vi "DL-SMART-MS-Modify-06-23-7.0.vi"() -> ()   [LabVIEW 2013]
uses:
  <userlib>/caLab/Private/Put_DBL-1D_PV.vi
  <resource>/objmgr/imaqdx.rc
  <vilib>/Utility/file.llb/Write To Spreadsheet File (DBL).vi
  <userlib>/caLab/Private/Put_I32_PV.vi
  <userlib>/caLab/Private/Get_PV.vi
  <vilib>/Analysis/NI_AALPro.lvlib
  cal_p.vi
  <userlib>/caLab/Private/CaLabEvent_PV-1D.vi
  <vilib>/Utility/file.llb/Read From Spreadsheet File (DBL).vi
  <vilib>/Utility/config.llb/NI_LVConfig.lvlib
  <vilib>/Utility/config.llb/Write Key (Double).vi
  <vilib>/Utility/config.llb/Read Key (Double).vi
  <vilib>/Utility/config.llb/Write Key (U32).vi
  <vilib>/Utility/config.llb/Read Key (U32).vi
  <vilib>/Utility/config.llb/Write Key (String).vi
  <vilib>/Utility/config.llb/Read Key (String).vi
  <vilib>/Utility/config.llb/Config Data RefNum.ctl
panel:
  out "targetMark":string
  out "config":T1 caption="引用句柄"
  in  "stop":bool=TRUE
  out "LaserEnergy uJ 2":dbl
  out "idn status":string
  out "MS":cluster{dbl[], "filtered data":dbl[]}(graph)
  out "std sample":T2(array[cluster])
  out "Image":T3(plugin-control)
  out "selected id":i32
  out "selected row":i32
  out "currentNO":string
  out "commet":string
  out "sampleID":string
  in  "Shots/Point":i32=100
  in  "chamber in":bool caption="TakeMS"
  in  "chamber out":bool caption="TakeMS"
  in  "Laser parameter":T5
  in  "ADC parameter":T6
  in  "ShutDownSystem":bool
  in  "ADC reference":refnum<vi>
  in  "SetLaserTransmission":dbl(slide) min=0.0 max=50.0 scale=0.0..20.0
  in  "LaserHV":u8=50 min=1 max=100
  in  "频率/Hz":u8=30
  out "Pul.HV-Real":dbl
  out "Identify Spcetrum":cluster{"ID1:X":dbl[], "ID1:Y":dbl[]}[](graph)
  in  "测试记录":i32(listbox)=6
  in  "Identification Results (单靶鉴定结果)":i32(listbox)=2
  in  "HVEnable":bool
  out "GateClose":bool
  out "LaserOK":bool
  out "HV-OK":bool
  out "Vacuum-OK":bool
  in  "Tab Control":T7(tab)
  in  "helix-Zeta-Step":dbl=100.0
  in  "helix-b":dbl=0.2
  in  "AcquireMS-Methods":u8(ring) items=["SinglePoint", "Multipoints", "MultiTar"]
  in  "Thresh":dbl=-0.005 format="%#_13g"
  in  "right rank":i32=2
  in  "left rank":i32=2
  in  "deBaseline":bool
  in  "MCPHV-Set":dbl=1400.0 min=0.0 max=1600.0
  in  "LensHV-Set":dbl=8000.0 min=0.0 max=10000.0
  in  "Tar.HV-Set":dbl=18010.0 min=0.0 max=20000.0
  in  "Pul.HV-Set":dbl=1400.0 min=0.0 max=2000.0
  in  "PulseDelay":dbl
  in  "ADCFreq":dbl
  in  "CH1_Coupling":u64(ring)=2 items=["Volt DC"=1, "Volt AC"=2, "Ampere DC"=4, "Ampere AC"=8, "Ohm"=16]
  in  "Channel 1_Range":dbl(ring)=4.0 items=["80 V"=80.0, "40 V"=40.0, "20 V"=20.0, "8 V"=8.0, "4 V"=4.0, "2 V"=2.0, "800 mV"=0.8, "400 mV"=0.4, "200 mV"=0.2]
  in  "Anal. Setting File":string="High Mass"
  in  "SettingFileSave":bool caption="TakeMS"
  in  "SettingFileAppl":bool caption="TakeMS"
  in  "SettingDel":bool caption="TakeMS"
  in  "RunADC":bool caption="TakeMS"
  out "ADCstatus":bool
  in  "Vac_Prot.":bool
  in  "Turbo_Fore":bool
  in  "Main_Samp":bool
  in  "Samp_Atmos":bool
  in  "Fore_Samp":bool
  in  "StartPump":bool
  in  "SopPump":bool
  out "TurboSpeed":dbl(knob) scale=0.0..100.0
  out "PumpKW":dbl
  out "PumpAmps":dbl
  out "PumpTemp":u16
  out "PumpVolts":dbl
  in  "laser OFF":bool
  in  "laser ON":bool
  out "cluster":T8
  in  "laser Deactive":bool
  out "A1-position-Y":dbl=45.0 caption="Y" min=0.0 max=55.0
  out "A1-position-X":dbl=53.4 caption="X" min=0.0 max=55.0
  in  "GO":bool
  in  "Y":dbl min=0.0 max=55.0
  in  "X":dbl min=0.0 max=55.0
  in  "A1-Position":bool caption="X-"
  in  "Plat_To_Zero":bool caption="TakeMS"
  in  "Plat_Cal":bool caption="TakeMS"
  out "Y当前":dbl
  out "X当前":dbl
  out "移动":bool
  out "Y满":bool
  out "Y标":bool
  out "X满":bool
  out "Y0":bool
  out "X0":bool
  out "靶位In/Out":bool
  out "仓门":bool
  out "Y过热":bool
  out "X过热":bool
  out "通讯":bool
  in  "Operation Record":i32(listbox)
  in  "OptionRecordLoad 2":bool caption="TakeMS"
  in  "OptionRecordClear":bool caption="TakeMS"
  out "c:":dbl
  out "b:":dbl
  out "a:":dbl
  in  "cancel cal":bool
  in  "cal save":bool
  in  "peak cal":bool
  in  "peak detect":bool
  in  "标准样品":u16(ring) items=["肺炎克雷伯菌", "铜绿假单胞菌"]
  in  "定标参数":i32(listbox)
  out "Tar.HV-Real":dbl
  out "LensHV-Real":dbl
  out "MCPHV-Real":dbl
  out "Lvaccum":dbl=0.83 format="%#_2e"
  out "Hvaccum":dbl=3.4e-05 format="%#_2e"
  in  "H12":bool
  in  "G12":bool
  in  "F12":bool
  in  "E12":bool
  in  "D12":bool
  in  "C12":bool
  in  "B12":bool
  in  "A12":bool
  in  "H11":bool
  in  "G11":bool
  in  "F11":bool
  in  "E11":bool
  in  "D11":bool
  in  "C11":bool
  in  "B11":bool
  in  "A11":bool
  in  "H10":bool
  in  "G10":bool
  in  "F10":bool
  in  "E10":bool
  in  "D10":bool
  in  "C10":bool
  in  "B10":bool
  in  "A10":bool
  in  "H9":bool
  in  "G9":bool
  in  "F9":bool
  in  "E9":bool
  in  "D9":bool
  in  "C9":bool
  in  "B9":bool
  in  "A9":bool
  in  "H8":bool
  in  "G8":bool
  in  "F8":bool
  in  "E8":bool
  in  "D8":bool
  in  "C8":bool
  in  "B8":bool
  in  "A8":bool
  in  "H7":bool
  in  "G7":bool
  in  "F7":bool
  in  "E7":bool
  in  "D7":bool
  in  "C7":bool
  in  "B7":bool
  in  "A7":bool
  in  "H6":bool
  in  "G6":bool
  in  "F6":bool
  in  "E6":bool
  in  "D6":bool
  in  "C6":bool
  in  "B6":bool
  in  "A6":bool
  in  "H5":bool
  in  "G5":bool
  in  "F5":bool
  in  "E5":bool
  in  "D5":bool
  in  "C5":bool
  in  "B5":bool
  in  "A5":bool
  in  "H4":bool
  in  "G4":bool
  in  "F4":bool
  in  "E4":bool
  in  "D4":bool
  in  "C4":bool
  in  "B4":bool
  in  "A4":bool
  in  "H3":bool
  in  "G3":bool
  in  "F3":bool
  in  "E3":bool
  in  "D3":bool
  in  "C3":bool
  in  "B3":bool
  in  "A3":bool
  in  "H2":bool
  in  "G2":bool
  in  "F2":bool
  in  "E2":bool
  in  "D2":bool
  in  "C2":bool
  in  "B2":bool
  in  "A2":bool
  in  "H1":bool
  in  "G1":bool
  in  "F1":bool
  in  "E1":bool
  in  "D1":bool
  in  "C1":bool
  in  "B1":bool
  in  "A1":bool
  in  "Clear":bool caption="TakeMS"
  in  "Add":bool caption="TakeMS"
  in  "TakeMS-Stop":bool caption="TakeMS"
  in  "TakeMS-Run":bool caption="TakeMS"
  # "Laser (激光)"
  # "光栅"
  # "uJ"
  # "Acq.(采谱)"
  # "Vacuum(真空)"
  # "1"
  # "2"
  # "3"
  # "4"
  # "5"
  # "6"
  # "7"
  # "8"
  # "9"
  # "10"
  # "11"
  # "12"
  # "A"
  # "Pa"
  # "High"
  # "B"
  # "Low"
  # "Pa"
  # "C"
  # "H.V.(高压)"
  # "D"
  # "MCP"
  # "V"
  # "E"
  # "Tar."
  # "V"
  # "F"
  # "Pul."
  # "V"
  # "G"
  # "Lens"
  # "V"
  # "H"
  # "Vauum (真空)"
  # "H.V. (高压)"
  # "Laser (激光)"
  # "Gate (仓门)"
  # "mm"
  # "Radian"
  # "H.V. (高压参数)"
  # "ADC(采集卡设置)"
  # "ADCFreq(采样)"
  # "MCP (探测器)"
  # "V"
  # "Hz"
  # "Tar. (靶)"
  # "V"
  # "Setting File(设置文件)"
  # "Coupling"
  # "Pulse (脉冲)"
  # "V"
  # "IntRange"
  # "V"
  # "Lens (透镜)"
  # "Delay (延时)"
  # "ns"
  # "Sole. Valves"
  # "Turbo Pump"
  # "自锁保护"
  # "机械/分子"
  # "主仓/样仓"
  # "样仓/大气"
  # "机械/样仓"
  # "激光器状态"
  # "mm"
  # "mm"
  # "mm"
  # "mm"
  # "mm"
  # "mm"
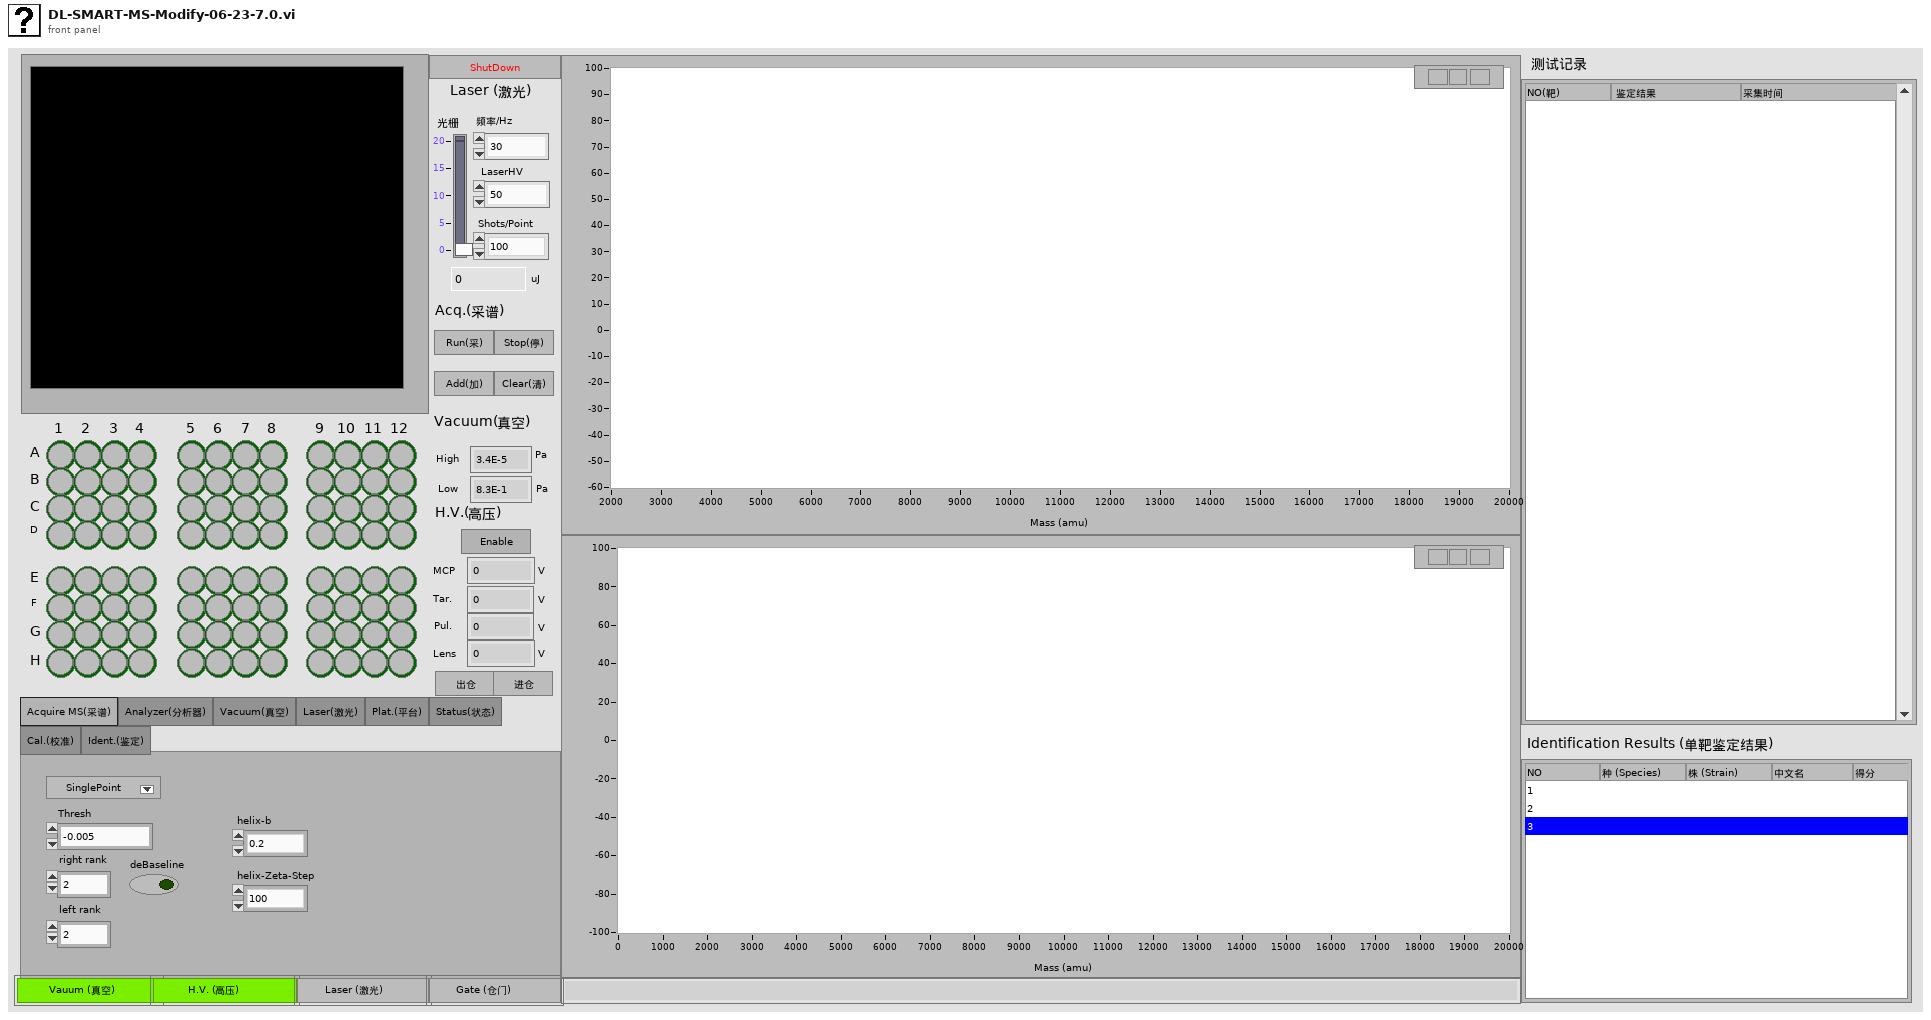
[diagram p1: front panel]
types:
  T1 = typedef "NI_LVConfig.lvlib/Config Data RefNum.ctl" = refnum<k1>
  T2 = cluster{"name":string, "mz":dbl[], "time":dbl[]}[]
  T3 = typedef "IMAQ Image.ctl" = refnum<image>
  T4 = typedef "Semaphore RefNum" = refnum<k1>
  T5 = cluster{"VISA resource name":refnum<visa-resource-name>, "standby":bool, "semaphore in":T4, "SetLaserEnergy":dbl}
  T6 = cluster{"TpDeviceHandle_t":u32, "Record Length/Samples":u64, "ShotsPerPoint":u16}
  T7 = enum32{"Acquire MS(采谱)", "Analyzer(分析器)", "Vacuum(真空)", "Laser(激光)", "Plat.(平台)", "Status(状态)", "Cal.(校准)", "Ident.(鉴定)"}
  T8 = cluster{"链接":bool, "待机":bool, "发射":bool, "[3]":bool, "内存":bool, "测能":bool, "温警":bool, "静态":bool, "操作":bool}
  T9 = cluster{"tag1":string, "tag2":string, "x":dbl[], "y":dbl[], "ID1:X":dbl[], "ID1:Y":dbl[], "ID1:REF:X":dbl[], "ID1:REF:Y":dbl[], "ID2:X":dbl[], "ID2:Y":dbl[], "ID2:REF:X":dbl[], "ID2:REF:Y":dbl[], "ID3:X":dbl[], "ID3:Y":dbl[], "ID3:REF:X":dbl[], "ID3:REF:Y":dbl[], "ID1:TAG1":string, "ID1:TAG2":string, "ID2:TAG1":string, "ID2:TAG2":string, "ID3:TAG1":string, "ID3:TAG2":string, "ID1:NAME":string, "ID2:NAME":string, "ID3:NAME":string, "ID1:SCORE":string, "ID2:SCORE":string, "ID3:SCORE":string, "NO":string}[]
  T10 = cluster{"laser semaphore":T4, "pump semaphore":T4}
  T11 = enum8{"Enabled", "Disabled", "Disabled and Grayed Out"}
  T12 = cluster{"tag1":string, "tag2":string, "x":dbl[], "y":dbl[], "ID1:X":dbl[], "ID1:Y":dbl[], "ID1:REF:X":dbl[], "ID1:REF:Y":dbl[], "ID2:X":dbl[], "ID2:Y":dbl[], "ID2:REF:X":dbl[], "ID2:REF:Y":dbl[], "ID3:X":dbl[], "ID3:Y":dbl[], "ID3:REF:X":dbl[], "ID3:REF:Y":dbl[], "ID1:TAG1":string, "ID1:TAG2":string, "ID2:TAG1":string, "ID2:TAG2":string, "ID3:TAG1":string, "ID3:TAG2":string, "ID1:NAME":string, "ID2:NAME":string, "ID3:NAME":string, "ID1:SCORE":string, "ID2:SCORE":string, "ID3:SCORE":string, "NO":string}
  T13 = cluster{"monitor":refnum<user-event>, "motor status":refnum<user-event>, "motor":refnum<user-event>, "notifier out":refnum<notifier>, "queue out":refnum<queue>, "AI":T4, "DI":T4, "CX":T4, "CY":T4}
  T14 = cluster{"AI Task":refnum<k21>, "AO Task":refnum<k21>, "DO Task":refnum<k21>, "DI Task":refnum<k21>, "PWM x":refnum<k21>, "PWM y":refnum<k21>, "counter x":refnum<k21>, "counter y":refnum<k21>}
  T15 = cluster{"tasks":cluster{"AI Task":refnum<k21>, "AO Task":refnum<k21>, "DO Task":refnum<k21>, "DI Task":refnum<k21>, "PWM x":refnum<k21>, "PWM y":refnum<k21>, "counter x":refnum<k21>, "counter y":refnum<k21>}, "interface":cluster{"monitor":refnum<user-event>, "motor status":refnum<user-event>, "motor":refnum<user-event>, "notifier out":refnum<notifier>, "queue out":refnum<queue>, "AI":T4, "DI":T4, "CX":T4, "CY":T4}, "error out":errorcluster}
  T16 = cluster{"ConfiguredPumpCom":refnum<visa-resource-name>, "ConfiguredLaserCom":refnum<visa-resource-name>}
  T17 = typedef "LVPoint32TypeDef.ctl" = cluster{"Horizontal":i32, "Vertical":i32}
  T18 = typedef "LVRowAndColumnTypeDef.ctl" = cluster{"Row":i32, "Column":i32}
  T19 = cluster{"Type":u32, "Version":u32, "Flags":u32, "SerialNumberHigh":u32, "SerialNumberLow":u32, "BusType":u32, "InterfaceName":string, "VendorName":string, "ModelName":string, "CameraFileName":string, "CameraAttributeURL":string}[]
  T20 = cluster{"Type":u32, "Version":u32, "Flags":u32, "SerialNumberHigh":u32, "SerialNumberLow":u32, "BusType":u32, "InterfaceName":string, "VendorName":string, "ModelName":string, "CameraFileName":string, "CameraAttributeURL":string}
  T21 = typedef "IMAQdx.ctl" = refnum<k21>
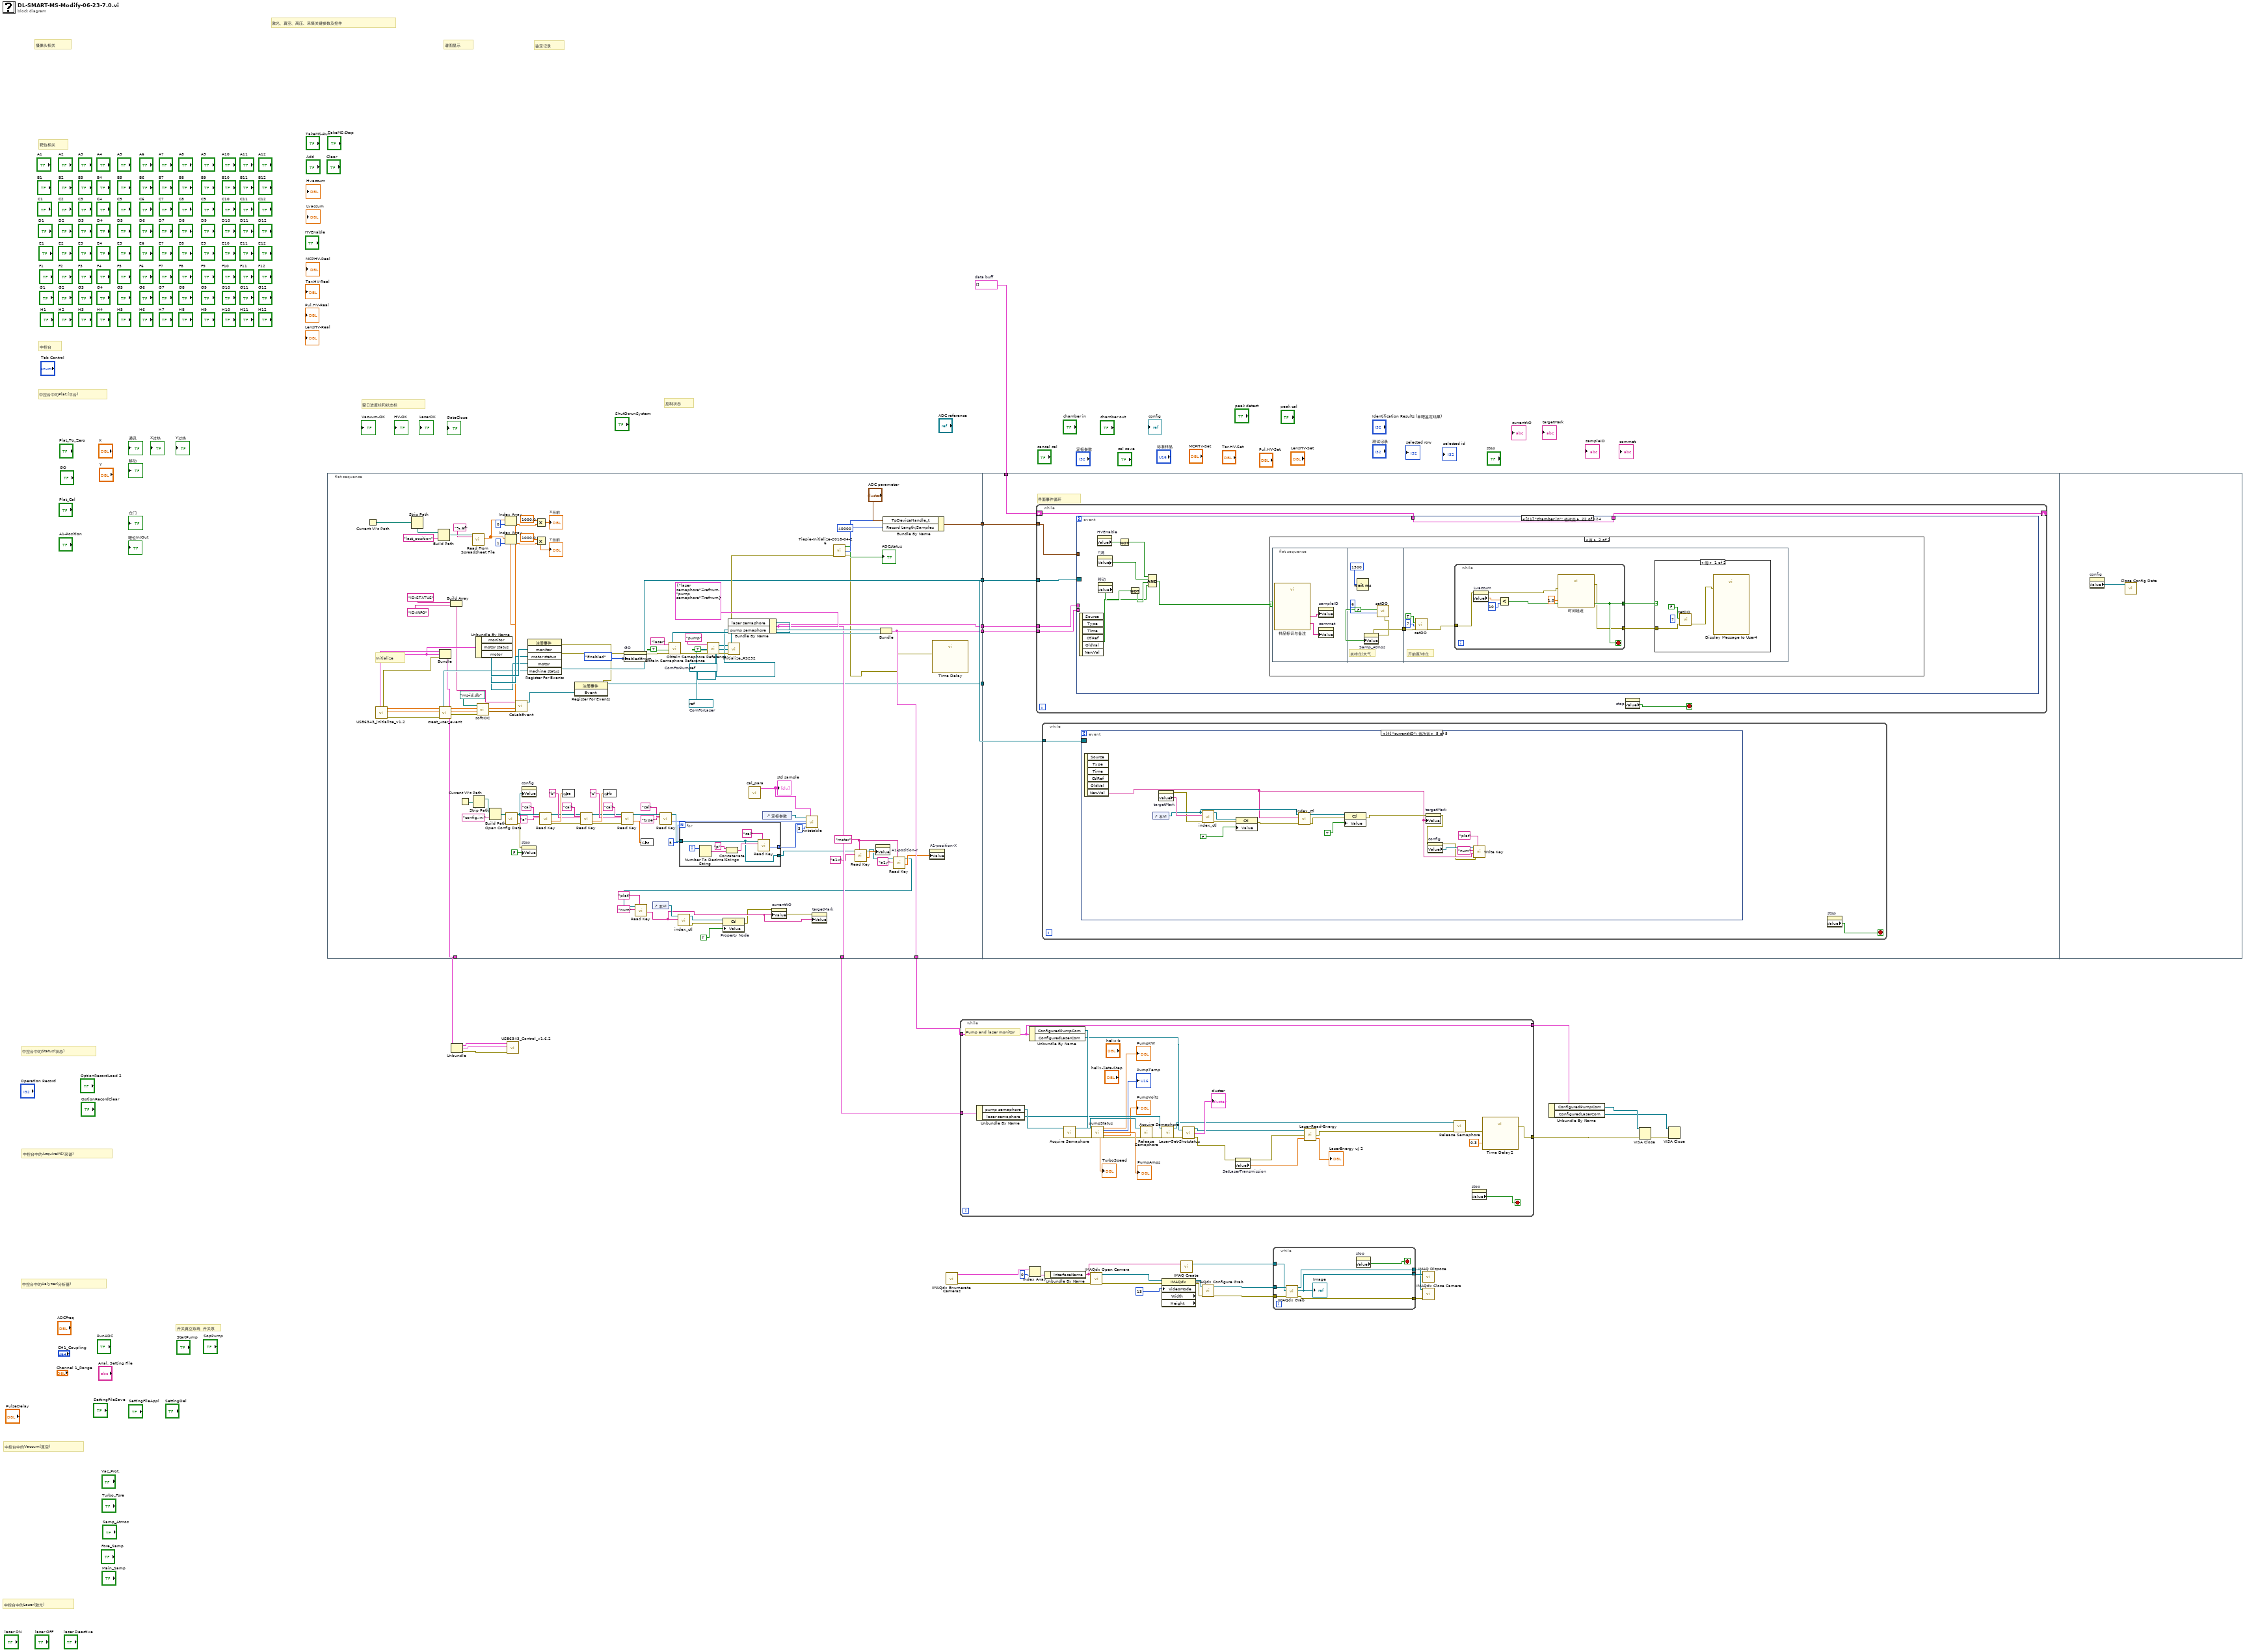
[diagram p0: block diagram]
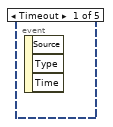
[diagram p2: hidden frame]
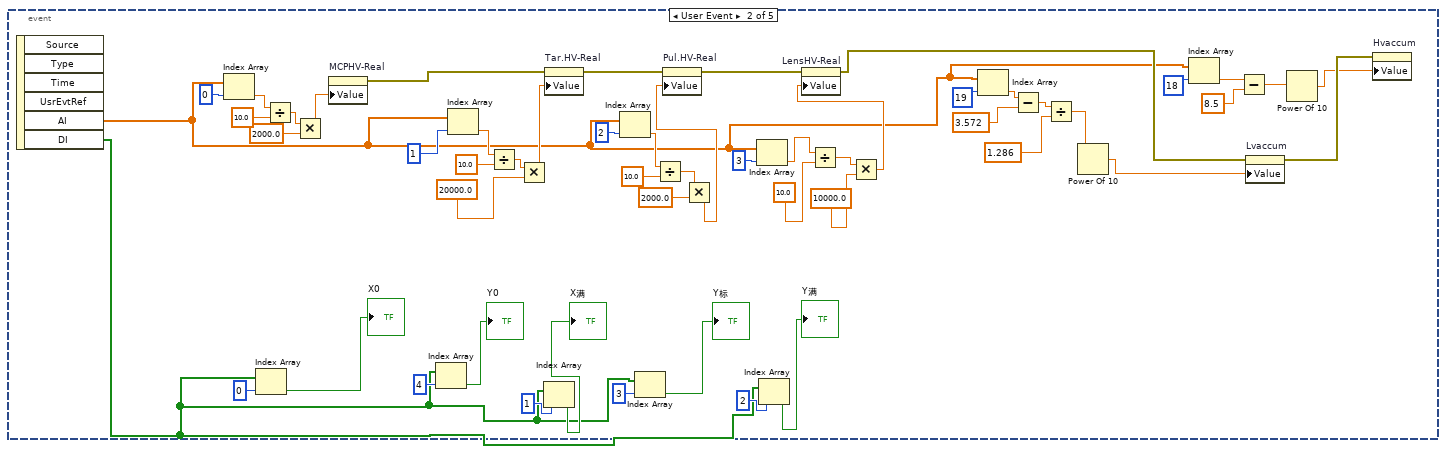
[diagram p3: hidden frame]
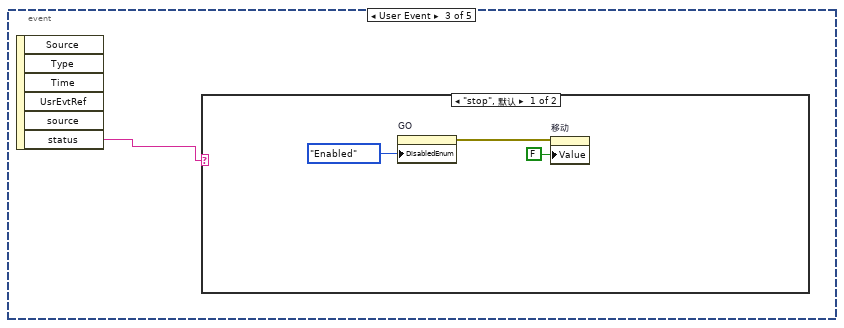
[diagram p4: hidden frame]
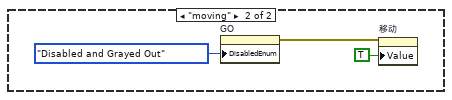
[diagram p5: hidden frame]
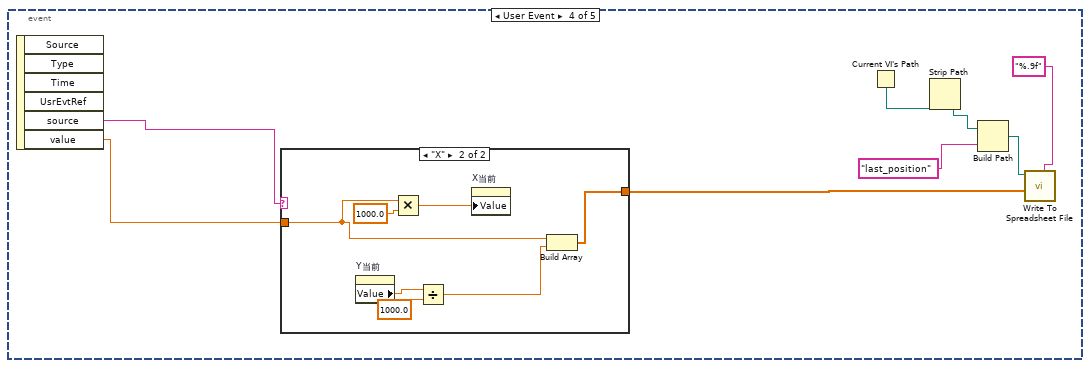
[diagram p6: hidden frame]
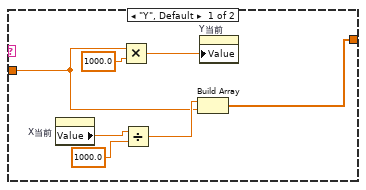
[diagram p7: hidden frame]
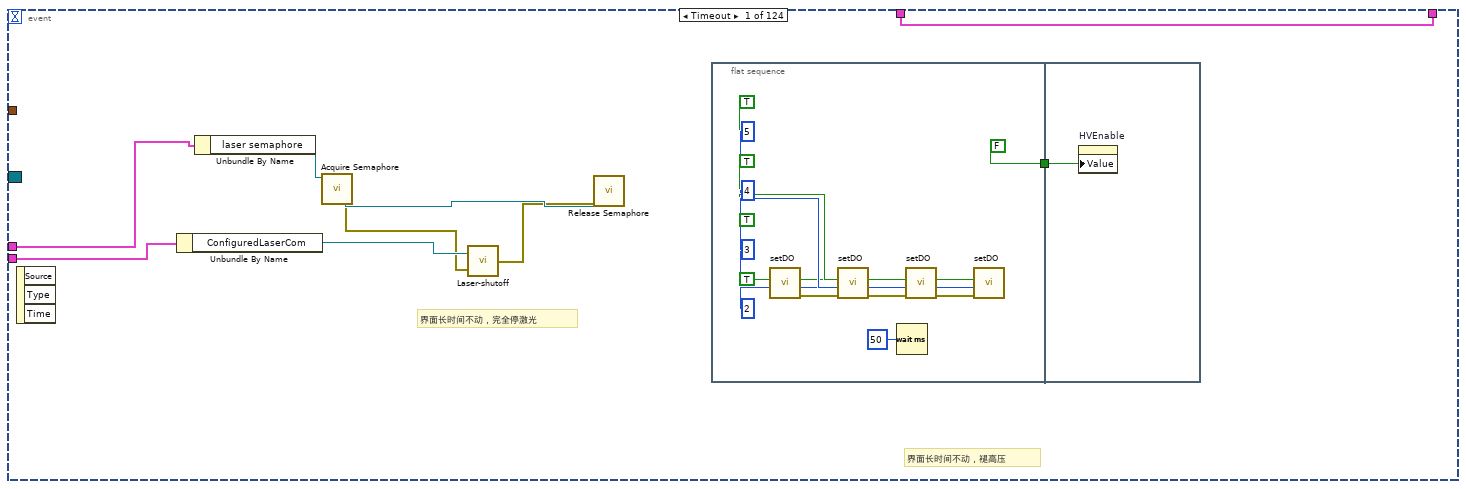
[diagram p8: hidden frame]
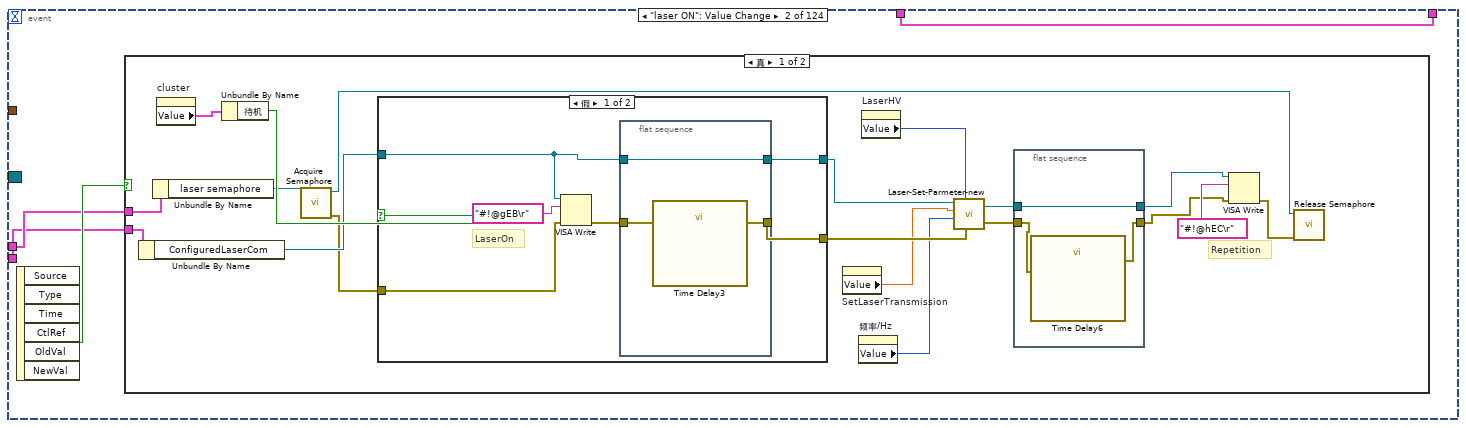
[diagram p9: hidden frame]
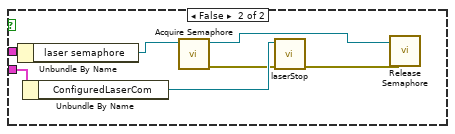
[diagram p11: hidden frame]
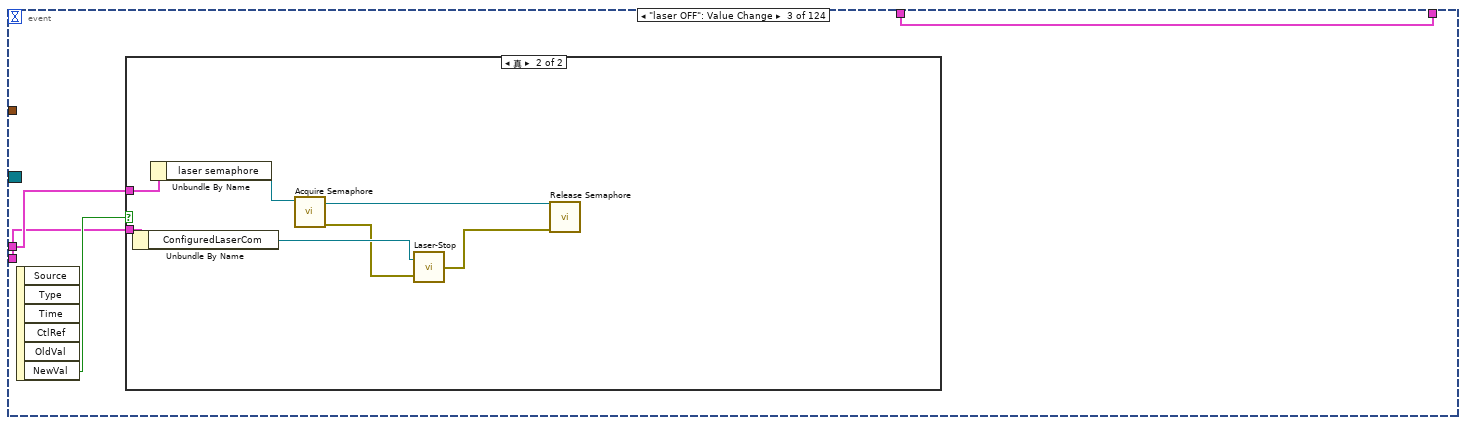
[diagram p12: hidden frame]
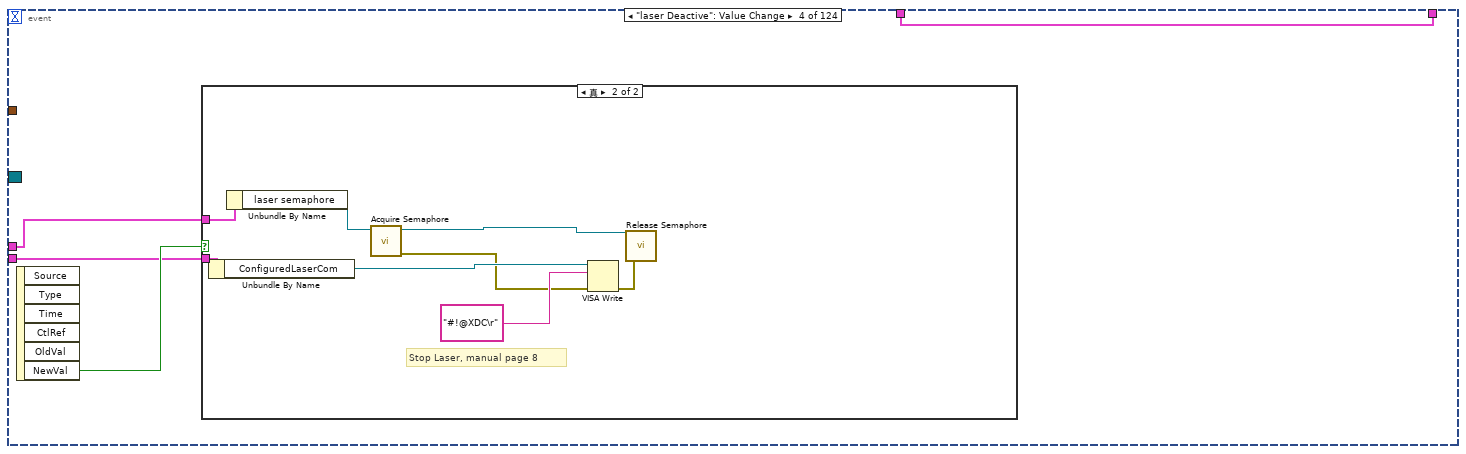
[diagram p14: hidden frame]
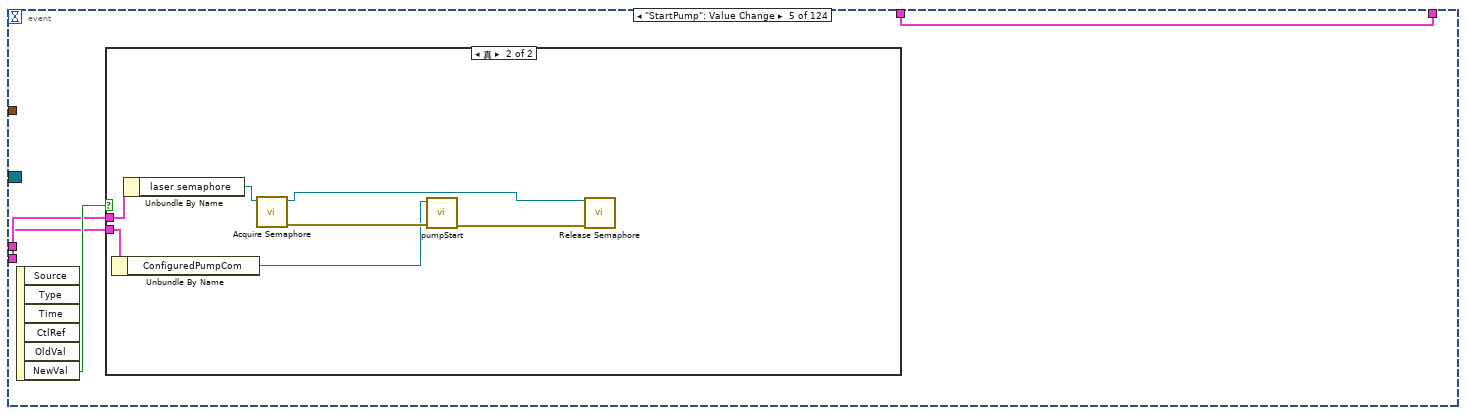
[diagram p16: hidden frame]
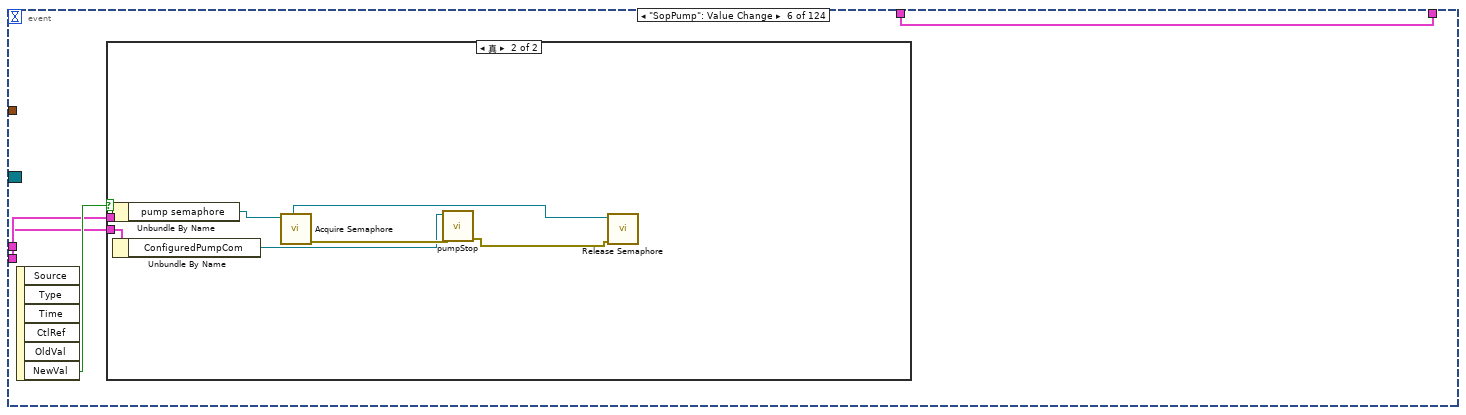
[diagram p18: hidden frame]
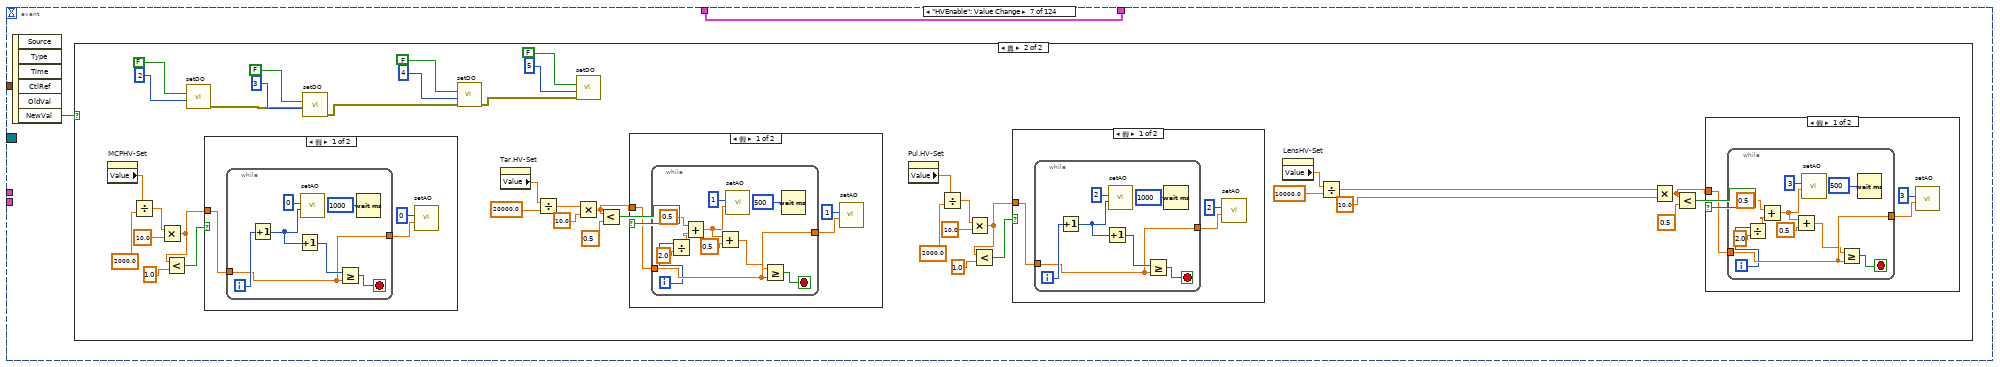
[diagram p20: hidden frame]
diagram:
  w26 = T9 []  # data buff
  # "Pump and laser monitor"
  # "开关真空系统  开关泵"
  # "控制状态"
  # "鉴定记录"
  # "谱图显示"
  # "激光、真空、高压、采集关键参数及控件"
  # "窗口进度栏和状态栏"
  # "中控台中的Laser(激光)"
  # "中控台中的Vaccum(真空)"
  # "中控台中的Aalyzer(分析器)"
  # "中控台中的AcquireMS(采谱)"
  # "中控台中的Status(状态)"
  # "中控台中的Plat.(平台)"
  # "中控台"
  # "靶位相关"
  # "摄像头相关"
  n1 = flat-sequence {
    tunnel: [w91] -> w33
    tunnel: [w116] -> w32
    tunnel: [w116] -> w30
    tunnel: [w115] -> w31
    tunnel: [w115] -> w29
    tunnel: [w119] -> w28
    tunnel: [w108] -> w27
    tunnel: [w79] -> w6
    tunnel: w33 -> [w146]
    tunnel: w32 -> [w150]
    tunnel: w31 -> [w149]
    tunnel: w27 -> [w148]
    tunnel: w26 -> [w147]
    tunnel: w6 -> [w145]
    frame #0 {
      w46 = "motor" ("section")
      w113 = refnum<visa-resource-name> "COM9"  # ComForLaser
      w114 = refnum<visa-resource-name> "COM10"  # ComForPump
      # "Initialize"
      n2 = Current VI's Path() -> (path=w106:path)
      n3 = Strip Path(path=w106) -> (stripped path=w105:path)  [unwired: 1 out]
      n4 = Build Path(base path=w105, name or relative path="last_position") -> (appended path=w103:path)
      n5 = Build Array("ID:STATUS", "ID:INFO") -> (w81:string[])
      n6 = Current VI's Path() -> (path=w76:path)
      n7 = call-poly <vilib>:"Read From Spreadsheet File.vi"("format (%.3f)"="%.6f", "file path (dialog if empty)"=w103) -> ("first row"=w101:dbl[])  [unwired: 5 in, 4 out]
      n8 = Strip Path(path=w76) -> (stripped path=w75:path)  [unwired: 1 out]
      n9 = Build Path(base path=w75, name or relative path="config.ini" ("名称或相对路径")) -> (appended path=w73:path)
      n10 = Index Array(array=w101, index=0) -> (element=w98:dbl)
      n11 = Index Array(array=w101, index=1) -> (element=w95:dbl)
      n12 = call "USB6343_initialize_v1.2.vi"("Y initial position"=w95, "X initial position"=w98) -> ("error out"=w120:errorcluster, "interface"=w121:T13, "tasks"=w122:T14)  [unwired: 7 in]
      n13 = Bundle("tasks"=w122, "interface"=w121, "error out"=w120) -> (w119:T15)  [unwired: 1 in]
      n14 = call "creat_user_event.vi"("error in (no error)"=w120) -> ("error out"=w88:errorcluster, "machine status"=w130:refnum<user-event>)  [unwired: 9 in]
      n15 = Unbundle By Name(w121) -> ("monitor"=w137:refnum<user-event>, "motor status"=w136:refnum<user-event>, "motor"=w135:refnum<user-event>)
      n16 = call "softIOC.vi"("error in (no error)"=w88, "路径"=path "ms-id.db") -> ("error out"=w89:errorcluster)  [unwired: 8 in, 1 out]
      n17 = call <vilib>:"Open Config Data.vi"("configuration file path"=w73) -> ("error out"=w72:errorcluster, "refnum"=w71:T1)  [unwired: 8 in, 1 out]
      n18 = call-poly <userlib>:"CaLabEvent.vi"("error in (no error)"=w89, "PV Names"=w81) -> ("Event"=w80:refnum<user-event>)  [unwired: 7 in, 2 out]
      n19 = property on="config" class="TypRef (严格)"("Value"=w71) -> ()  [unwired: 2 in, 2 out]
      n20 = property on="stop" class="Bool (严格)"(error in=w72, "Value"=FALSE ("ShutDownSystem")) -> ()  [unwired: 1 in, 2 out]
      n21 = Multiply(x=1000.0, y=w98) -> (x*y=→"X当前":dbl)
      n22 = Multiply(x=1000.0, y=w95) -> (x*y=→"Y当前":dbl)
      n23 = call-poly <vilib>:"Read Key.vi"("section"="cal", "key"="a", "refnum"=w71) -> ("error out"=w63:errorcluster, "value"=w68:dbl, "refnum out"=w64:T1)  [unwired: 5 in, 1 out]
      n24 = global write "cal_p.vi" "a"(w68) -> ()
      n25 = register-events(w80) -> (reference out=w79:refnum<event-registration>, error out=w78:errorcluster)  [unwired: 2 in]
      n26 = register-events(error in=w78, w137, w136, w135, w130) -> (reference out=w91:refnum<event-registration>, error out=w87:errorcluster)  [unwired: 1 in]
      n27 = call-poly <vilib>:"Read Key.vi"("section"="cal", "error in (no error)"=w63, "key"="b", "refnum"=w64) -> ("error out"=w59:errorcluster, "value"=w65:dbl, "refnum out"=w58:T1)  [unwired: 4 in, 1 out]
      n28 = global write "cal_p.vi" "b"(w65) -> ()
      n29 = call-poly <vilib>:"Read Key.vi"("section"="cal", "error in (no error)"=w59, "key"="c", "refnum"=w58) -> ("value"=w60:dbl, "refnum out"=w57:T1)  [unwired: 4 in, 2 out]
      n30 = property on="GO" class="Bool (严格)"(error in=w87, "DisabledEnum"=T11."Enabled" ("Disabled")) -> (error out=w131:errorcluster)  [unwired: 1 in, 1 out]
      n31 = global write "cal_p.vi" "c"(w60) -> ()
      n32 = control-ref of="本VI"() -> (w40:refnum<vi>)
      n33 = call-poly <vilib>:"Read Key.vi"("section"="cal", "key"="type", "refnum"=w57) -> ("value"=w54:u32, "refnum out"=w53:T1)  [unwired: 5 in, 2 out]
      n34 = call <vilib>:"Obtain Semaphore Reference.vi"("error in (no error)"=w131, "create if not found (T)"=TRUE, "name (unnamed)"="laser") -> ("error out"=w126:errorcluster, "semaphore"=w123:T4)  [unwired: 2 in, 1 out]
      n35 = for {
        N: 5 -> [_]
        tunnel: w53 -> [w138]
        tunnel: [w139] -> w51 mode=indexing
        tunnel: [w138] -> w50
        i -> [w143]
        n36 = Number To Decimal String(number=w143) -> (decimal integer string=w142:string)  [unwired: 1 in]
        n37 = Concatenate Strings("p", w142) -> (w140:string)
        n38 = call-poly <vilib>:"Read Key.vi"("section"="cal", "key"=w140, "refnum"=w138) -> ("value"=w139:u32)  [unwired: 5 in, 3 out]
      }
      n39 = call <vilib>:"Obtain Semaphore Reference.vi"("error in (no error)"=w126, "create if not found (T)"=TRUE, "name (unnamed)"="pump") -> ("error out"=w125:errorcluster, "semaphore"=w117:T4)  [unwired: 2 in, 1 out]
      n40 = Bundle By Name(cluster=T10 {"laser semaphore"=refnum, "pump semaphore"=refnum}, "laser semaphore"=w123, "pump semaphore"=w117) -> (w116:T10)
      n41 = call "Initialize_RS232.vi"("error in (no error)"=w125, "ComForLaser"=w113, "ComForPump"=w114) -> ("error out"=w112:errorcluster, "ConfiguredLaserCom"=w128:refnum<visa-resource-name>, "ConfiguredPumpCom"=w129:refnum<visa-resource-name>)
      n42 = call "cal_para.vi"() -> ("std sample"=w85:T2)  [unwired: 11 in]
      "std sample" <- w85
      n43 = control-ref of="定标参数"() -> (w86:refnum<vi>)
      n44 = call "writetable.vi"("std sample"=w85, "col"=3, "Array in"=w51, "type"=w54, "reference"=w86) -> ()  [unwired: 7 in]
      n45 = call "Tiepie-Initialize-2018-04-26.vi"("error in (no error)"=w112) -> ("error out"=w90:errorcluster, "TpDeviceHandle_t"=w110:u32, "Card-OK"=→"ADCstatus":bool)  [unwired: 3 in]
      n46 = call-poly <vilib>:"Read Key.vi"("section"=w46, "key"="a1x", "refnum"=w50) -> ("value"=w48:dbl, "refnum out"=w47:T1)  [unwired: 5 in, 2 out]
      n47 = property on="A1-position-Y" class="DigNum (严格)"("Value"=w48) -> ()  [unwired: 2 in, 2 out]
      n48 = Bundle("ConfiguredPumpCom"=w129, "ConfiguredLaserCom"=w128) -> (w115:T16)  [unwired: 1 in]
      n49 = Bundle By Name(cluster="ADC parameter", "TpDeviceHandle_t"=w110, "Record Length/Samples"=u64 40000) -> (w108:T6)
      n50 = call-poly <vilib>:"Read Key.vi"("section"=w46, "key"="a1y", "refnum"=w47) -> ("value"=w44:dbl, "refnum out"=w43:T1)  [unwired: 5 in, 2 out]
      n51 = call-poly <vilib>:"Read Key.vi"("section"="plat", "key"="num", "refnum"=w43) -> ("value"=w35:string)  [unwired: 5 in, 3 out]
      n52 = call "index_ctl.vi"("lable"=w35, "VI refence"=w40) -> ("error out"=w39:errorcluster, "Ctl refence"=w38:refnum<vi>)  [unwired: 8 in]
      n53 = property on="Property Node" class="Ctl"(reference=w38, error in=w39, "Value"=TRUE) -> (error out=w34:errorcluster)  [unwired: 1 out]
      n54 = property on="currentNO" class="Str"(error in=w34, "Value"=w35) -> (error out=w36:errorcluster)  [unwired: 1 in, 1 out]
      n55 = property on="targetMark" class="Str"(error in=w36, "Value"=w35) -> ()  [unwired: 1 in, 2 out]
      n56 = property on="A1-position-X" class="DigNum (严格)"("Value"=w44) -> ()  [unwired: 2 in, 2 out]
      n57 = call "Time Delay"("error in (no error)"=w90) -> ()  [unwired: 10 in, 1 out]
    }
    frame #1 {
      # "界面事件循环"
      n58 = while {
        tunnel: w145 -> [w258]
        tunnel: w149 -> [w257]
        tunnel: w150 -> [w256]
        tunnel: w148 -> [w255]
        shift-right: [w253] -> _
        shift-left: w147 -> [w254]
        stop <- w252 stop-if-true
        n59 = event shown="[21] \"chamber in\": 值改变" {
          selector: w258 -> [_ _ _ _ _ _ _ _ _ _ _ _ _ _ _ _ _ _ _ _ _ _ _ _ _ _ _ _ _ _ _ _ _ _ _ _ _ _ _ _ _ _ _ _ _ _ _ _ _ _ _ _ _ _ _ _ _ _ _ _ _ _ _ _ _ _ _ _ _ _ _ _ _ _ _ _ _ _ _ _ _ _ _ _ _ _ _ _ _ _ _ _ _ _ _ _ _ _ _ _ _ _ _ _ _ _ _ _ _ _ _ _ _ _ _ _ _ _ _ _ _ _ _ _]
          dyn-events: _ -> [_ _ _ _ _ _ _ _ _ _ _ _ _ _ _ _ _ _ _ _ _ _ _ _ _ _ _ _ _ _ _ _ _ _ _ _ _ _ _ _ _ _ _ _ _ _ _ _ _ _ _ _ _ _ _ _ _ _ _ _ _ _ _ _ _ _ _ _ _ _ _ _ _ _ _ _ _ _ _ _ _ _ _ _ _ _ _ _ _ _ _ _ _ _ _ _ _ _ _ _ _ _ _ _ _ _ _ _ _ _ _ _ _ _ _ _ _ _ _ _ _ _ _ _]
          timeout: _ -> [_ _ _ _ _ _ _ _ _ _ _ _ _ _ _ _ _ _ _ _ _ _ _ _ _ _ _ _ _ _ _ _ _ _ _ _ _ _ _ _ _ _ _ _ _ _ _ _ _ _ _ _ _ _ _ _ _ _ _ _ _ _ _ _ _ _ _ _ _ _ _ _ _ _ _ _ _ _ _ _ _ _ _ _ _ _ _ _ _ _ _ _ _ _ _ _ _ _ _ _ _ _ _ _ _ _ _ _ _ _ _ _ _ _ _ _ _ _ _ _ _ _ _ _]
          tunnel: w257 -> [w261 w283 w326 w337 w349 w360 _ _ _ _ _ _ _ _ w555 w614 _ _ _ _ _ _ _ _ _ _ _ _ _ _ _ _ _ _ _ _ _ _ _ _ _ _ _ _ _ _ _ _ _ _ _ _ _ _ _ _ _ _ _ _ _ _ _ _ _ _ _ _ _ _ _ _ _ _ _ _ _ _ _ _ _ _ _ _ _ _ _ _ _ _ _ _ _ _ _ _ _ _ _ _ _ _ _ _ _ _ _ _ _ _ _ _ _ _ _ _ _ _ _ _ _ _ _ w2697]
          tunnel: w256 -> [w262 w284 w327 w336 w350 w361 _ _ _ _ _ _ _ _ w556 w615 _ _ _ _ _ _ _ _ _ _ _ _ _ _ _ _ _ _ _ _ _ _ _ _ _ _ _ _ _ _ _ _ _ _ _ _ _ _ _ _ _ _ _ _ _ _ _ _ _ _ _ _ _ _ _ _ _ _ _ _ _ _ _ _ _ _ _ _ _ _ _ _ _ _ _ _ _ _ _ _ _ _ _ _ _ _ _ _ _ _ _ _ _ _ _ _ _ _ _ _ _ _ _ _ _ _ _ _]
          tunnel: w255 -> [_ _ _ _ _ _ _ _ _ _ _ _ _ _ w557 _ _ _ _ _ _ _ _ _ _ _ _ _ _ _ _ _ _ _ _ _ _ _ _ _ _ _ _ _ _ _ _ _ _ _ _ _ _ _ _ _ _ _ _ _ _ _ _ _ _ _ _ _ _ _ _ _ _ _ _ _ _ _ _ _ _ _ _ _ _ _ _ _ _ _ _ _ _ _ _ _ _ _ _ _ _ _ _ _ _ _ _ _ _ _ _ _ _ _ _ _ _ _ _ _ _ _ _ _]
          tunnel: w254 -> [w259 w282 w325 w339 w348 w359 w370 w478 w493 w508 w515 w522 w529 w538 w554 w616 w618 w648 w683 w722 w724 w731 w768 w806 w808 w858 w870 w886 w904 w921 w938 w955 w972 w991 w1016 w1033 w1050 w1067 w1084 w1101 w1120 w1139 w1158 w1177 w1196 w1215 w1234 w1253 w1272 w1291 w1310 w1329 w1348 w1367 w1386 w1405 w1424 w1443 w1462 w1481 w1500 w1519 w1538 w1557 w1576 w1595 w1614 w1633 w1652 w1671 w1694 w1713 w1732 w1751 w1770 w1789 w1808 w1827 w1846 w1865 w1884 w1903 w1922 w1941 w1960 w1979 w1998 w2017 w2036 w2055 w2074 w2093 w2112 w2131 w2150 w2169 w2188 w2207 w2226 w2245 w2264 w2283 w2302 w2321 w2340 w2359 w2378 w2397 w2416 w2435 w2454 w2473 w2492 w2511 w2530 w2549 w2568 w2587 w2606 w2625 w2644 w2663 w2682 w2696]
          tunnel: [w259 w282 w325 w339 w348 w359 w370 w478 w493 w508 w515 w522 w529 w538 w553 w616 w617 w648 w683 w722 w724 w731 w768 w806 w808 w858 w870 w886 w904 w921 w938 w955 w972 w990 w1016 w1033 w1050 w1067 w1084 w1101 w1120 w1139 w1158 w1177 w1196 w1215 w1234 w1253 w1272 w1291 w1310 w1329 w1348 w1367 w1386 w1405 w1424 w1443 w1462 w1481 w1500 w1519 w1538 w1557 w1576 w1595 w1614 w1633 w1652 w1671 w1694 w1713 w1732 w1751 w1770 w1789 w1808 w1827 w1846 w1865 w1884 w1903 w1922 w1941 w1960 w1979 w1998 w2017 w2036 w2055 w2074 w2093 w2112 w2131 w2150 w2169 w2188 w2207 w2226 w2245 w2264 w2283 w2302 w2321 w2340 w2359 w2378 w2397 w2416 w2435 w2454 w2473 w2492 w2511 w2530 w2549 w2568 w2587 w2606 w2625 w2644 w2663 w2682 w2696] -> w253
          event Timeout {
            # "界面长时间不动，褪高压"
            # "界面长时间不动，完全停激光"
            n60 = event-data() -> ()  [unwired: 1 in, 3 out]
            n61 = Unbundle By Name(w261) -> ("ConfiguredLaserCom"=w265:refnum<visa-resource-name>)
            n62 = Unbundle By Name(w262) -> ("laser semaphore"=w267:T4)
            n63 = call <vilib>:"Acquire Semaphore.vi"("semaphore"=w267) -> ("error out"=w264:errorcluster, "semaphore out"=w266:T4)  [unwired: 4 in, 1 out]
            n64 = call "Laser-shutoff.vi"("error in (no error)"=w264, "VISA resource name"=w265) -> ("error out"=w263:errorcluster)
            n65 = call <vilib>:"Release Semaphore.vi"("error in (no error)"=w263, "semaphore"=w266) -> ()  [unwired: 4 in, 2 out]
            n66 = flat-sequence {
              tunnel: [FALSE ("HVEnable")] -> w260
              tunnel: w260 -> [w281]
              frame #0 {
                n67 = call "setDO.vi"("channel"=2, "on/off"=TRUE) -> ("错误输出"=w278:errorcluster)  [unwired: 9 in]
                n68 = call "setDO.vi"("错误输入（无错误）"=w278, "channel"=3, "on/off"=TRUE) -> ("错误输出"=w279:errorcluster)  [unwired: 8 in]
                n69 = Wait (ms)(milliseconds to wait=u32 50) -> ()  [unwired: 1 out]
                n70 = call "setDO.vi"("错误输入（无错误）"=w279, "channel"=4, "on/off"=TRUE) -> ("错误输出"=w280:errorcluster)  [unwired: 8 in]
                n71 = call "setDO.vi"("错误输入（无错误）"=w280, "channel"=5, "on/off"=TRUE) -> ()  [unwired: 8 in, 1 out]
              }
              frame #1 {
                n72 = property on="HVEnable" class="Bool (严格)"("Value"=w281) -> ()  [unwired: 2 in, 2 out]
              }
            }
          }
          event "laser ON": Value Change {
            n73 = event-data() -> ("NewVal"=w285:bool)  [unwired: 1 in, 5 out]
            n74 = case shown="真" w285 {
              tunnel: w284 -> [w304 w324]
              tunnel: w283 -> [w303 w322]
              frame True {
                # "Repetition"
                n75 = Unbundle By Name(w303) -> ("ConfiguredLaserCom"=w300:refnum<visa-resource-name>)
                n76 = Unbundle By Name(w304) -> ("laser semaphore"=w297:T4)
                n77 = property on="cluster" class="Clust (严格)"() -> ("Value"=w302:T8)  [unwired: 2 in, 2 out]
                n78 = Unbundle By Name(w302) -> ("待机"=w301:bool)
                n79 = call <vilib>:"Acquire Semaphore.vi"("semaphore"=w297) -> ("error out"=w295:errorcluster, "semaphore out"=w296:T4)  [unwired: 4 in, 1 out]
                n80 = case shown="假" w301 {
                  tunnel: w300 -> [w312 w317]
                  tunnel: [w311 w317] -> w294
                  tunnel: [w309 w316] -> w293
                  tunnel: w295 -> [w308 w316]
                  frame False {
                    # "LaserOn"
                    n81 = VISA Write(VISA resource name=w312, write buffer="#!@gEB\r", error in (no error)=w308) -> (error out=w310:errorcluster)  [unwired: 2 out]
                    n82 = flat-sequence {
                      tunnel: w310 -> [w315]
                      tunnel: [w315] -> w309
                      tunnel: w312 -> [w314]
                      tunnel: [w314] -> w311
                      frame #0 {
                        n83 = call "Time Delay3"() -> ()  [unwired: 11 in, 1 out]
                      }
                    }
                  }
                  frame True {
                  }
                }
                n84 = property on="SetLaserTransmission" class="Slide (严格)"() -> ("Value"=w287:dbl)  [unwired: 2 in, 2 out]
                n85 = property on="频率/Hz" class="DigNum (严格)"() -> ("Value"=w286:u8)  [unwired: 2 in, 2 out]
                n86 = property on="LaserHV" class="DigNum (严格)"() -> ("Value"=w288:u8)  [unwired: 2 in, 2 out]
                n87 = call "Laser-Set-Parmeter-new.vi"("error in (no error)"=w293, "LaserHV"=w288, "LaserFreq"=w286, "SetTransmission"=w287, "VISA resource name"=w294) -> ("error out"=w290:errorcluster, "VISA resource name out"=w292:refnum<visa-resource-name>)  [unwired: 1 in]
                n88 = flat-sequence {
                  tunnel: w292 -> [w307]
                  tunnel: [w307] -> w291
                  tunnel: w290 -> [w306]
                  tunnel: [w305] -> w289
                  frame #0 {
                    n89 = call "Time Delay6"("error in (no error)"=w306) -> ("error out"=w305:errorcluster)  [unwired: 10 in]
                  }
                }
                n90 = VISA Write(VISA resource name=w291, write buffer="#!@hEC\r", error in (no error)=w289) -> (error out=w298:errorcluster)  [unwired: 2 out]
                n91 = call <vilib>:"Release Semaphore.vi"("error in (no error)"=w298, "semaphore"=w296) -> ()  [unwired: 4 in, 2 out]
              }
              frame False {
                n92 = Unbundle By Name(w324) -> ("laser semaphore"=w323:T4)
                n93 = Unbundle By Name(w322) -> ("ConfiguredLaserCom"=w321:refnum<visa-resource-name>)
                n94 = call <vilib>:"Acquire Semaphore.vi"("semaphore"=w323) -> ("error out"=w320:errorcluster, "semaphore out"=w318:T4)  [unwired: 4 in, 1 out]
                n95 = call "laserStop.vi"("error in (no error)"=w320, "VISA resource name"=w321) -> ("error out"=w319:errorcluster)  [unwired: 9 in]
                n96 = call <vilib>:"Release Semaphore.vi"("error in (no error)"=w319, "semaphore"=w318) -> ()  [unwired: 4 in, 2 out]
              }
            }
          }
          event "laser OFF": Value Change {
            n97 = event-data() -> ("NewVal"=w328:bool)  [unwired: 1 in, 5 out]
            n98 = case shown="真" w328 {
              tunnel: w327 -> [_ w335]
              tunnel: w326 -> [_ w333]
              frame False {
              }
              frame True {
                n99 = Unbundle By Name(w333) -> ("ConfiguredLaserCom"=w331:refnum<visa-resource-name>)
                n100 = Unbundle By Name(w335) -> ("laser semaphore"=w334:T4)
                n101 = call <vilib>:"Acquire Semaphore.vi"("semaphore"=w334) -> ("error out"=w330:errorcluster, "semaphore out"=w332:T4)  [unwired: 4 in, 1 out]
                n102 = call "Laser-Stop.vi"("error in (no error)"=w330, "VISA resource name"=w331) -> ("error out"=w329:errorcluster)
                n103 = call <vilib>:"Release Semaphore.vi"("error in (no error)"=w329, "semaphore"=w332) -> ()  [unwired: 4 in, 2 out]
              }
            }
          }
          event "laser Deactive": Value Change {
            n104 = event-data() -> ("NewVal"=w338:bool)  [unwired: 1 in, 5 out]
            n105 = case shown="真" w338 {
              tunnel: w336 -> [_ w347]
              tunnel: w337 -> [_ w345]
              frame False {
              }
              frame True {
                # "Stop Laser, manual page 8"
                n106 = Unbundle By Name(w345) -> ("ConfiguredLaserCom"=w342:refnum<visa-resource-name>)
                n107 = Unbundle By Name(w347) -> ("laser semaphore"=w346:T4)
                n108 = call <vilib>:"Acquire Semaphore.vi"("semaphore"=w346) -> ("error out"=w341:errorcluster, "semaphore out"=w344:T4)  [unwired: 4 in, 1 out]
                n109 = VISA Write(VISA resource name=w342, write buffer="#!@XDC\r", error in (no error)=w341) -> (error out=w340:errorcluster)  [unwired: 2 out]
                n110 = call <vilib>:"Release Semaphore.vi"("error in (no error)"=w340, "semaphore"=w344) -> ()  [unwired: 4 in, 2 out]
              }
            }
          }
          event "StartPump": Value Change {
            n111 = event-data() -> ("NewVal"=w351:bool)  [unwired: 1 in, 5 out]
            n112 = case shown="真" w351 {
              tunnel: w350 -> [_ w356]
              tunnel: w349 -> [_ w355]
              frame False {
              }
              frame True {
                n113 = Unbundle By Name(w355) -> ("ConfiguredPumpCom"=w354:refnum<visa-resource-name>)
                n114 = Unbundle By Name(w356) -> ("laser semaphore"=w353:T4)
                n115 = call <vilib>:"Acquire Semaphore.vi"("semaphore"=w353) -> ("error out"=w358:errorcluster, "semaphore out"=w352:T4)  [unwired: 4 in, 1 out]
                n116 = call "pumpStart.vi"("error in (no error)"=w358, "VISA resource name"=w354) -> ("error out"=w357:errorcluster)  [unwired: 9 in]
                n117 = call <vilib>:"Release Semaphore.vi"("error in (no error)"=w357, "semaphore"=w352) -> ()  [unwired: 4 in, 2 out]
              }
            }
          }
          event "SopPump": Value Change {
            n118 = event-data() -> ("NewVal"=w362:bool)  [unwired: 1 in, 5 out]
            n119 = case shown="真" w362 {
              tunnel: w361 -> [_ w366]
              tunnel: w360 -> [_ w364]
              frame False {
              }
              frame True {
                n120 = Unbundle By Name(w366) -> ("pump semaphore"=w365:T4)
                n121 = Unbundle By Name(w364) -> ("ConfiguredPumpCom"=w363:refnum<visa-resource-name>)
                n122 = call <vilib>:"Acquire Semaphore.vi"("semaphore"=w365) -> ("error out"=w369:errorcluster, "semaphore out"=w367:T4)  [unwired: 4 in, 1 out]
                n123 = call "pumpStop.vi"("error in (no error)"=w369, "VISA resource name"=w363) -> ("error out"=w368:errorcluster)  [unwired: 9 in]
                n124 = call <vilib>:"Release Semaphore.vi"("error in (no error)"=w368, "semaphore"=w367) -> ()  [unwired: 4 in, 2 out]
              }
            }
          }
          event "HVEnable": Value Change {
            n125 = event-data() -> ("NewVal"=w371:bool)  [unwired: 1 in, 5 out]
            n126 = case shown="真" w371 {
              frame False {
                n127 = call "setDO.vi"("channel"=2, "on/off"=TRUE) -> ("错误输出"=w374:errorcluster)  [unwired: 9 in]
                n128 = call "setDO.vi"("错误输入（无错误）"=w374, "channel"=3, "on/off"=TRUE) -> ("错误输出"=w373:errorcluster)  [unwired: 8 in]
                n129 = call "setDO.vi"("错误输入（无错误）"=w373, "channel"=4, "on/off"=TRUE) -> ("错误输出"=w372:errorcluster)  [unwired: 8 in]
                n130 = call "setDO.vi"("错误输入（无错误）"=w372, "channel"=5, "on/off"=TRUE) -> ()  [unwired: 8 in, 1 out]
              }
              frame True {
                n131 = property on="MCPHV-Set" class="DigNum (严格)"() -> ("Value"=w407:dbl)  [unwired: 2 in, 2 out]
                n132 = Divide(x=w407, y=2000.0) -> (x/y=w409:dbl)
                n133 = Multiply(x=w409, y=10.0) -> (x*y=w400:dbl)
                n134 = Less?(x=w400, y=1.0) -> (x < y?=w401:bool)
                n135 = call "setDO.vi"("channel"=2, "on/off"=FALSE) -> ("错误输出"=w413:errorcluster)  [unwired: 9 in]
                n136 = case shown="假" w401 {
                  tunnel: w400 -> [w468 w476]
                  frame False {
                    n137 = while {
                      tunnel: w468 -> [w470]
                      tunnel: [w470] -> w466
                      i -> [w474]
                      stop <- w471 stop-if-true
                      n138 = Increment(x=w474) -> (x+1=w473:i32)
                      n139 = Increment(x=w473) -> (x+1=w472:i32)
                      n140 = call "setAO.vi"("value"=w473, "channel"=0) -> ()  [unwired: 9 in, 1 out]
                      n141 = Greater Or Equal?(x=w472, y=w470) -> (x >= y?=w471:bool)
                      n142 = Wait (ms)(milliseconds to wait=1000) -> ()  [unwired: 1 out]
                    }
                    n143 = call "setAO.vi"("value"=w466, "channel"=0) -> ()  [unwired: 9 in, 1 out]
                  }
                  frame True {
                    n144 = call "setAO.vi"("value"=w476, "channel"=0) -> ()  [unwired: 9 in, 1 out]
                  }
                }
                n145 = call "setDO.vi"("错误输入（无错误）"=w413, "channel"=3, "on/off"=FALSE) -> ("错误输出"=w412:errorcluster)  [unwired: 8 in]
                n146 = call "setDO.vi"("错误输入（无错误）"=w412, "channel"=4, "on/off"=FALSE) -> ("错误输出"=w411:errorcluster)  [unwired: 8 in]
                n147 = property on="Tar.HV-Set" class="DigNum (严格)"() -> ("Value"=w403:dbl)  [unwired: 2 in, 2 out]
                n148 = Divide(x=w403, y=20000.0) -> (x/y=w405:dbl)
                n149 = call "setDO.vi"("错误输入（无错误）"=w411, "channel"=5, "on/off"=FALSE) -> ()  [unwired: 8 in, 1 out]
                n150 = Multiply(x=w405, y=10.0) -> (x*y=w397:dbl)
                n151 = Less?(x=w397, y=0.5) -> (x < y?=w398:bool)
                n152 = case shown="假" w398 {
                  tunnel: w397 -> [w452 w464]
                  frame False {
                    n153 = while {
                      tunnel: w452 -> [w461]
                      tunnel: [w461] -> w450
                      i -> [w457]
                      stop <- w462 stop-if-true
                      n154 = Divide(x=w457, y=2.0) -> (x/y=w458:dbl)
                      n155 = Add(x=0.5, y=w458) -> (x+y=w455:dbl)
                      n156 = Add(x=w455, y=0.5) -> (x+y=w453:dbl)
                      n157 = call "setAO.vi"("value"=w455, "channel"=1) -> ()  [unwired: 9 in, 1 out]
                      n158 = Greater Or Equal?(x=w453, y=w461) -> (x >= y?=w462:bool)
                      n159 = Wait (ms)(milliseconds to wait=500) -> ()  [unwired: 1 out]
                    }
                    n160 = call "setAO.vi"("value"=w450, "channel"=1) -> ()  [unwired: 9 in, 1 out]
                  }
                  frame True {
                    n161 = call "setAO.vi"("value"=w464, "channel"=1) -> ()  [unwired: 9 in, 1 out]
                  }
                }
                n162 = property on="Pul.HV-Set" class="DigNum (严格)"() -> ("Value"=w396:dbl)  [unwired: 2 in, 2 out]
                n163 = Divide(x=w396, y=2000.0) -> (x/y=w391:dbl)
                n164 = Multiply(x=w391, y=10.0) -> (x*y=w395:dbl)
                n165 = Less?(x=w395, y=1.0) -> (x < y?=w394:bool)
                n166 = case shown="假" w394 {
                  tunnel: w395 -> [w440 w448]
                  frame False {
                    n167 = while {
                      tunnel: w440 -> [w442]
                      tunnel: [w442] -> w438
                      i -> [w446]
                      stop <- w443 stop-if-true
                      n168 = Increment(x=w446) -> (x+1=w445:i32)
                      n169 = Increment(x=w445) -> (x+1=w444:i32)
                      n170 = call "setAO.vi"("value"=w445, "channel"=2) -> ()  [unwired: 9 in, 1 out]
                      n171 = Greater Or Equal?(x=w444, y=w442) -> (x >= y?=w443:bool)
                      n172 = Wait (ms)(milliseconds to wait=1000) -> ()  [unwired: 1 out]
                    }
                    n173 = call "setAO.vi"("value"=w438, "channel"=2) -> ()  [unwired: 9 in, 1 out]
                  }
                  frame True {
                    n174 = call "setAO.vi"("value"=w448, "channel"=2) -> ()  [unwired: 9 in, 1 out]
                  }
                }
                n175 = property on="LensHV-Set" class="DigNum (严格)"() -> ("Value"=w389:dbl)  [unwired: 2 in, 2 out]
                n176 = Divide(x=w389, y=10000.0) -> (x/y=w384:dbl)
                n177 = Multiply(x=w384, y=10.0) -> (x*y=w388:dbl)
                n178 = Less?(x=w388, y=0.5) -> (x < y?=w387:bool)
                n179 = case shown="假" w387 {
                  tunnel: w388 -> [w424 w436]
                  frame False {
                    n180 = while {
                      tunnel: w424 -> [w433]
                      tunnel: [w433] -> w422
                      i -> [w429]
                      stop <- w434 stop-if-true
                      n181 = Divide(x=w429, y=2.0) -> (x/y=w430:dbl)
                      n182 = Add(x=0.5, y=w430) -> (x+y=w427:dbl)
                      n183 = Add(x=w427, y=0.5) -> (x+y=w425:dbl)
                      n184 = call "setAO.vi"("value"=w427, "channel"=3) -> ()  [unwired: 9 in, 1 out]
                      n185 = Greater Or Equal?(x=w425, y=w433) -> (x >= y?=w434:bool)
                      n186 = Wait (ms)(milliseconds to wait=500) -> ()  [unwired: 1 out]
                    }
                    n187 = call "setAO.vi"("value"=w422, "channel"=3) -> ()  [unwired: 9 in, 1 out]
                  }
                  frame True {
                    n188 = call "setAO.vi"("value"=w436, "channel"=3) -> ()  [unwired: 9 in, 1 out]
                  }
                }
              }
            }
          }
          event "Samp_Atmos": Value Change {
            n189 = event-data() -> ("OldVal"=w479:bool, "NewVal"=w483:bool)  [unwired: 1 in, 4 out]
            n190 = property on="Fore_Samp" class="Bool (严格)"() -> ("Value"=w482:bool)  [unwired: 2 in, 2 out]
            n191 = And(x=w483, y=w482) -> (x .and. y?=w481:bool)
            n192 = Not(x=w481) -> (.not. x?=w480:bool)
            n193 = case shown="真" w480 {
              tunnel: w483 -> [_ w486]
              tunnel: w479 -> [w485 _]
              frame False {
                n194 = property on="Samp_Atmos" class="Bool (严格)"("Value"=w485) -> (error out=w484:errorcluster)  [unwired: 2 in, 1 out]
                n195 = call "Display Message to User7"("error in (no error)"=w484) -> ()  [unwired: 9 in, 2 out]
              }
              frame True {
                n196 = case shown="假" w486 {
                  frame False {
                    n197 = call "setDO.vi"("channel"=6, "on/off"=FALSE) -> ()  [unwired: 9 in, 1 out]
                  }
                  frame True {
                    n198 = property on="Y满" class="Bool (严格)"() -> ("Value"=w490:bool)  [unwired: 2 in, 2 out]
                    n199 = Not(x=w490) -> (.not. x?=w489:bool)
                    n200 = case shown="假" w489 {
                      frame False {
                        n201 = call "setDO.vi"("channel"=6, "on/off"=TRUE) -> ()  [unwired: 9 in, 1 out]
                      }
                      frame True {
                        n202 = call "Display Message to User6"() -> ()  [unwired: 10 in, 2 out]
                      }
                    }
                  }
                }
              }
            }
          }
          event "Fore_Samp": Value Change {
            n203 = event-data() -> ("OldVal"=w494:bool, "NewVal"=w498:bool)  [unwired: 1 in, 4 out]
            n204 = property on="Samp_Atmos" class="Bool (严格)"() -> ("Value"=w497:bool)  [unwired: 2 in, 2 out]
            n205 = And(x=w498, y=w497) -> (x .and. y?=w496:bool)
            n206 = Not(x=w496) -> (.not. x?=w495:bool)
            n207 = case shown="真" w495 {
              tunnel: w498 -> [_ w501]
              tunnel: w494 -> [w500 _]
              frame False {
                n208 = property on="Fore_Samp" class="Bool (严格)"("Value"=w500) -> (error out=w499:errorcluster)  [unwired: 2 in, 1 out]
                n209 = call "Display Message to User8"("error in (no error)"=w499) -> ()  [unwired: 9 in, 2 out]
              }
              frame True {
                n210 = case shown="真" w501 {
                  frame False {
                    n211 = call "setDO.vi"("channel"=7, "on/off"=FALSE) -> ()  [unwired: 9 in, 1 out]
                  }
                  frame True {
                    n212 = property on="Y满" class="Bool (严格)"() -> ("Value"=w505:bool)  [unwired: 2 in, 2 out]
                    n213 = Not(x=w505) -> (.not. x?=w504:bool)
                    n214 = case shown="真" w504 {
                      frame False {
                        n215 = call "setDO.vi"("channel"=7, "on/off"=TRUE) -> ()  [unwired: 9 in, 1 out]
                      }
                      frame True {
                        n216 = call "Display Message to User"() -> ()  [unwired: 10 in, 2 out]
                      }
                    }
                  }
                }
              }
            }
          }
          event "MCPHV-Set": Value Change {
            n217 = event-data() -> ("NewVal"=w509:dbl)  [unwired: 1 in, 5 out]
            n218 = Divide(x=w509, y=2000.0) -> (x/y=w512:dbl)
            n219 = Multiply(x=w512, y=10.0) -> (x*y=w510:dbl)
            n220 = call "setAO.vi"("value"=w510, "channel"=0) -> ()  [unwired: 9 in, 1 out]
          }
          event "Tar.HV-Set": Value Change {
            n221 = event-data() -> ("NewVal"=w521:dbl)  [unwired: 1 in, 5 out]
            n222 = Divide(x=w521, y=20000.0) -> (x/y=w518:dbl)
            n223 = Multiply(x=w518, y=10.0) -> (x*y=w516:dbl)
            n224 = call "setAO.vi"("value"=w516, "channel"=1) -> ()  [unwired: 9 in, 1 out]
          }
          event "Pul.HV-Set": Value Change {
            n225 = event-data() -> ("NewVal"=w528:dbl)  [unwired: 1 in, 5 out]
            n226 = Divide(x=w528, y=2000.0) -> (x/y=w525:dbl)
            n227 = Multiply(x=w525, y=10.0) -> (x*y=w523:dbl)
            n228 = call "setAO.vi"("value"=w523, "channel"=2) -> ()  [unwired: 9 in, 1 out]
          }
          event "LensHV-Set": Value Change {
            n229 = event-data() -> ("NewVal"=w535:dbl)  [unwired: 1 in, 5 out]
            n230 = Divide(x=w535, y=10000.0) -> (x/y=w532:dbl)
            n231 = Multiply(x=w532, y=10.0) -> (x*y=w531:dbl)
            n232 = call "setAO.vi"("value"=w531, "channel"=3) -> ()  [unwired: 9 in, 1 out]
          }
          event "Image": Mouse Down {
            n233 = event-data() -> ("Coords"=w536:T17)  [unwired: 1 in, 7 out]
            n234 = property on="移动" class="Bool (严格)"() -> ("Value"=w537:bool)  [unwired: 2 in, 2 out]
            n235 = case shown="假" w537 {
              tunnel: w536 -> [w548 _]
              frame False {
                w545 = -0.005 ("x")
                n236 = Unbundle(w548) -> ("Horizontal"=w547:i32, "Vertical"=w546:i32)
                n237 = property on="X当前" class="DigNum (严格)"() -> ("Value"=w544:dbl)  [unwired: 2 in, 2 out]
                n238 = property on="Y当前" class="DigNum (严格)"() -> ("Value"=w540:dbl)  [unwired: 2 in, 2 out]
                n239 = Subtract(x=w547, y=252.0) -> (x-y=w550:dbl)
                n240 = Subtract(x=w546, y=191.0) -> (x-y=w549:dbl)
                n241 = Multiply(x=w545, y=w550) -> (x*y=w543:dbl)
                n242 = Multiply(x=w545, y=w549) -> (x*y=w541:dbl)
                n243 = Add(x=w544, y=w543) -> (x+y=w542:dbl)
                n244 = Add(x=w541, y=w540) -> (x+y=w539:dbl)
                n245 = call "goto.vi"("Y(mm)"=w539, "X(mm)"=w542) -> ()  [unwired: 9 in, 1 out]
              }
              frame True {
              }
            }
          }
          event "TakeMS-Run": Value Change {
            n246 = event-data() -> ("NewVal"=w558:bool)  [unwired: 1 in, 5 out]
            n247 = case shown="真" w558 {
              tunnel: w557 -> [_ w574]
              tunnel: w556 -> [_ w571]
              tunnel: w555 -> [_ w570]
              tunnel: w554 -> [w559 w561]
              tunnel: [w559 w560] -> w553
              frame False {
              }
              frame True {
                n248 = Unbundle By Name(w570) -> ("ConfiguredLaserCom"=w567:refnum<visa-resource-name>)
                n249 = Unbundle By Name(w571) -> ("laser semaphore"=w565:T4)
                n250 = property on="cluster" class="Clust (严格)"() -> ("Value"=w569:T8)  [unwired: 2 in, 2 out]
                n251 = Bundle By Name(cluster=w574, "ShotsPerPoint"="Shots/Point") -> (w572:T6)
                n252 = Unbundle By Name(w569) -> ("待机"=w566:bool)
                n253 = property on="SetLaserTransmission" class="Slide (严格)"() -> ("Value"=w564:dbl)  [unwired: 2 in, 2 out]
                n254 = Bundle By Name(cluster="Laser parameter", "VISA resource name"=w567, "standby"=w566, "semaphore in"=w565, "SetLaserEnergy"=w564) -> (w563:T5)
                n255 = case shown="0, 默认" "AcquireMS-Methods" {
                  tunnel: w572 -> [w594 _ _]
                  tunnel: w563 -> [w595 _ _]
                  tunnel: w561 -> [w593 w604 w605]
                  tunnel: [w584 w604 w605] -> w560
                  frame 0, Default {
                    n256 = Get Date/Time String() -> (date string=w591:string, time string=w590:string)  [unwired: 3 in]
                    n257 = Concatenate Strings(w591, " " ("字符串"), w590) -> (w585:string)
                    n258 = call "Tiepie-takeData-2018-06-01.vi"("left rank"="left rank", "right rank"="right rank", "deBaseline"="deBaseline", "Thresh"="Thresh", "Laser parameter"=w595, "ADC parameter"=w594) -> ("output cluster"=w576:cluster{dbl[], "filtered data":dbl[]})  [unwired: 1 in, 1 out]
                    "MS" <- w576
                    n259 = Unbundle(w576) -> (w577:dbl[], "filtered data"=w592:dbl[])
                    n260 = property on="currentNO" class="Str"() -> ("Value"=w587:string)  [unwired: 2 in, 2 out]
                    n261 = Bundle By Name(cluster=T12 {"tag1"="", "tag2"="", "x"=[], "y"=[], "ID1:X"=[], "ID1:Y"=[], "ID1:REF:X"=[], "ID1:REF:Y"=[], "ID2:X"=[], "ID2:Y"=[], "ID2:REF:X"=[], "ID2:REF:Y"=[], "ID3:X"=[], "ID3:Y"=[], "ID3:REF:X"=[], "ID3:REF:Y"=[], "ID1:TAG1"="", "ID1:TAG2"="", "ID2:TAG1"="", "ID2:TAG2"="", "ID3:TAG1"="", "ID3:TAG2"="", "ID1:NAME"="", "ID2:NAME"="", "ID3:NAME"="", "ID1:SCORE"="", "ID2:SCORE"="", "ID3:SCORE"="", "NO"=""}, "y"=w592, "x"=w577, "tag1"="未鉴定", "tag2"=w585, "NO"=w587) -> (w586:T12)
                    n262 = Build Array (concatenate)(w593, w586) -> (w584:T9)
                    n263 = for {
                      tunnel: w584 -> [w603] mode=indexing
                      shift-right: [w596] -> w582
                      shift-left: string[][] [] ("Item Names") -> [w598]
                      i -> [w599]
                      n264 = Unbundle By Name(w603) -> ("NO"=w602:string, "tag1"=w601:string, "tag2"=w600:string)
                      n265 = Build Array(w602, w601, w600) -> (w597:string[])
                      n266 = Insert Into Array "Insert Into Array"(array=w598, index (row)=w599, new element=w597) -> (w596:string[][])  [unwired: 1 in]
                    }
                    n267 = property on="测试记录" class="MCListbox (严格)"("ItemNames"=w582) -> ()  [unwired: 2 in, 2 out]
                  }
                  frame 1 {
                  }
                  frame 2 {
                  }
                }
              }
            }
          }
          event "LaserHV", "频率/Hz", "SetLaserTransmission": Value Change {
            n268 = event-data() -> ()  [unwired: 1 in, 6 out]
            n269 = Unbundle By Name(w614) -> ("ConfiguredLaserCom"=w606:refnum<visa-resource-name>)
            n270 = Unbundle By Name(w615) -> ("laser semaphore"=w610:T4)
            n271 = call <vilib>:"Acquire Semaphore.vi"("semaphore"=w610) -> ("error out"=w609:errorcluster, "semaphore out"=w607:T4)  [unwired: 4 in, 1 out]
            n272 = call "Laser-Set-Parmeter-new.vi"("error in (no error)"=w609, "LaserHV"="LaserHV", "LaserFreq"="频率/Hz", "SetTransmission"="SetLaserTransmission", "VISA resource name"=w606) -> ("error out"=w608:errorcluster)  [unwired: 1 in, 1 out]
            n273 = call <vilib>:"Release Semaphore.vi"("error in (no error)"=w608, "semaphore"=w607) -> ()  [unwired: 4 in, 2 out]
          }
          event "测试记录": Shortcut Menu Selection (User) {
            n274 = event-data() -> ("ItemTag"=w619:string)  [unwired: 1 in, 7 out]
            n275 = case shown="\"鉴定\"" w619 {
              tunnel: w618 -> [w620 w627 w634 w639]
              tunnel: [w620 w627 w634 w635] -> w617
              frame "假", Default {
              }
              frame "鉴定" {
                n276 = property on="selected row" class="DigNum (严格)"() -> ("Value"=w623:i32)  [unwired: 2 in, 2 out]
                n277 = Index Array(array=w627, index=w623) -> (element=w633:T12)
                n278 = Unbundle By Name(w633) -> ("x"=w632:dbl[], "y"=w628:dbl[])
                n279 = call-poly <userlib>:"CaLabPut.vi"("Values"=w632, "PV Names"="MS:X") -> ("Error out"=w630:errorcluster)  [unwired: 6 in, 3 out]
                n280 = call-poly <userlib>:"CaLabPut.vi"("Error in (no error)"=w630, "Values"=w628, "PV Names"="MS:Y") -> ("Error out"=w626:errorcluster)  [unwired: 5 in, 3 out]
                n281 = call-poly <userlib>:"CaLabPut.vi"("Error in (no error)"=w626, "Value"=w623, "PV Name"="MS:NUM") -> ("Error out"=w625:errorcluster)  [unwired: 5 in, 3 out]
                n282 = call-poly <userlib>:"CaLabPut.vi"("Error in (no error)"=w625, "Value"=1, "PV Name"="MS:START") -> ()  [unwired: 5 in, 4 out]
              }
              frame "参数" {
              }
              frame "删除" {
                n283 = property on="selected row" class="DigNum (严格)"() -> ("Value"=w638:i32)  [unwired: 2 in, 2 out]
                n284 = Delete From Array "Delete From Array"(array=w639, index=w638) -> (array with subset deleted=w635:T9)  [unwired: 1 in, 1 out]
                n285 = for {
                  tunnel: w635 -> [w647] mode=indexing
                  shift-right: [w640] -> w636
                  shift-left: string[][] [] ("Item Names") -> [w642]
                  i -> [w643]
                  n286 = Unbundle By Name(w647) -> ("NO"=w646:string, "tag1"=w645:string, "tag2"=w644:string)
                  n287 = Build Array(w646, w645, w644) -> (w641:string[])
                  n288 = Insert Into Array "Insert Into Array"(array=w642, index (row)=w643, new element=w641) -> (w640:string[][])  [unwired: 1 in]
                }
                n289 = property on="测试记录" class="MCListbox (严格)"("ItemNames"=w636) -> ()  [unwired: 2 in, 2 out]
              }
            }
          }
          event "测试记录": Mouse Down {
            n290 = event-data() -> ("Coords"=w653:T17)  [unwired: 1 in, 7 out]
            n291 = invoke on="测试记录" class="MCListbox (严格)" method="Point To Row Column"("Point"=w653) -> ("CellPosition"=w652:T18)  [unwired: 6 in, 6 out]
            n292 = Unbundle By Name(w652) -> ("Row"=w649:i32)
            n293 = Array Size(array=w648) -> (size(s)=w651:i32)
            n294 = Greater Or Equal?(x=w651, y=w649) -> (x >= y?=w650:bool)
            n295 = case shown="真" w650 {
              tunnel: w649 -> [_ w680]
              tunnel: w648 -> [_ w681]
              frame False {
              }
              frame True {
                n296 = property on="selected row" class="DigNum (严格)"("Value"=w680) -> ()  [unwired: 2 in, 2 out]
                n297 = Index Array(array=w681, index=w680) -> (element=w679:T12)
                n298 = Unbundle By Name(w679) -> ("ID1:TAG1"=w662:string, "ID1:TAG2"=w676:string, "ID1:NAME"=w675:string, "ID1:SCORE"=w666:string, "ID2:TAG1"=w660:string, "ID2:TAG2"=w673:string, "ID2:NAME"=w672:string, "ID2:SCORE"=w665:string, "ID3:TAG1"=w658:string, "ID3:TAG2"=w657:string, "ID3:NAME"=w656:string, "ID3:SCORE"=w655:string)
                n299 = Build Array("1" ("element"), w662, w676, w675, w666) -> (w674:string[])
                n300 = Build Array("2" ("element"), w660, w673, w672, w665) -> (w669:string[])
                n301 = Build Array("3" ("element"), w658, w657, w656, w655) -> (w664:string[])
                n302 = Insert Into Array(array=string[][] [] ("项名"), index (row)=0 ("索引 (行)"), new element=w674) -> (w671:string[][])  [unwired: 1 in]
                n303 = Insert Into Array(array=w671, index (row)=1 ("索引 (行)"), new element=w669) -> (w668:string[][])  [unwired: 1 in]
                n304 = Insert Into Array(array=w668, index (row)=2 ("索引 (行)"), new element=w664) -> (w663:string[][])  [unwired: 1 in]
                n305 = property on="Identification Results (单靶鉴定结果)" class="MCListbox (严格)"("ItemNames"=w663) -> ()  [unwired: 2 in, 2 out]
              }
            }
          }
          event "Identification Results (单靶鉴定结果)": Mouse Down {
            n306 = event-data() -> ("Coords"=w687:T17)  [unwired: 1 in, 7 out]
            n307 = invoke on="Identification Results (单靶鉴定结果)" class="MCListbox (严格)" method="Point To Row Column"("Point"=w687) -> ("CellPosition"=w686:T18)  [unwired: 6 in, 6 out]
            n308 = Unbundle By Name(w686) -> ("Row"=w682:i32)
            n309 = Less Or Equal?(x=w682, y=2) -> (x <= y?=w684:bool)
            n310 = case shown="真" w684 {
              tunnel: w683 -> [_ w694]
              tunnel: w682 -> [_ w688]
              frame False {
              }
              frame True {
                n311 = property on="selected row" class="DigNum (严格)"() -> ("Value"=w693:i32)  [unwired: 2 in, 2 out]
                n312 = Index Array(array=w694, index=w693) -> (element=w692:T12)
                n313 = case shown="2" w688 {
                  tunnel: w692 -> [w700 w712 w721]
                  tunnel: [w699 w708 w717] -> w691
                  tunnel: [w698 w707 w716] -> w689
                  frame 0, Default {
                    n314 = Unbundle By Name(w700) -> ("x"=w702:dbl[], "y"=w701:dbl[], "ID1:REF:X"=w703:dbl[], "ID1:REF:Y"=w697:dbl[])
                    n315 = Multiply(x=w697, y=-1.0) -> (x*y=w695:dbl[])
                    n316 = Bundle("x"=w702, "y"=w701) -> (w699:cluster{"x":dbl[], "y":dbl[]})  [unwired: 1 in]
                    n317 = Bundle("ID1:REF:X"=w703, w695) -> (w698:cluster{"ID1:REF:X":dbl[], dbl[]})  [unwired: 1 in]
                  }
                  frame 1 {
                    n318 = Unbundle By Name(w712) -> ("x"=w710:dbl[], "y"=w709:dbl[], "ID2:REF:X"=w711:dbl[], "ID2:REF:Y"=w706:dbl[])
                    n319 = Multiply(x=w706, y=-1.0) -> (x*y=w704:dbl[])
                    n320 = Bundle("x"=w710, "y"=w709) -> (w708:cluster{"x":dbl[], "y":dbl[]})  [unwired: 1 in]
                    n321 = Bundle("ID2:REF:X"=w711, w704) -> (w707:cluster{"ID2:REF:X":dbl[], dbl[]})  [unwired: 1 in]
                  }
                  frame 2 {
                    n322 = Unbundle By Name(w721) -> ("x"=w719:dbl[], "y"=w718:dbl[], "ID3:REF:X"=w720:dbl[], "ID3:REF:Y"=w715:dbl[])
                    n323 = Multiply(x=w715, y=-1.0) -> (x*y=w713:dbl[])
                    n324 = Bundle("x"=w719, "y"=w718) -> (w717:cluster{"x":dbl[], "y":dbl[]})  [unwired: 1 in]
                    n325 = Bundle("ID3:REF:X"=w720, w713) -> (w716:cluster{"ID3:REF:X":dbl[], dbl[]})  [unwired: 1 in]
                  }
                }
                n326 = Build Array(w691, w689) -> (→"Identify Spcetrum":cluster{"ID3:REF:X":dbl[], "y":dbl[]}[])
              }
            }
          }
          event "Plat_To_Zero": Value Change {
            n327 = event-data() -> ("NewVal"=w723:bool)  [unwired: 1 in, 5 out]
            n328 = case shown="假" w723 {
              frame False {
              }
              frame True {
                (unwired) TRUE ("plat zeroed")
                n329 = call "plate_cal.vi"() -> ()  [unwired: 11 in, 1 out]
              }
            }
          }
          event "GO": Value Change {
            n330 = event-data() -> ("NewVal"=w726:bool)  [unwired: 1 in, 5 out]
            n331 = property on="移动" class="Bool (严格)"() -> ("Value"=w728:bool)  [unwired: 2 in, 2 out]
            n332 = Not(x=w728) -> (.not. x?=w727:bool)
            n333 = And(x=w727, y=w726) -> (x .and. y?=w725:bool)
            n334 = case shown="真" w725 {
              frame False {
              }
              frame True {
                n335 = property on="X" class="DigNum (严格)"() -> ("Value"=w730:dbl)  [unwired: 2 in, 2 out]
                n336 = property on="Y" class="DigNum (严格)"() -> ("Value"=w729:dbl)  [unwired: 2 in, 2 out]
                n337 = call "goto.vi"("Y(mm)"=w729, "X(mm)"=w730) -> ()  [unwired: 9 in, 1 out]
              }
            }
          }
          event "chamber in": Value Change {
            n338 = event-data() -> ("NewVal"=w733:bool)  [unwired: 1 in, 5 out]
            n339 = property on="HVEnable" class="Bool (严格)"() -> ("Value"=w738:bool)  [unwired: 2 in, 2 out]
            n340 = property on="Y满" class="Bool (严格)"() -> ("Value"=w734:bool)  [unwired: 2 in, 2 out]
            n341 = property on="移动" class="Bool (严格)"() -> ("Value"=w737:bool)  [unwired: 2 in, 2 out]
            n342 = Not(x=w738) -> (.not. x?=w735:bool)
            n343 = Not(x=w737) -> (.not. x?=w736:bool)
            n344 = Compound Arithmetic op=AND(w735, w734, w736, w733) -> (w732:bool)
            n345 = case shown="真" w732 {
              frame False {
              }
              frame True {
                n346 = flat-sequence {
                  tunnel: [w743] -> w739
                  tunnel: w739 -> [w750]
                  frame #0 {
                    n347 = call "样品标识与备注"() -> ("备注"=w740:string, "样品名称"=w741:string)  [unwired: 16 in, 2 out]
                    n348 = property on="sampleID" class="Str"("Value"=w741) -> ()  [unwired: 2 in, 2 out]
                    n349 = property on="commet" class="Str"("Value"=w740) -> ()  [unwired: 2 in, 2 out]
                  }
                  frame #1 {
                    w744 = FALSE ("on/off")
                    # "关样仓/大气"
                    n350 = Wait (ms)(milliseconds to wait=1500) -> ()  [unwired: 1 out]
                    n351 = call "setDO.vi"("channel"=6, "on/off"=w744) -> ("错误输出"=w742:errorcluster)  [unwired: 9 in]
                    n352 = property on="Samp_Atmos" class="Bool (严格)"(error in=w742, "Value"=w744) -> (error out=w743:errorcluster)  [unwired: 1 in, 1 out]
                  }
                  frame #2 {
                    # "开前泵/样仓"
                    n353 = call "setDO.vi"("错误输入（无错误）"=w750, "channel"=7, "on/off"=TRUE) -> ("错误输出"=w747:errorcluster)  [unwired: 8 in]
                    n354 = while {
                      tunnel: [w757] -> w749
                      tunnel: [w754] -> w748
                      tunnel: w747 -> [w756]
                      stop <- w757 stop-if-true
                      n355 = property on="Lvaccum" class="DigNum (严格)"(error in=w756) -> (error out=w755:errorcluster, "Value"=w759:dbl)  [unwired: 1 in, 1 out]
                      n356 = Less?(x=w759, y=10) -> (x < y?=w757:bool)
                      n357 = call "时间延迟"("error in (no error)"=w755, "Delay Time (s)"=1.0) -> ("error out"=w754:errorcluster)  [unwired: 9 in]
                    }
                    n358 = case shown="假" w749 {
                      tunnel: w748 -> [w761 w763]
                      frame False {
                        (unwired) 7
                        n359 = call "setDO.vi"("错误输入（无错误）"=w761, "on/off"=FALSE) -> ("错误输出"=w760:errorcluster)  [unwired: 9 in]
                        n360 = call "Display Message to User4"("error in (no error)"=w760) -> ()  [unwired: 9 in, 2 out]
                      }
                      frame True {
                        n361 = flat-sequence {
                          tunnel: w763 -> [w764]
                          frame #0 {
                            n362 = call "setDO.vi"("错误输入（无错误）"=w764, "channel"=7, "on/off"=FALSE) -> ()  [unwired: 8 in, 1 out]
                          }
                          frame #1 {
                            n363 = call "chamber_in.vi"() -> ()  [unwired: 12 in]
                          }
                        }
                      }
                    }
                  }
                }
              }
            }
          }
          event "chamber out": Value Change {
            n364 = event-data() -> ("NewVal"=w767:bool)  [unwired: 1 in, 5 out]
            n365 = case shown="真" w767 {
              frame False {
              }
              frame True {
                n366 = property on="移动" class="Bool (严格)"() -> ("Value"=w773:bool)  [unwired: 2 in, 2 out]
                n367 = property on="Y满" class="Bool (严格)"() -> ("Value"=w774:bool)  [unwired: 2 in, 2 out]
                n368 = property on="HVEnable" class="Bool (严格)"() -> ("Value"=w775:bool)  [unwired: 2 in, 2 out]
                n369 = Not "非"(x=w773) -> (.not. x?=w771:bool)
                n370 = Not "非"(x=w774) -> (.not. x?=w772:bool)
                n371 = Not "非"(x=w775) -> (.not. x?=w769:bool)
                n372 = Compound Arithmetic op=AND "复合运算"(w769, w772, w771) -> (w770:bool)
                n373 = case shown="真" w770 {
                  frame False {
                    n374 = call "Display Message to User3"() -> ()  [unwired: 10 in, 2 out]
                  }
                  frame True {
                    n375 = flat-sequence {
                      tunnel: [w779] -> w777
                      tunnel: w777 -> [w785]
                      tunnel: [w786] -> w776
                      tunnel: w776 -> [w797]
                      frame #0 {
                        n376 = call "chamber_out.vi"() -> ()  [unwired: 12 in]
                      }
                      frame #1 {
                        w780 = FALSE ("on/off")
                        # "关前泵/样仓"
                        n377 = Wait (ms)(milliseconds to wait=1500) -> ()  [unwired: 1 out]
                        n378 = call "setDO.vi"("channel"=7, "on/off"=w780) -> ("错误输出"=w778:errorcluster)  [unwired: 9 in]
                        n379 = property on="Fore_Samp" class="Bool (严格)"(error in=w778, "Value"=w780) -> (error out=w779:errorcluster)  [unwired: 1 in, 1 out]
                      }
                      frame #2 {
                        # "开样仓/大气"
                        n380 = call "Time Delay4"("error in (no error)"=w785, "Delay Time (s)"=3.0) -> ("error out"=w784:errorcluster)  [unwired: 9 in]
                        n381 = property on="Y满" class="Bool (严格)"(error in=w784) -> (error out=w787:errorcluster, "Value"=w788:bool)  [unwired: 1 in, 1 out]
                        n382 = case shown="真" w788 {
                          tunnel: w787 -> [w790 w792]
                          tunnel: [w789 w791] -> w786
                          frame False {
                            n383 = call "Display Message to User2"("error in (no error)"=w790) -> ("error out"=w789:errorcluster)  [unwired: 9 in, 1 out]
                          }
                          frame True {
                            n384 = call "setDO.vi"("错误输入（无错误）"=w792, "channel"=6, "on/off"=TRUE) -> ("错误输出"=w791:errorcluster)  [unwired: 8 in]
                          }
                        }
                      }
                      frame #3 {
                        n385 = call "Time Delay5"("error in (no error)"=w797, "Delay Time (s)"=3.0) -> ("error out"=w796:errorcluster)  [unwired: 9 in]
                        n386 = call "setDO.vi"("错误输入（无错误）"=w796, "channel"=6, "on/off"=FALSE) -> ()  [unwired: 8 in, 1 out]
                      }
                    }
                  }
                }
              }
            }
          }
          event "标准样品": Value Change {
            n387 = event-data() -> ("NewVal"=w800:u16)  [unwired: 1 in, 5 out]
            n388 = local read "std sample"() -> (w804:T2)
            n389 = control-ref of="定标参数"() -> (w805:refnum<vi>)
            n390 = property on="config" class="TypRef (严格)"() -> ("Value"=w803:T1)  [unwired: 2 in, 2 out]
            n391 = call-poly <vilib>:"Write Key.vi"("section"="cal", "value"=w800, "key"="type", "refnum"=w803) -> ()  [unwired: 5 in, 3 out]
            n392 = call "writetable.vi"("std sample"=w804, "type"=w800, "reference"=w805) -> ()  [unwired: 9 in]
          }
          event "peak cal": Value Change {
            n393 = event-data() -> ("NewVal"=w807:bool)  [unwired: 1 in, 5 out]
            n394 = case shown="真" w807 {
              frame False {
              }
              frame True {
                w819 = "cal" ("section")
                n395 = property on="定标参数" class="MCListbox (严格)"() -> ("ItemNames"=w838:string[][])  [unwired: 2 in, 2 out]
                n396 = Index Array(array=w838, index (col)=1 ("disabled index (col)")) -> (element=w839:string[])  [unwired: 1 in]
                n397 = Index Array(array=w838, index (col)=3 ("disabled index (col)")) -> (element=w836:string[])  [unwired: 1 in]
                n398 = property on="config" class="TypRef (严格)"() -> ("Value"=w813:T1)  [unwired: 2 in, 2 out]
                n399 = Fract/Exp String To Number(string=w836) -> (number=w814:dbl[])  [unwired: 3 in, 1 out]
                n400 = Fract/Exp String To Number(string=w839) -> (number=w829:dbl[])  [unwired: 3 in, 1 out]
                n401 = call "write_peak_data.vi"("array in"=w814, "refnum"=w813) -> ("error out"=w811:errorcluster, "refnum out"=w812:T1)  [unwired: 8 in]
                n402 = call <vilib>:"General Polynomial Fit.vi"("Y"=w829, "polynomial order"=2, "X"=w814) -> ("Polynomial Coefficients"=w832:dbl[])  [unwired: 9 in, 3 out]
                n403 = Index Array(array=w832, index=2) -> (element=w822:dbl)
                "a:" <- w822
                n404 = Index Array(array=w832, index=1) -> (element=w817:dbl)
                "b:" <- w817
                n405 = Index Array(array=w832, index=0) -> (element=w816:dbl)
                "c:" <- w816
                n406 = global write "cal_p.vi" "a"(w822) -> ()
                n407 = global write "cal_p.vi" "b"(w817) -> ()
                n408 = for {
                  tunnel: w814 -> [w853] mode=indexing
                  tunnel: [w857] -> w830 mode=indexing
                  tunnel: w816 -> [w854]
                  tunnel: w817 -> [w855]
                  tunnel: w822 -> [w856]
                  n409 = formula code="m=a*x*x+b*x+c;"("a"=w856, "b"=w855, "c"=w854, "x"=w853) -> ("m"=w857:dbl)
                }
                n410 = global write "cal_p.vi" "c"(w816) -> ()
                n411 = call-poly <vilib>:"Write Key.vi"("section"=w819, "error in (no error)"=w811, "value"=w822, "key"="a", "refnum"=w812) -> ("error out"=w810:errorcluster, "refnum out"=w821:T1)  [unwired: 4 in, 1 out]
                n412 = for {
                  tunnel: w830 -> [w851] mode=indexing
                  tunnel: w829 -> [w852] mode=indexing
                  tunnel: [w850] -> w824 mode=indexing
                  n413 = formula code="delta=100*(m-m0)/m0;"("m0"=w852, "m"=w851) -> ("delta"=w850:dbl)
                }
                n414 = call-poly <vilib>:"Write Key.vi"("section"=w819, "error in (no error)"=w810, "value"=w817, "key"="b", "refnum"=w821) -> ("error out"=w809:errorcluster, "refnum out"=w815:T1)  [unwired: 4 in, 1 out]
                n415 = call-poly <vilib>:"Write Key.vi"("section"=w819, "error in (no error)"=w809, "value"=w816, "key"="c", "refnum"=w815) -> ()  [unwired: 4 in, 3 out]
                n416 = control-ref of="定标参数"() -> (w828:refnum<vi>)
                n417 = property on="Property Node" class="MCListbox (严格)"(reference=w828) -> (reference out=w827:refnum<vi>, "ItemNames"=w826:string[][])  [unwired: 1 in, 1 out]
                n418 = for {
                  shift-right: [w846] -> w825
                  shift-left: w826 -> [w849]
                  tunnel: w824 -> [w847] mode=indexing
                  i -> [w848]
                  n419 = Number To Fractional String(number=w847, precision (6)=i16 2) -> (F-format string=w844:string)  [unwired: 2 in]
                  n420 = Concatenate Strings(w844, "%" ("string")) -> (w842:string)
                  n421 = Replace Array Subset(array=w849, new element=w842, index (row)=w848, index (col)=4 ("disabled index (col)")) -> (w846:string[][])
                }
                n422 = property on="Property Node" class="MCListbox (严格)"(reference=w827, "ItemNames"=w825) -> ()  [unwired: 1 in, 2 out]
              }
            }
          }
          event "A1-Position": Value Change {
            n423 = event-data() -> ("NewVal"=w859:bool)  [unwired: 1 in, 5 out]
            n424 = case shown="真" w859 {
              frame False {
              }
              frame True {
                n425 = property on="X当前" class="DigNum (严格)"() -> ("Value"=w865:dbl)  [unwired: 2 in, 2 out]
                "A1-position-X" <- w865
                n426 = property on="Y当前" class="DigNum (严格)"() -> ("Value"=w860:dbl)  [unwired: 2 in, 2 out]
                "A1-position-Y" <- w860
                n427 = property on="config" class="TypRef (严格)"() -> ("Value"=w868:T1)  [unwired: 2 in, 2 out]
                n428 = call-poly <vilib>:"Write Key.vi"("section"="motor", "value"=w865, "key"="a1x", "refnum"=w868) -> ("error out"=w861:errorcluster, "refnum out"=w862:T1)  [unwired: 5 in, 1 out]
                n429 = call-poly <vilib>:"Write Key.vi"("section"="motor", "error in (no error)"=w861, "value"=w860, "key"="a1y", "refnum"=w862) -> ()  [unwired: 4 in, 3 out]
              }
            }
          }
          event "A1": Value Change {
            n430 = event-data() -> ("NewVal"=w872:bool)  [unwired: 1 in, 5 out]
            n431 = property on="移动" class="Bool (严格)"() -> ("Value"=w874:bool)  [unwired: 2 in, 2 out]
            n432 = Not(x=w874) -> (.not. x?=w873:bool)
            n433 = And(x=w873, y=w872) -> (x .and. y?=w871:bool)
            n434 = case shown="真" w871 {
              frame False {
              }
              frame True {
                n435 = property on="A1-position-X" class="DigNum (严格)"() -> (error out=w879:errorcluster, "Value"=w877:dbl)  [unwired: 2 in, 1 out]
                n436 = property on="A1-position-Y" class="DigNum (严格)"(error in=w879) -> (error out=w878:errorcluster, "Value"=w876:dbl)  [unwired: 1 in, 1 out]
                n437 = vi-ref "goto.vi"() -> (w883:refnum<vi>)
                n438 = property class="VI"(reference=w883, error in=w878) -> ("Name"=w882:string)  [unwired: 2 out]
                n439 = Open VI Reference(type specifier VI Refnum (for type only)=refnum<vi> refnum, vi path=w882, options=128) -> (vi reference=w880:refnum<vi>)  [unwired: 3 in, 1 out]
                n440 = call-by-ref "Start Asynchronous Call"(reference=w880, "Y(mm)"=w876, "X(mm)"=w877) -> ()  [unwired: 10 in, 3 out]
              }
            }
            n441 = property on="currentNO" class="Str"("Val(Sgnl)"="A1") -> ()  [unwired: 2 in, 2 out]
          }
          event "A2": Value Change {
            n442 = event-data() -> ("NewVal"=w887:bool)  [unwired: 1 in, 5 out]
            n443 = property on="移动" class="Bool (严格)"() -> ("Value"=w890:bool)  [unwired: 2 in, 2 out]
            n444 = Not(x=w890) -> (.not. x?=w889:bool)
            n445 = And(x=w889, y=w887) -> (x .and. y?=w888:bool)
            n446 = case shown="真" w888 {
              frame False {
              }
              frame True {
                n447 = property on="A1-position-X" class="DigNum (严格)"() -> (error out=w894:errorcluster, "Value"=w901:dbl)  [unwired: 2 in, 1 out]
                n448 = property on="A1-position-Y" class="DigNum (严格)"(error in=w894) -> (error out=w893:errorcluster, "Value"=w891:dbl)  [unwired: 1 in, 1 out]
                n449 = Subtract(x=w901, y=4.5) -> (x-y=w892:dbl)
                n450 = vi-ref "goto.vi"() -> (w899:refnum<vi>)
                n451 = property class="VI"(reference=w899, error in=w893) -> ("Name"=w898:string)  [unwired: 2 out]
                n452 = Open VI Reference(type specifier VI Refnum (for type only)=refnum<vi> refnum, vi path=w898, options=128) -> (vi reference=w896:refnum<vi>)  [unwired: 3 in, 1 out]
                n453 = call-by-ref "Start Asynchronous Call"(reference=w896, "Y(mm)"=w891, "X(mm)"=w892) -> ()  [unwired: 10 in, 3 out]
              }
            }
            n454 = control-ref of="currentNO"() -> (w884:refnum<vi>)
            n455 = property on="属性节点" class="Str"(reference=w884, "Val(Sgnl)"="A2") -> ()  [unwired: 1 in, 2 out]
          }
          event "A3": Value Change {
            n456 = event-data() -> ("NewVal"=w905:bool)  [unwired: 1 in, 5 out]
            n457 = property on="移动" class="Bool (严格)"() -> ("Value"=w908:bool)  [unwired: 2 in, 2 out]
            n458 = Not(x=w908) -> (.not. x?=w907:bool)
            n459 = And(x=w907, y=w905) -> (x .and. y?=w906:bool)
            n460 = case shown="真" w906 {
              frame False {
              }
              frame True {
                n461 = property on="A1-position-X" class="DigNum (严格)"() -> (error out=w912:errorcluster, "Value"=w919:dbl)  [unwired: 2 in, 1 out]
                n462 = property on="A1-position-Y" class="DigNum (严格)"(error in=w912) -> (error out=w911:errorcluster, "Value"=w909:dbl)  [unwired: 1 in, 1 out]
                n463 = Subtract(x=w919, y=9.0) -> (x-y=w910:dbl)
                n464 = vi-ref "goto.vi"() -> (w917:refnum<vi>)
                n465 = property class="VI"(reference=w917, error in=w911) -> ("Name"=w916:string)  [unwired: 2 out]
                n466 = Open VI Reference(type specifier VI Refnum (for type only)=refnum<vi> refnum, vi path=w916, options=128) -> (vi reference=w914:refnum<vi>)  [unwired: 3 in, 1 out]
                n467 = call-by-ref "Start Asynchronous Call"(reference=w914, "Y(mm)"=w909, "X(mm)"=w910) -> ()  [unwired: 10 in, 3 out]
              }
            }
            n468 = control-ref of="currentNO"() -> (w902:refnum<vi>)
            n469 = property on="属性节点" class="Str"(reference=w902, "Val(Sgnl)"="A3") -> ()  [unwired: 1 in, 2 out]
          }
          event "A4": Value Change {
            n470 = event-data() -> ("NewVal"=w922:bool)  [unwired: 1 in, 5 out]
            n471 = property on="移动" class="Bool (严格)"() -> ("Value"=w925:bool)  [unwired: 2 in, 2 out]
            n472 = Not(x=w925) -> (.not. x?=w924:bool)
            n473 = And(x=w924, y=w922) -> (x .and. y?=w923:bool)
            n474 = case shown="真" w923 {
              frame False {
              }
              frame True {
                n475 = property on="A1-position-X" class="DigNum (严格)"() -> (error out=w929:errorcluster, "Value"=w936:dbl)  [unwired: 2 in, 1 out]
                n476 = property on="A1-position-Y" class="DigNum (严格)"(error in=w929) -> (error out=w928:errorcluster, "Value"=w926:dbl)  [unwired: 1 in, 1 out]
                n477 = Subtract(x=w936, y=13.5) -> (x-y=w927:dbl)
                n478 = vi-ref "goto.vi"() -> (w934:refnum<vi>)
                n479 = property class="VI"(reference=w934, error in=w928) -> ("Name"=w933:string)  [unwired: 2 out]
                n480 = Open VI Reference(type specifier VI Refnum (for type only)=refnum<vi> refnum, vi path=w933, options=128) -> (vi reference=w931:refnum<vi>)  [unwired: 3 in, 1 out]
                n481 = call-by-ref "Start Asynchronous Call"(reference=w931, "Y(mm)"=w926, "X(mm)"=w927) -> ()  [unwired: 10 in, 3 out]
              }
            }
            n482 = property on="currentNO" class="Str"("Val(Sgnl)"="A4") -> ()  [unwired: 2 in, 2 out]
          }
          event "A5": Value Change {
            n483 = event-data() -> ("NewVal"=w939:bool)  [unwired: 1 in, 5 out]
            n484 = property on="移动" class="Bool (严格)"() -> ("Value"=w942:bool)  [unwired: 2 in, 2 out]
            n485 = Not(x=w942) -> (.not. x?=w941:bool)
            n486 = And(x=w941, y=w939) -> (x .and. y?=w940:bool)
            n487 = case shown="真" w940 {
              frame False {
              }
              frame True {
                n488 = property on="A1-position-X" class="DigNum (严格)"() -> (error out=w946:errorcluster, "Value"=w953:dbl)  [unwired: 2 in, 1 out]
                n489 = property on="A1-position-Y" class="DigNum (严格)"(error in=w946) -> (error out=w945:errorcluster, "Value"=w943:dbl)  [unwired: 1 in, 1 out]
                n490 = Subtract(x=w953, y=18) -> (x-y=w944:dbl)
                n491 = vi-ref "goto.vi"() -> (w951:refnum<vi>)
                n492 = property class="VI"(reference=w951, error in=w945) -> ("Name"=w950:string)  [unwired: 2 out]
                n493 = Open VI Reference(type specifier VI Refnum (for type only)=refnum<vi> refnum, vi path=w950, options=128) -> (vi reference=w948:refnum<vi>)  [unwired: 3 in, 1 out]
                n494 = call-by-ref "Start Asynchronous Call"(reference=w948, "Y(mm)"=w943, "X(mm)"=w944) -> ()  [unwired: 10 in, 3 out]
              }
            }
            n495 = property on="currentNO" class="Str"("Val(Sgnl)"="A5") -> ()  [unwired: 2 in, 2 out]
          }
          event "A6": Value Change {
            n496 = event-data() -> ("NewVal"=w956:bool)  [unwired: 1 in, 5 out]
            n497 = property on="移动" class="Bool (严格)"() -> ("Value"=w959:bool)  [unwired: 2 in, 2 out]
            n498 = Not(x=w959) -> (.not. x?=w958:bool)
            n499 = And(x=w958, y=w956) -> (x .and. y?=w957:bool)
            n500 = case shown="真" w957 {
              frame False {
              }
              frame True {
                n501 = property on="A1-position-X" class="DigNum (严格)"() -> (error out=w963:errorcluster, "Value"=w970:dbl)  [unwired: 2 in, 1 out]
                n502 = property on="A1-position-Y" class="DigNum (严格)"(error in=w963) -> (error out=w962:errorcluster, "Value"=w960:dbl)  [unwired: 1 in, 1 out]
                n503 = Subtract(x=w970, y=22.5) -> (x-y=w961:dbl)
                n504 = vi-ref "goto.vi"() -> (w968:refnum<vi>)
                n505 = property class="VI"(reference=w968, error in=w962) -> ("Name"=w967:string)  [unwired: 2 out]
                n506 = Open VI Reference(type specifier VI Refnum (for type only)=refnum<vi> refnum, vi path=w967, options=128) -> (vi reference=w965:refnum<vi>)  [unwired: 3 in, 1 out]
                n507 = call-by-ref "Start Asynchronous Call"(reference=w965, "Y(mm)"=w960, "X(mm)"=w961) -> ()  [unwired: 10 in, 3 out]
              }
            }
            n508 = property on="currentNO" class="Str"("Val(Sgnl)"="A6") -> ()  [unwired: 2 in, 2 out]
          }
          event "A7": Value Change {
            n509 = event-data() -> ("NewVal"=w973:bool)  [unwired: 1 in, 5 out]
            n510 = property on="移动" class="Bool (严格)"() -> ("Value"=w976:bool)  [unwired: 2 in, 2 out]
            n511 = Not(x=w976) -> (.not. x?=w975:bool)
            n512 = And(x=w975, y=w973) -> (x .and. y?=w974:bool)
            n513 = case shown="真" w974 {
              frame False {
              }
              frame True {
                n514 = property on="A1-position-X" class="DigNum (严格)"() -> (error out=w980:errorcluster, "Value"=w987:dbl)  [unwired: 2 in, 1 out]
                n515 = property on="A1-position-Y" class="DigNum (严格)"(error in=w980) -> (error out=w979:errorcluster, "Value"=w977:dbl)  [unwired: 1 in, 1 out]
                n516 = Subtract(x=w987, y=27) -> (x-y=w978:dbl)
                n517 = vi-ref "goto.vi"() -> (w985:refnum<vi>)
                n518 = property class="VI"(reference=w985, error in=w979) -> ("Name"=w984:string)  [unwired: 2 out]
                n519 = Open VI Reference(type specifier VI Refnum (for type only)=refnum<vi> refnum, vi path=w984, options=128) -> (vi reference=w982:refnum<vi>)  [unwired: 3 in, 1 out]
                n520 = call-by-ref "Start Asynchronous Call"(reference=w982, "Y(mm)"=w977, "X(mm)"=w978) -> ()  [unwired: 10 in, 3 out]
              }
            }
            n521 = property on="currentNO" class="Str"("Val(Sgnl)"="A7") -> ()  [unwired: 2 in, 2 out]
          }
          event User Event {
            n522 = event-data() -> ("PV name"=w989:string, "value array (string)"=w988:string[])  [unwired: 1 in, 9 out]
            n523 = case shown="\"ID:STATUS\"" w989 {
              tunnel: w991 -> [w995 w1001]
              tunnel: [w995 w1004] -> w990
              tunnel: w988 -> [w994 _]
              frame "ID:INFO", Default {
                n524 = Index Array(array=w994, index=0) -> (element=→"idn status":string)
              }
              frame "ID:STATUS" {
                n525 = call "getIOCdata.vi"() -> ("输出簇"=w1002:T12)  [unwired: 11 in]
                n526 = call-poly <userlib>:"CaLabGet.vi"("PV Name"="MS:NUM") -> ("1rst Value (number)"=w1000:dbl)  [unwired: 8 in, 6 out]
                n527 = Index Array(array=w1001, index=w1000) -> (element=w999:T12)
                n528 = Unbundle By Name(w999) -> ("NO"=w998:string, "tag2"=w997:string)
                n529 = Bundle By Name(cluster=w1002, "NO"=w998, "tag2"=w997) -> (w996:T12)
                n530 = Replace Array Subset "Replace Array Subset"(array=w1001, new element=w996, index=w1000) -> (w1004:T9)
                n531 = for {
                  tunnel: w1004 -> [w1014] mode=indexing
                  shift-right: [w1007] -> w1003
                  shift-left: string[][] [] ("Item Names") -> [w1009]
                  i -> [w1010]
                  n532 = Unbundle By Name(w1014) -> ("NO"=w1013:string, "tag1"=w1012:string, "tag2"=w1011:string)
                  n533 = Build Array(w1013, w1012, w1011) -> (w1008:string[])
                  n534 = Insert Into Array "Insert Into Array"(array=w1009, index (row)=w1010, new element=w1008) -> (w1007:string[][])  [unwired: 1 in]
                }
                n535 = property on="测试记录" class="MCListbox (严格)"("ItemNames"=w1003) -> ()  [unwired: 2 in, 2 out]
              }
            }
          }
          event "A8": Value Change {
            n536 = event-data() -> ("NewVal"=w1017:bool)  [unwired: 1 in, 5 out]
            n537 = property on="移动" class="Bool (严格)"() -> ("Value"=w1020:bool)  [unwired: 2 in, 2 out]
            n538 = Not(x=w1020) -> (.not. x?=w1019:bool)
            n539 = And(x=w1019, y=w1017) -> (x .and. y?=w1018:bool)
            n540 = case shown="假" w1018 {
              frame False {
              }
              frame True {
                n541 = property on="A1-position-X" class="DigNum (严格)"() -> (error out=w1024:errorcluster, "Value"=w1031:dbl)  [unwired: 2 in, 1 out]
                n542 = property on="A1-position-Y" class="DigNum (严格)"(error in=w1024) -> (error out=w1023:errorcluster, "Value"=w1021:dbl)  [unwired: 1 in, 1 out]
                n543 = Subtract(x=w1031, y=31.5) -> (x-y=w1022:dbl)
                n544 = vi-ref "goto.vi"() -> (w1029:refnum<vi>)
                n545 = property class="VI"(reference=w1029, error in=w1023) -> ("Name"=w1028:string)  [unwired: 2 out]
                n546 = Open VI Reference(type specifier VI Refnum (for type only)=refnum<vi> refnum, vi path=w1028, options=128) -> (vi reference=w1026:refnum<vi>)  [unwired: 3 in, 1 out]
                n547 = call-by-ref "Start Asynchronous Call"(reference=w1026, "Y(mm)"=w1021, "X(mm)"=w1022) -> ()  [unwired: 10 in, 3 out]
              }
            }
            n548 = property on="currentNO" class="Str"("Val(Sgnl)"="A8") -> ()  [unwired: 2 in, 2 out]
          }
          event "A9": Value Change {
            n549 = event-data() -> ("NewVal"=w1034:bool)  [unwired: 1 in, 5 out]
            n550 = property on="移动" class="Bool (严格)"() -> ("Value"=w1037:bool)  [unwired: 2 in, 2 out]
            n551 = Not(x=w1037) -> (.not. x?=w1036:bool)
            n552 = And(x=w1036, y=w1034) -> (x .and. y?=w1035:bool)
            n553 = case shown="真" w1035 {
              frame False {
              }
              frame True {
                n554 = property on="A1-position-X" class="DigNum (严格)"() -> (error out=w1041:errorcluster, "Value"=w1048:dbl)  [unwired: 2 in, 1 out]
                n555 = property on="A1-position-Y" class="DigNum (严格)"(error in=w1041) -> (error out=w1040:errorcluster, "Value"=w1038:dbl)  [unwired: 1 in, 1 out]
                n556 = Subtract(x=w1048, y=36) -> (x-y=w1039:dbl)
                n557 = vi-ref "goto.vi"() -> (w1046:refnum<vi>)
                n558 = property class="VI"(reference=w1046, error in=w1040) -> ("Name"=w1045:string)  [unwired: 2 out]
                n559 = Open VI Reference(type specifier VI Refnum (for type only)=refnum<vi> refnum, vi path=w1045, options=128) -> (vi reference=w1043:refnum<vi>)  [unwired: 3 in, 1 out]
                n560 = call-by-ref "Start Asynchronous Call"(reference=w1043, "Y(mm)"=w1038, "X(mm)"=w1039) -> ()  [unwired: 10 in, 3 out]
              }
            }
            n561 = property on="currentNO" class="Str"("Val(Sgnl)"="A9") -> ()  [unwired: 2 in, 2 out]
          }
          event "A10": Value Change {
            n562 = event-data() -> ("NewVal"=w1051:bool)  [unwired: 1 in, 5 out]
            n563 = property on="移动" class="Bool (严格)"() -> ("Value"=w1054:bool)  [unwired: 2 in, 2 out]
            n564 = Not(x=w1054) -> (.not. x?=w1053:bool)
            n565 = And(x=w1053, y=w1051) -> (x .and. y?=w1052:bool)
            n566 = case shown="真" w1052 {
              frame False {
              }
              frame True {
                n567 = property on="A1-position-X" class="DigNum (严格)"() -> (error out=w1058:errorcluster, "Value"=w1065:dbl)  [unwired: 2 in, 1 out]
                n568 = property on="A1-position-Y" class="DigNum (严格)"(error in=w1058) -> (error out=w1057:errorcluster, "Value"=w1055:dbl)  [unwired: 1 in, 1 out]
                n569 = Subtract(x=w1065, y=40.5) -> (x-y=w1056:dbl)
                n570 = vi-ref "goto.vi"() -> (w1063:refnum<vi>)
                n571 = property class="VI"(reference=w1063, error in=w1057) -> ("Name"=w1062:string)  [unwired: 2 out]
                n572 = Open VI Reference(type specifier VI Refnum (for type only)=refnum<vi> refnum, vi path=w1062, options=128) -> (vi reference=w1060:refnum<vi>)  [unwired: 3 in, 1 out]
                n573 = call-by-ref "Start Asynchronous Call"(reference=w1060, "Y(mm)"=w1055, "X(mm)"=w1056) -> ()  [unwired: 10 in, 3 out]
              }
            }
            n574 = property on="currentNO" class="Str"("Val(Sgnl)"="A10") -> ()  [unwired: 2 in, 2 out]
          }
          event "A11": Value Change {
            n575 = event-data() -> ("NewVal"=w1068:bool)  [unwired: 1 in, 5 out]
            n576 = property on="移动" class="Bool (严格)"() -> ("Value"=w1071:bool)  [unwired: 2 in, 2 out]
            n577 = Not(x=w1071) -> (.not. x?=w1070:bool)
            n578 = And(x=w1070, y=w1068) -> (x .and. y?=w1069:bool)
            n579 = case shown="真" w1069 {
              frame False {
              }
              frame True {
                n580 = property on="A1-position-X" class="DigNum (严格)"() -> (error out=w1075:errorcluster, "Value"=w1082:dbl)  [unwired: 2 in, 1 out]
                n581 = property on="A1-position-Y" class="DigNum (严格)"(error in=w1075) -> (error out=w1074:errorcluster, "Value"=w1072:dbl)  [unwired: 1 in, 1 out]
                n582 = Subtract(x=w1082, y=45) -> (x-y=w1073:dbl)
                n583 = vi-ref "goto.vi"() -> (w1080:refnum<vi>)
                n584 = property class="VI"(reference=w1080, error in=w1074) -> ("Name"=w1079:string)  [unwired: 2 out]
                n585 = Open VI Reference(type specifier VI Refnum (for type only)=refnum<vi> refnum, vi path=w1079, options=128) -> (vi reference=w1077:refnum<vi>)  [unwired: 3 in, 1 out]
                n586 = call-by-ref "Start Asynchronous Call"(reference=w1077, "Y(mm)"=w1072, "X(mm)"=w1073) -> ()  [unwired: 10 in, 3 out]
              }
            }
            n587 = property on="currentNO" class="Str"("Val(Sgnl)"="A11") -> ()  [unwired: 2 in, 2 out]
          }
          event "A12": Value Change {
            n588 = event-data() -> ("NewVal"=w1085:bool)  [unwired: 1 in, 5 out]
            n589 = property on="移动" class="Bool (严格)"() -> ("Value"=w1088:bool)  [unwired: 2 in, 2 out]
            n590 = Not(x=w1088) -> (.not. x?=w1087:bool)
            n591 = And(x=w1087, y=w1085) -> (x .and. y?=w1086:bool)
            n592 = case shown="真" w1086 {
              frame False {
              }
              frame True {
                n593 = property on="A1-position-X" class="DigNum (严格)"() -> (error out=w1092:errorcluster, "Value"=w1099:dbl)  [unwired: 2 in, 1 out]
                n594 = property on="A1-position-Y" class="DigNum (严格)"(error in=w1092) -> (error out=w1091:errorcluster, "Value"=w1089:dbl)  [unwired: 1 in, 1 out]
                n595 = Subtract(x=w1099, y=49.5) -> (x-y=w1090:dbl)
                n596 = vi-ref "goto.vi"() -> (w1097:refnum<vi>)
                n597 = property class="VI"(reference=w1097, error in=w1091) -> ("Name"=w1096:string)  [unwired: 2 out]
                n598 = Open VI Reference(type specifier VI Refnum (for type only)=refnum<vi> refnum, vi path=w1096, options=128) -> (vi reference=w1094:refnum<vi>)  [unwired: 3 in, 1 out]
                n599 = call-by-ref "Start Asynchronous Call"(reference=w1094, "Y(mm)"=w1089, "X(mm)"=w1090) -> ()  [unwired: 10 in, 3 out]
              }
            }
            n600 = property on="currentNO" class="Str"("Val(Sgnl)"="A12") -> ()  [unwired: 2 in, 2 out]
          }
          event "B1": Value Change {
            n601 = event-data() -> ("NewVal"=w1102:bool)  [unwired: 1 in, 5 out]
            n602 = property on="移动" class="Bool (严格)"() -> ("Value"=w1105:bool)  [unwired: 2 in, 2 out]
            n603 = Not(x=w1105) -> (.not. x?=w1104:bool)
            n604 = And(x=w1104, y=w1102) -> (x .and. y?=w1103:bool)
            n605 = case shown="真" w1103 {
              frame False {
              }
              frame True {
                n606 = property on="A1-position-X" class="DigNum (严格)"() -> (error out=w1111:errorcluster, "Value"=w1118:dbl)  [unwired: 2 in, 1 out]
                n607 = property on="A1-position-Y" class="DigNum (严格)"(error in=w1111) -> (error out=w1110:errorcluster, "Value"=w1107:dbl)  [unwired: 1 in, 1 out]
                n608 = Subtract(x=w1107, y=4.5) -> (x-y=w1106:dbl)
                n609 = Subtract(x=w1118, y=0) -> (x-y=w1109:dbl)
                n610 = vi-ref "goto.vi"() -> (w1116:refnum<vi>)
                n611 = property class="VI"(reference=w1116, error in=w1110) -> ("Name"=w1115:string)  [unwired: 2 out]
                n612 = Open VI Reference(type specifier VI Refnum (for type only)=refnum<vi> refnum, vi path=w1115, options=128) -> (vi reference=w1113:refnum<vi>)  [unwired: 3 in, 1 out]
                n613 = call-by-ref "Start Asynchronous Call"(reference=w1113, "Y(mm)"=w1106, "X(mm)"=w1109) -> ()  [unwired: 10 in, 3 out]
              }
            }
            n614 = property on="currentNO" class="Str"("Val(Sgnl)"="B1") -> ()  [unwired: 2 in, 2 out]
          }
          event "B2": Value Change {
            n615 = event-data() -> ("NewVal"=w1121:bool)  [unwired: 1 in, 5 out]
            n616 = property on="移动" class="Bool (严格)"() -> ("Value"=w1124:bool)  [unwired: 2 in, 2 out]
            n617 = Not(x=w1124) -> (.not. x?=w1123:bool)
            n618 = And(x=w1123, y=w1121) -> (x .and. y?=w1122:bool)
            n619 = case shown="真" w1122 {
              frame False {
              }
              frame True {
                n620 = property on="A1-position-X" class="DigNum (严格)"() -> (error out=w1130:errorcluster, "Value"=w1137:dbl)  [unwired: 2 in, 1 out]
                n621 = property on="A1-position-Y" class="DigNum (严格)"(error in=w1130) -> (error out=w1129:errorcluster, "Value"=w1126:dbl)  [unwired: 1 in, 1 out]
                n622 = Subtract(x=w1126, y=4.5) -> (x-y=w1125:dbl)
                n623 = Subtract(x=w1137, y=4.5) -> (x-y=w1128:dbl)
                n624 = vi-ref "goto.vi"() -> (w1135:refnum<vi>)
                n625 = property class="VI"(reference=w1135, error in=w1129) -> ("Name"=w1134:string)  [unwired: 2 out]
                n626 = Open VI Reference(type specifier VI Refnum (for type only)=refnum<vi> refnum, vi path=w1134, options=128) -> (vi reference=w1132:refnum<vi>)  [unwired: 3 in, 1 out]
                n627 = call-by-ref "Start Asynchronous Call"(reference=w1132, "Y(mm)"=w1125, "X(mm)"=w1128) -> ()  [unwired: 10 in, 3 out]
              }
            }
            n628 = property on="currentNO" class="Str"("Val(Sgnl)"="B2") -> ()  [unwired: 2 in, 2 out]
          }
          event "B3": Value Change {
            n629 = event-data() -> ("NewVal"=w1140:bool)  [unwired: 1 in, 5 out]
            n630 = property on="移动" class="Bool (严格)"() -> ("Value"=w1143:bool)  [unwired: 2 in, 2 out]
            n631 = Not(x=w1143) -> (.not. x?=w1142:bool)
            n632 = And(x=w1142, y=w1140) -> (x .and. y?=w1141:bool)
            n633 = case shown="真" w1141 {
              frame False {
              }
              frame True {
                n634 = property on="A1-position-X" class="DigNum (严格)"() -> (error out=w1149:errorcluster, "Value"=w1156:dbl)  [unwired: 2 in, 1 out]
                n635 = property on="A1-position-Y" class="DigNum (严格)"(error in=w1149) -> (error out=w1148:errorcluster, "Value"=w1145:dbl)  [unwired: 1 in, 1 out]
                n636 = Subtract(x=w1145, y=4.5) -> (x-y=w1144:dbl)
                n637 = Subtract(x=w1156, y=9) -> (x-y=w1147:dbl)
                n638 = vi-ref "goto.vi"() -> (w1154:refnum<vi>)
                n639 = property class="VI"(reference=w1154, error in=w1148) -> ("Name"=w1153:string)  [unwired: 2 out]
                n640 = Open VI Reference(type specifier VI Refnum (for type only)=refnum<vi> refnum, vi path=w1153, options=128) -> (vi reference=w1151:refnum<vi>)  [unwired: 3 in, 1 out]
                n641 = call-by-ref "Start Asynchronous Call"(reference=w1151, "Y(mm)"=w1144, "X(mm)"=w1147) -> ()  [unwired: 10 in, 3 out]
              }
            }
            n642 = property on="currentNO" class="Str"("Val(Sgnl)"="B3") -> ()  [unwired: 2 in, 2 out]
          }
          event "B4": Value Change {
            n643 = event-data() -> ("NewVal"=w1159:bool)  [unwired: 1 in, 5 out]
            n644 = property on="移动" class="Bool (严格)"() -> ("Value"=w1162:bool)  [unwired: 2 in, 2 out]
            n645 = Not(x=w1162) -> (.not. x?=w1161:bool)
            n646 = And(x=w1161, y=w1159) -> (x .and. y?=w1160:bool)
            n647 = case shown="真" w1160 {
              frame False {
              }
              frame True {
                n648 = property on="A1-position-X" class="DigNum (严格)"() -> (error out=w1168:errorcluster, "Value"=w1175:dbl)  [unwired: 2 in, 1 out]
                n649 = property on="A1-position-Y" class="DigNum (严格)"(error in=w1168) -> (error out=w1167:errorcluster, "Value"=w1164:dbl)  [unwired: 1 in, 1 out]
                n650 = Subtract(x=w1164, y=4.5) -> (x-y=w1163:dbl)
                n651 = Subtract(x=w1175, y=13.5) -> (x-y=w1166:dbl)
                n652 = vi-ref "goto.vi"() -> (w1173:refnum<vi>)
                n653 = property class="VI"(reference=w1173, error in=w1167) -> ("Name"=w1172:string)  [unwired: 2 out]
                n654 = Open VI Reference(type specifier VI Refnum (for type only)=refnum<vi> refnum, vi path=w1172, options=128) -> (vi reference=w1170:refnum<vi>)  [unwired: 3 in, 1 out]
                n655 = call-by-ref "Start Asynchronous Call"(reference=w1170, "Y(mm)"=w1163, "X(mm)"=w1166) -> ()  [unwired: 10 in, 3 out]
              }
            }
            n656 = property on="currentNO" class="Str"("Val(Sgnl)"="B4") -> ()  [unwired: 2 in, 2 out]
          }
          event "B5": Value Change {
            n657 = event-data() -> ("NewVal"=w1178:bool)  [unwired: 1 in, 5 out]
            n658 = property on="移动" class="Bool (严格)"() -> ("Value"=w1181:bool)  [unwired: 2 in, 2 out]
            n659 = Not(x=w1181) -> (.not. x?=w1180:bool)
            n660 = And(x=w1180, y=w1178) -> (x .and. y?=w1179:bool)
            n661 = case shown="真" w1179 {
              frame False {
              }
              frame True {
                n662 = property on="A1-position-X" class="DigNum (严格)"() -> (error out=w1187:errorcluster, "Value"=w1194:dbl)  [unwired: 2 in, 1 out]
                n663 = property on="A1-position-Y" class="DigNum (严格)"(error in=w1187) -> (error out=w1186:errorcluster, "Value"=w1183:dbl)  [unwired: 1 in, 1 out]
                n664 = Subtract(x=w1183, y=4.5) -> (x-y=w1182:dbl)
                n665 = Subtract(x=w1194, y=18) -> (x-y=w1185:dbl)
                n666 = vi-ref "goto.vi"() -> (w1192:refnum<vi>)
                n667 = property class="VI"(reference=w1192, error in=w1186) -> ("Name"=w1191:string)  [unwired: 2 out]
                n668 = Open VI Reference(type specifier VI Refnum (for type only)=refnum<vi> refnum, vi path=w1191, options=128) -> (vi reference=w1189:refnum<vi>)  [unwired: 3 in, 1 out]
                n669 = call-by-ref "Start Asynchronous Call"(reference=w1189, "Y(mm)"=w1182, "X(mm)"=w1185) -> ()  [unwired: 10 in, 3 out]
              }
            }
            n670 = property on="currentNO" class="Str"("Val(Sgnl)"="B5") -> ()  [unwired: 2 in, 2 out]
          }
          event "B6": Value Change {
            n671 = event-data() -> ("NewVal"=w1197:bool)  [unwired: 1 in, 5 out]
            n672 = property on="移动" class="Bool (严格)"() -> ("Value"=w1200:bool)  [unwired: 2 in, 2 out]
            n673 = Not(x=w1200) -> (.not. x?=w1199:bool)
            n674 = And(x=w1199, y=w1197) -> (x .and. y?=w1198:bool)
            n675 = case shown="真" w1198 {
              frame False {
              }
              frame True {
                n676 = property on="A1-position-X" class="DigNum (严格)"() -> (error out=w1206:errorcluster, "Value"=w1213:dbl)  [unwired: 2 in, 1 out]
                n677 = property on="A1-position-Y" class="DigNum (严格)"(error in=w1206) -> (error out=w1205:errorcluster, "Value"=w1202:dbl)  [unwired: 1 in, 1 out]
                n678 = Subtract(x=w1202, y=4.5) -> (x-y=w1201:dbl)
                n679 = Subtract(x=w1213, y=22.5) -> (x-y=w1204:dbl)
                n680 = vi-ref "goto.vi"() -> (w1211:refnum<vi>)
                n681 = property class="VI"(reference=w1211, error in=w1205) -> ("Name"=w1210:string)  [unwired: 2 out]
                n682 = Open VI Reference(type specifier VI Refnum (for type only)=refnum<vi> refnum, vi path=w1210, options=128) -> (vi reference=w1208:refnum<vi>)  [unwired: 3 in, 1 out]
                n683 = call-by-ref "Start Asynchronous Call"(reference=w1208, "Y(mm)"=w1201, "X(mm)"=w1204) -> ()  [unwired: 10 in, 3 out]
              }
            }
            n684 = property on="currentNO" class="Str"("Val(Sgnl)"="B6") -> ()  [unwired: 2 in, 2 out]
          }
          event "B7": Value Change {
            n685 = event-data() -> ("NewVal"=w1216:bool)  [unwired: 1 in, 5 out]
            n686 = property on="移动" class="Bool (严格)"() -> ("Value"=w1219:bool)  [unwired: 2 in, 2 out]
            n687 = Not(x=w1219) -> (.not. x?=w1218:bool)
            n688 = And(x=w1218, y=w1216) -> (x .and. y?=w1217:bool)
            n689 = case shown="真" w1217 {
              frame False {
              }
              frame True {
                n690 = property on="A1-position-X" class="DigNum (严格)"() -> (error out=w1225:errorcluster, "Value"=w1232:dbl)  [unwired: 2 in, 1 out]
                n691 = property on="A1-position-Y" class="DigNum (严格)"(error in=w1225) -> (error out=w1224:errorcluster, "Value"=w1221:dbl)  [unwired: 1 in, 1 out]
                n692 = Subtract(x=w1221, y=4.5) -> (x-y=w1220:dbl)
                n693 = Subtract(x=w1232, y=27) -> (x-y=w1223:dbl)
                n694 = vi-ref "goto.vi"() -> (w1230:refnum<vi>)
                n695 = property class="VI"(reference=w1230, error in=w1224) -> ("Name"=w1229:string)  [unwired: 2 out]
                n696 = Open VI Reference(type specifier VI Refnum (for type only)=refnum<vi> refnum, vi path=w1229, options=128) -> (vi reference=w1227:refnum<vi>)  [unwired: 3 in, 1 out]
                n697 = call-by-ref "Start Asynchronous Call"(reference=w1227, "Y(mm)"=w1220, "X(mm)"=w1223) -> ()  [unwired: 10 in, 3 out]
              }
            }
            n698 = property on="currentNO" class="Str"("Val(Sgnl)"="B7") -> ()  [unwired: 2 in, 2 out]
          }
          event "B8": Value Change {
            n699 = event-data() -> ("NewVal"=w1235:bool)  [unwired: 1 in, 5 out]
            n700 = property on="移动" class="Bool (严格)"() -> ("Value"=w1238:bool)  [unwired: 2 in, 2 out]
            n701 = Not(x=w1238) -> (.not. x?=w1237:bool)
            n702 = And(x=w1237, y=w1235) -> (x .and. y?=w1236:bool)
            n703 = case shown="真" w1236 {
              frame False {
              }
              frame True {
                n704 = property on="A1-position-X" class="DigNum (严格)"() -> (error out=w1244:errorcluster, "Value"=w1251:dbl)  [unwired: 2 in, 1 out]
                n705 = property on="A1-position-Y" class="DigNum (严格)"(error in=w1244) -> (error out=w1243:errorcluster, "Value"=w1240:dbl)  [unwired: 1 in, 1 out]
                n706 = Subtract(x=w1240, y=4.5) -> (x-y=w1239:dbl)
                n707 = Subtract(x=w1251, y=31.5) -> (x-y=w1242:dbl)
                n708 = vi-ref "goto.vi"() -> (w1249:refnum<vi>)
                n709 = property class="VI"(reference=w1249, error in=w1243) -> ("Name"=w1248:string)  [unwired: 2 out]
                n710 = Open VI Reference(type specifier VI Refnum (for type only)=refnum<vi> refnum, vi path=w1248, options=128) -> (vi reference=w1246:refnum<vi>)  [unwired: 3 in, 1 out]
                n711 = call-by-ref "Start Asynchronous Call"(reference=w1246, "Y(mm)"=w1239, "X(mm)"=w1242) -> ()  [unwired: 10 in, 3 out]
              }
            }
            n712 = property on="currentNO" class="Str"("Val(Sgnl)"="B8") -> ()  [unwired: 2 in, 2 out]
          }
          event "B9": Value Change {
            n713 = event-data() -> ("NewVal"=w1254:bool)  [unwired: 1 in, 5 out]
            n714 = property on="移动" class="Bool (严格)"() -> ("Value"=w1257:bool)  [unwired: 2 in, 2 out]
            n715 = Not(x=w1257) -> (.not. x?=w1256:bool)
            n716 = And(x=w1256, y=w1254) -> (x .and. y?=w1255:bool)
            n717 = case shown="真" w1255 {
              frame False {
              }
              frame True {
                n718 = property on="A1-position-X" class="DigNum (严格)"() -> (error out=w1263:errorcluster, "Value"=w1270:dbl)  [unwired: 2 in, 1 out]
                n719 = property on="A1-position-Y" class="DigNum (严格)"(error in=w1263) -> (error out=w1262:errorcluster, "Value"=w1259:dbl)  [unwired: 1 in, 1 out]
                n720 = Subtract(x=w1259, y=4.5) -> (x-y=w1258:dbl)
                n721 = Subtract(x=w1270, y=36) -> (x-y=w1261:dbl)
                n722 = vi-ref "goto.vi"() -> (w1268:refnum<vi>)
                n723 = property class="VI"(reference=w1268, error in=w1262) -> ("Name"=w1267:string)  [unwired: 2 out]
                n724 = Open VI Reference(type specifier VI Refnum (for type only)=refnum<vi> refnum, vi path=w1267, options=128) -> (vi reference=w1265:refnum<vi>)  [unwired: 3 in, 1 out]
                n725 = call-by-ref "Start Asynchronous Call"(reference=w1265, "Y(mm)"=w1258, "X(mm)"=w1261) -> ()  [unwired: 10 in, 3 out]
              }
            }
            n726 = property on="currentNO" class="Str"("Val(Sgnl)"="B9") -> ()  [unwired: 2 in, 2 out]
          }
          event "B10": Value Change {
            n727 = event-data() -> ("NewVal"=w1273:bool)  [unwired: 1 in, 5 out]
            n728 = property on="移动" class="Bool (严格)"() -> ("Value"=w1276:bool)  [unwired: 2 in, 2 out]
            n729 = Not(x=w1276) -> (.not. x?=w1275:bool)
            n730 = And(x=w1275, y=w1273) -> (x .and. y?=w1274:bool)
            n731 = case shown="真" w1274 {
              frame False {
              }
              frame True {
                n732 = property on="A1-position-X" class="DigNum (严格)"() -> (error out=w1282:errorcluster, "Value"=w1289:dbl)  [unwired: 2 in, 1 out]
                n733 = property on="A1-position-Y" class="DigNum (严格)"(error in=w1282) -> (error out=w1281:errorcluster, "Value"=w1278:dbl)  [unwired: 1 in, 1 out]
                n734 = Subtract(x=w1278, y=4.5) -> (x-y=w1277:dbl)
                n735 = Subtract(x=w1289, y=40.5) -> (x-y=w1280:dbl)
                n736 = vi-ref "goto.vi"() -> (w1287:refnum<vi>)
                n737 = property class="VI"(reference=w1287, error in=w1281) -> ("Name"=w1286:string)  [unwired: 2 out]
                n738 = Open VI Reference(type specifier VI Refnum (for type only)=refnum<vi> refnum, vi path=w1286, options=128) -> (vi reference=w1284:refnum<vi>)  [unwired: 3 in, 1 out]
                n739 = call-by-ref "Start Asynchronous Call"(reference=w1284, "Y(mm)"=w1277, "X(mm)"=w1280) -> ()  [unwired: 10 in, 3 out]
              }
            }
            n740 = property on="currentNO" class="Str"("Val(Sgnl)"="B10") -> ()  [unwired: 2 in, 2 out]
          }
          event "B11": Value Change {
            n741 = event-data() -> ("NewVal"=w1292:bool)  [unwired: 1 in, 5 out]
            n742 = property on="移动" class="Bool (严格)"() -> ("Value"=w1295:bool)  [unwired: 2 in, 2 out]
            n743 = Not(x=w1295) -> (.not. x?=w1294:bool)
            n744 = And(x=w1294, y=w1292) -> (x .and. y?=w1293:bool)
            n745 = case shown="真" w1293 {
              frame False {
              }
              frame True {
                n746 = property on="A1-position-X" class="DigNum (严格)"() -> (error out=w1301:errorcluster, "Value"=w1308:dbl)  [unwired: 2 in, 1 out]
                n747 = property on="A1-position-Y" class="DigNum (严格)"(error in=w1301) -> (error out=w1300:errorcluster, "Value"=w1297:dbl)  [unwired: 1 in, 1 out]
                n748 = Subtract(x=w1297, y=4.5) -> (x-y=w1296:dbl)
                n749 = Subtract(x=w1308, y=45) -> (x-y=w1299:dbl)
                n750 = vi-ref "goto.vi"() -> (w1306:refnum<vi>)
                n751 = property class="VI"(reference=w1306, error in=w1300) -> ("Name"=w1305:string)  [unwired: 2 out]
                n752 = Open VI Reference(type specifier VI Refnum (for type only)=refnum<vi> refnum, vi path=w1305, options=128) -> (vi reference=w1303:refnum<vi>)  [unwired: 3 in, 1 out]
                n753 = call-by-ref "Start Asynchronous Call"(reference=w1303, "Y(mm)"=w1296, "X(mm)"=w1299) -> ()  [unwired: 10 in, 3 out]
              }
            }
            n754 = property on="currentNO" class="Str"("Val(Sgnl)"="B11") -> ()  [unwired: 2 in, 2 out]
          }
          event "B12": Value Change {
            n755 = event-data() -> ("NewVal"=w1311:bool)  [unwired: 1 in, 5 out]
            n756 = property on="移动" class="Bool (严格)"() -> ("Value"=w1314:bool)  [unwired: 2 in, 2 out]
            n757 = Not(x=w1314) -> (.not. x?=w1313:bool)
            n758 = And(x=w1313, y=w1311) -> (x .and. y?=w1312:bool)
            n759 = case shown="真" w1312 {
              frame False {
              }
              frame True {
                n760 = property on="A1-position-X" class="DigNum (严格)"() -> (error out=w1320:errorcluster, "Value"=w1327:dbl)  [unwired: 2 in, 1 out]
                n761 = property on="A1-position-Y" class="DigNum (严格)"(error in=w1320) -> (error out=w1319:errorcluster, "Value"=w1316:dbl)  [unwired: 1 in, 1 out]
                n762 = Subtract(x=w1316, y=4.5) -> (x-y=w1315:dbl)
                n763 = Subtract(x=w1327, y=49.5) -> (x-y=w1318:dbl)
                n764 = vi-ref "goto.vi"() -> (w1325:refnum<vi>)
                n765 = property class="VI"(reference=w1325, error in=w1319) -> ("Name"=w1324:string)  [unwired: 2 out]
                n766 = Open VI Reference(type specifier VI Refnum (for type only)=refnum<vi> refnum, vi path=w1324, options=128) -> (vi reference=w1322:refnum<vi>)  [unwired: 3 in, 1 out]
                n767 = call-by-ref "Start Asynchronous Call"(reference=w1322, "Y(mm)"=w1315, "X(mm)"=w1318) -> ()  [unwired: 10 in, 3 out]
              }
            }
            n768 = property on="currentNO" class="Str"("Val(Sgnl)"="B12") -> ()  [unwired: 2 in, 2 out]
          }
          event "C1": Value Change {
            n769 = event-data() -> ("NewVal"=w1330:bool)  [unwired: 1 in, 5 out]
            n770 = property on="移动" class="Bool (严格)"() -> ("Value"=w1333:bool)  [unwired: 2 in, 2 out]
            n771 = Not(x=w1333) -> (.not. x?=w1332:bool)
            n772 = And(x=w1332, y=w1330) -> (x .and. y?=w1331:bool)
            n773 = case shown="真" w1331 {
              frame False {
              }
              frame True {
                n774 = property on="A1-position-X" class="DigNum (严格)"() -> (error out=w1339:errorcluster, "Value"=w1346:dbl)  [unwired: 2 in, 1 out]
                n775 = property on="A1-position-Y" class="DigNum (严格)"(error in=w1339) -> (error out=w1338:errorcluster, "Value"=w1335:dbl)  [unwired: 1 in, 1 out]
                n776 = Subtract(x=w1335, y=9) -> (x-y=w1334:dbl)
                n777 = Subtract(x=w1346, y=0) -> (x-y=w1337:dbl)
                n778 = vi-ref "goto.vi"() -> (w1344:refnum<vi>)
                n779 = property class="VI"(reference=w1344, error in=w1338) -> ("Name"=w1343:string)  [unwired: 2 out]
                n780 = Open VI Reference(type specifier VI Refnum (for type only)=refnum<vi> refnum, vi path=w1343, options=128) -> (vi reference=w1341:refnum<vi>)  [unwired: 3 in, 1 out]
                n781 = call-by-ref "Start Asynchronous Call"(reference=w1341, "Y(mm)"=w1334, "X(mm)"=w1337) -> ()  [unwired: 10 in, 3 out]
              }
            }
            n782 = property on="currentNO" class="Str"("Val(Sgnl)"="C1") -> ()  [unwired: 2 in, 2 out]
          }
          event "C2": Value Change {
            n783 = event-data() -> ("NewVal"=w1349:bool)  [unwired: 1 in, 5 out]
            n784 = property on="移动" class="Bool (严格)"() -> ("Value"=w1352:bool)  [unwired: 2 in, 2 out]
            n785 = Not(x=w1352) -> (.not. x?=w1351:bool)
            n786 = And(x=w1351, y=w1349) -> (x .and. y?=w1350:bool)
            n787 = case shown="真" w1350 {
              frame False {
              }
              frame True {
                n788 = property on="A1-position-X" class="DigNum (严格)"() -> (error out=w1358:errorcluster, "Value"=w1365:dbl)  [unwired: 2 in, 1 out]
                n789 = property on="A1-position-Y" class="DigNum (严格)"(error in=w1358) -> (error out=w1357:errorcluster, "Value"=w1354:dbl)  [unwired: 1 in, 1 out]
                n790 = Subtract(x=w1354, y=9) -> (x-y=w1353:dbl)
                n791 = Subtract(x=w1365, y=4.5) -> (x-y=w1356:dbl)
                n792 = vi-ref "goto.vi"() -> (w1363:refnum<vi>)
                n793 = property class="VI"(reference=w1363, error in=w1357) -> ("Name"=w1362:string)  [unwired: 2 out]
                n794 = Open VI Reference(type specifier VI Refnum (for type only)=refnum<vi> refnum, vi path=w1362, options=128) -> (vi reference=w1360:refnum<vi>)  [unwired: 3 in, 1 out]
                n795 = call-by-ref "Start Asynchronous Call"(reference=w1360, "Y(mm)"=w1353, "X(mm)"=w1356) -> ()  [unwired: 10 in, 3 out]
              }
            }
            n796 = property on="currentNO" class="Str"("Val(Sgnl)"="C2") -> ()  [unwired: 2 in, 2 out]
          }
          event "C3": Value Change {
            n797 = event-data() -> ("NewVal"=w1368:bool)  [unwired: 1 in, 5 out]
            n798 = property on="移动" class="Bool (严格)"() -> ("Value"=w1371:bool)  [unwired: 2 in, 2 out]
            n799 = Not(x=w1371) -> (.not. x?=w1370:bool)
            n800 = And(x=w1370, y=w1368) -> (x .and. y?=w1369:bool)
            n801 = case shown="真" w1369 {
              frame False {
              }
              frame True {
                n802 = property on="A1-position-X" class="DigNum (严格)"() -> (error out=w1377:errorcluster, "Value"=w1384:dbl)  [unwired: 2 in, 1 out]
                n803 = property on="A1-position-Y" class="DigNum (严格)"(error in=w1377) -> (error out=w1376:errorcluster, "Value"=w1373:dbl)  [unwired: 1 in, 1 out]
                n804 = Subtract(x=w1373, y=9) -> (x-y=w1372:dbl)
                n805 = Subtract(x=w1384, y=9) -> (x-y=w1375:dbl)
                n806 = vi-ref "goto.vi"() -> (w1382:refnum<vi>)
                n807 = property class="VI"(reference=w1382, error in=w1376) -> ("Name"=w1381:string)  [unwired: 2 out]
                n808 = Open VI Reference(type specifier VI Refnum (for type only)=refnum<vi> refnum, vi path=w1381, options=128) -> (vi reference=w1379:refnum<vi>)  [unwired: 3 in, 1 out]
                n809 = call-by-ref "Start Asynchronous Call"(reference=w1379, "Y(mm)"=w1372, "X(mm)"=w1375) -> ()  [unwired: 10 in, 3 out]
              }
            }
            n810 = property on="currentNO" class="Str"("Val(Sgnl)"="C3") -> ()  [unwired: 2 in, 2 out]
          }
          event "C4": Value Change {
            n811 = event-data() -> ("NewVal"=w1387:bool)  [unwired: 1 in, 5 out]
            n812 = property on="移动" class="Bool (严格)"() -> ("Value"=w1390:bool)  [unwired: 2 in, 2 out]
            n813 = Not(x=w1390) -> (.not. x?=w1389:bool)
            n814 = And(x=w1389, y=w1387) -> (x .and. y?=w1388:bool)
            n815 = case shown="真" w1388 {
              frame False {
              }
              frame True {
                n816 = property on="A1-position-X" class="DigNum (严格)"() -> (error out=w1396:errorcluster, "Value"=w1403:dbl)  [unwired: 2 in, 1 out]
                n817 = property on="A1-position-Y" class="DigNum (严格)"(error in=w1396) -> (error out=w1395:errorcluster, "Value"=w1392:dbl)  [unwired: 1 in, 1 out]
                n818 = Subtract(x=w1392, y=9) -> (x-y=w1391:dbl)
                n819 = Subtract(x=w1403, y=13.5) -> (x-y=w1394:dbl)
                n820 = vi-ref "goto.vi"() -> (w1401:refnum<vi>)
                n821 = property class="VI"(reference=w1401, error in=w1395) -> ("Name"=w1400:string)  [unwired: 2 out]
                n822 = Open VI Reference(type specifier VI Refnum (for type only)=refnum<vi> refnum, vi path=w1400, options=128) -> (vi reference=w1398:refnum<vi>)  [unwired: 3 in, 1 out]
                n823 = call-by-ref "Start Asynchronous Call"(reference=w1398, "Y(mm)"=w1391, "X(mm)"=w1394) -> ()  [unwired: 10 in, 3 out]
              }
            }
            n824 = property on="currentNO" class="Str"("Val(Sgnl)"="C4") -> ()  [unwired: 2 in, 2 out]
          }
          event "C5": Value Change {
            n825 = event-data() -> ("NewVal"=w1406:bool)  [unwired: 1 in, 5 out]
            n826 = property on="移动" class="Bool (严格)"() -> ("Value"=w1409:bool)  [unwired: 2 in, 2 out]
            n827 = Not(x=w1409) -> (.not. x?=w1408:bool)
            n828 = And(x=w1408, y=w1406) -> (x .and. y?=w1407:bool)
            n829 = case shown="真" w1407 {
              frame False {
              }
              frame True {
                n830 = property on="A1-position-X" class="DigNum (严格)"() -> (error out=w1415:errorcluster, "Value"=w1422:dbl)  [unwired: 2 in, 1 out]
                n831 = property on="A1-position-Y" class="DigNum (严格)"(error in=w1415) -> (error out=w1414:errorcluster, "Value"=w1411:dbl)  [unwired: 1 in, 1 out]
                n832 = Subtract(x=w1411, y=9) -> (x-y=w1410:dbl)
                n833 = Subtract(x=w1422, y=18) -> (x-y=w1413:dbl)
                n834 = vi-ref "goto.vi"() -> (w1420:refnum<vi>)
                n835 = property class="VI"(reference=w1420, error in=w1414) -> ("Name"=w1419:string)  [unwired: 2 out]
                n836 = Open VI Reference(type specifier VI Refnum (for type only)=refnum<vi> refnum, vi path=w1419, options=128) -> (vi reference=w1417:refnum<vi>)  [unwired: 3 in, 1 out]
                n837 = call-by-ref "Start Asynchronous Call"(reference=w1417, "Y(mm)"=w1410, "X(mm)"=w1413) -> ()  [unwired: 10 in, 3 out]
              }
            }
            n838 = property on="currentNO" class="Str"("Val(Sgnl)"="C5") -> ()  [unwired: 2 in, 2 out]
          }
          event "C6": Value Change {
            n839 = event-data() -> ("NewVal"=w1425:bool)  [unwired: 1 in, 5 out]
            n840 = property on="移动" class="Bool (严格)"() -> ("Value"=w1428:bool)  [unwired: 2 in, 2 out]
            n841 = Not(x=w1428) -> (.not. x?=w1427:bool)
            n842 = And(x=w1427, y=w1425) -> (x .and. y?=w1426:bool)
            n843 = case shown="真" w1426 {
              frame False {
              }
              frame True {
                n844 = property on="A1-position-X" class="DigNum (严格)"() -> (error out=w1434:errorcluster, "Value"=w1441:dbl)  [unwired: 2 in, 1 out]
                n845 = property on="A1-position-Y" class="DigNum (严格)"(error in=w1434) -> (error out=w1433:errorcluster, "Value"=w1430:dbl)  [unwired: 1 in, 1 out]
                n846 = Subtract(x=w1430, y=9) -> (x-y=w1429:dbl)
                n847 = Subtract(x=w1441, y=22.5) -> (x-y=w1432:dbl)
                n848 = vi-ref "goto.vi"() -> (w1439:refnum<vi>)
                n849 = property class="VI"(reference=w1439, error in=w1433) -> ("Name"=w1438:string)  [unwired: 2 out]
                n850 = Open VI Reference(type specifier VI Refnum (for type only)=refnum<vi> refnum, vi path=w1438, options=128) -> (vi reference=w1436:refnum<vi>)  [unwired: 3 in, 1 out]
                n851 = call-by-ref "Start Asynchronous Call"(reference=w1436, "Y(mm)"=w1429, "X(mm)"=w1432) -> ()  [unwired: 10 in, 3 out]
              }
            }
            n852 = property on="currentNO" class="Str"("Val(Sgnl)"="C6") -> ()  [unwired: 2 in, 2 out]
          }
          event "C7": Value Change {
            n853 = event-data() -> ("NewVal"=w1444:bool)  [unwired: 1 in, 5 out]
            n854 = property on="移动" class="Bool (严格)"() -> ("Value"=w1447:bool)  [unwired: 2 in, 2 out]
            n855 = Not(x=w1447) -> (.not. x?=w1446:bool)
            n856 = And(x=w1446, y=w1444) -> (x .and. y?=w1445:bool)
            n857 = case shown="真" w1445 {
              frame False {
              }
              frame True {
                n858 = property on="A1-position-X" class="DigNum (严格)"() -> (error out=w1453:errorcluster, "Value"=w1460:dbl)  [unwired: 2 in, 1 out]
                n859 = property on="A1-position-Y" class="DigNum (严格)"(error in=w1453) -> (error out=w1452:errorcluster, "Value"=w1449:dbl)  [unwired: 1 in, 1 out]
                n860 = Subtract(x=w1449, y=9) -> (x-y=w1448:dbl)
                n861 = Subtract(x=w1460, y=27) -> (x-y=w1451:dbl)
                n862 = vi-ref "goto.vi"() -> (w1458:refnum<vi>)
                n863 = property class="VI"(reference=w1458, error in=w1452) -> ("Name"=w1457:string)  [unwired: 2 out]
                n864 = Open VI Reference(type specifier VI Refnum (for type only)=refnum<vi> refnum, vi path=w1457, options=128) -> (vi reference=w1455:refnum<vi>)  [unwired: 3 in, 1 out]
                n865 = call-by-ref "Start Asynchronous Call"(reference=w1455, "Y(mm)"=w1448, "X(mm)"=w1451) -> ()  [unwired: 10 in, 3 out]
              }
            }
            n866 = property on="currentNO" class="Str"("Val(Sgnl)"="C7") -> ()  [unwired: 2 in, 2 out]
          }
          event "C8": Value Change {
            n867 = event-data() -> ("NewVal"=w1463:bool)  [unwired: 1 in, 5 out]
            n868 = property on="移动" class="Bool (严格)"() -> ("Value"=w1466:bool)  [unwired: 2 in, 2 out]
            n869 = Not(x=w1466) -> (.not. x?=w1465:bool)
            n870 = And(x=w1465, y=w1463) -> (x .and. y?=w1464:bool)
            n871 = case shown="真" w1464 {
              frame False {
              }
              frame True {
                n872 = property on="A1-position-X" class="DigNum (严格)"() -> (error out=w1472:errorcluster, "Value"=w1479:dbl)  [unwired: 2 in, 1 out]
                n873 = property on="A1-position-Y" class="DigNum (严格)"(error in=w1472) -> (error out=w1471:errorcluster, "Value"=w1468:dbl)  [unwired: 1 in, 1 out]
                n874 = Subtract(x=w1468, y=9) -> (x-y=w1467:dbl)
                n875 = Subtract(x=w1479, y=31.5) -> (x-y=w1470:dbl)
                n876 = vi-ref "goto.vi"() -> (w1477:refnum<vi>)
                n877 = property class="VI"(reference=w1477, error in=w1471) -> ("Name"=w1476:string)  [unwired: 2 out]
                n878 = Open VI Reference(type specifier VI Refnum (for type only)=refnum<vi> refnum, vi path=w1476, options=128) -> (vi reference=w1474:refnum<vi>)  [unwired: 3 in, 1 out]
                n879 = call-by-ref "Start Asynchronous Call"(reference=w1474, "Y(mm)"=w1467, "X(mm)"=w1470) -> ()  [unwired: 10 in, 3 out]
              }
            }
            n880 = property on="currentNO" class="Str"("Val(Sgnl)"="C8") -> ()  [unwired: 2 in, 2 out]
          }
          event "C9": Value Change {
            n881 = event-data() -> ("NewVal"=w1482:bool)  [unwired: 1 in, 5 out]
            n882 = property on="移动" class="Bool (严格)"() -> ("Value"=w1485:bool)  [unwired: 2 in, 2 out]
            n883 = Not(x=w1485) -> (.not. x?=w1484:bool)
            n884 = And(x=w1484, y=w1482) -> (x .and. y?=w1483:bool)
            n885 = case shown="真" w1483 {
              frame False {
              }
              frame True {
                n886 = property on="A1-position-X" class="DigNum (严格)"() -> (error out=w1491:errorcluster, "Value"=w1498:dbl)  [unwired: 2 in, 1 out]
                n887 = property on="A1-position-Y" class="DigNum (严格)"(error in=w1491) -> (error out=w1490:errorcluster, "Value"=w1487:dbl)  [unwired: 1 in, 1 out]
                n888 = Subtract(x=w1487, y=9) -> (x-y=w1486:dbl)
                n889 = Subtract(x=w1498, y=36) -> (x-y=w1489:dbl)
                n890 = vi-ref "goto.vi"() -> (w1496:refnum<vi>)
                n891 = property class="VI"(reference=w1496, error in=w1490) -> ("Name"=w1495:string)  [unwired: 2 out]
                n892 = Open VI Reference(type specifier VI Refnum (for type only)=refnum<vi> refnum, vi path=w1495, options=128) -> (vi reference=w1493:refnum<vi>)  [unwired: 3 in, 1 out]
                n893 = call-by-ref "Start Asynchronous Call"(reference=w1493, "Y(mm)"=w1486, "X(mm)"=w1489) -> ()  [unwired: 10 in, 3 out]
              }
            }
            n894 = property on="currentNO" class="Str"("Val(Sgnl)"="C9") -> ()  [unwired: 2 in, 2 out]
          }
          event "C10": Value Change {
            n895 = event-data() -> ("NewVal"=w1501:bool)  [unwired: 1 in, 5 out]
            n896 = property on="移动" class="Bool (严格)"() -> ("Value"=w1504:bool)  [unwired: 2 in, 2 out]
            n897 = Not(x=w1504) -> (.not. x?=w1503:bool)
            n898 = And(x=w1503, y=w1501) -> (x .and. y?=w1502:bool)
            n899 = case shown="真" w1502 {
              frame False {
              }
              frame True {
                n900 = property on="A1-position-X" class="DigNum (严格)"() -> (error out=w1510:errorcluster, "Value"=w1517:dbl)  [unwired: 2 in, 1 out]
                n901 = property on="A1-position-Y" class="DigNum (严格)"(error in=w1510) -> (error out=w1509:errorcluster, "Value"=w1506:dbl)  [unwired: 1 in, 1 out]
                n902 = Subtract(x=w1506, y=9) -> (x-y=w1505:dbl)
                n903 = Subtract(x=w1517, y=40.5) -> (x-y=w1508:dbl)
                n904 = vi-ref "goto.vi"() -> (w1515:refnum<vi>)
                n905 = property class="VI"(reference=w1515, error in=w1509) -> ("Name"=w1514:string)  [unwired: 2 out]
                n906 = Open VI Reference(type specifier VI Refnum (for type only)=refnum<vi> refnum, vi path=w1514, options=128) -> (vi reference=w1512:refnum<vi>)  [unwired: 3 in, 1 out]
                n907 = call-by-ref "Start Asynchronous Call"(reference=w1512, "Y(mm)"=w1505, "X(mm)"=w1508) -> ()  [unwired: 10 in, 3 out]
              }
            }
            n908 = property on="currentNO" class="Str"("Val(Sgnl)"="C10") -> ()  [unwired: 2 in, 2 out]
          }
          event "C11": Value Change {
            n909 = event-data() -> ("NewVal"=w1520:bool)  [unwired: 1 in, 5 out]
            n910 = property on="移动" class="Bool (严格)"() -> ("Value"=w1523:bool)  [unwired: 2 in, 2 out]
            n911 = Not(x=w1523) -> (.not. x?=w1522:bool)
            n912 = And(x=w1522, y=w1520) -> (x .and. y?=w1521:bool)
            n913 = case shown="真" w1521 {
              frame False {
              }
              frame True {
                n914 = property on="A1-position-X" class="DigNum (严格)"() -> (error out=w1529:errorcluster, "Value"=w1536:dbl)  [unwired: 2 in, 1 out]
                n915 = property on="A1-position-Y" class="DigNum (严格)"(error in=w1529) -> (error out=w1528:errorcluster, "Value"=w1525:dbl)  [unwired: 1 in, 1 out]
                n916 = Subtract(x=w1525, y=9) -> (x-y=w1524:dbl)
                n917 = Subtract(x=w1536, y=45) -> (x-y=w1527:dbl)
                n918 = vi-ref "goto.vi"() -> (w1534:refnum<vi>)
                n919 = property class="VI"(reference=w1534, error in=w1528) -> ("Name"=w1533:string)  [unwired: 2 out]
                n920 = Open VI Reference(type specifier VI Refnum (for type only)=refnum<vi> refnum, vi path=w1533, options=128) -> (vi reference=w1531:refnum<vi>)  [unwired: 3 in, 1 out]
                n921 = call-by-ref "Start Asynchronous Call"(reference=w1531, "Y(mm)"=w1524, "X(mm)"=w1527) -> ()  [unwired: 10 in, 3 out]
              }
            }
            n922 = property on="currentNO" class="Str"("Val(Sgnl)"="C11") -> ()  [unwired: 2 in, 2 out]
          }
          event "C12": Value Change {
            n923 = event-data() -> ("NewVal"=w1539:bool)  [unwired: 1 in, 5 out]
            n924 = property on="移动" class="Bool (严格)"() -> ("Value"=w1542:bool)  [unwired: 2 in, 2 out]
            n925 = Not(x=w1542) -> (.not. x?=w1541:bool)
            n926 = And(x=w1541, y=w1539) -> (x .and. y?=w1540:bool)
            n927 = case shown="真" w1540 {
              frame False {
              }
              frame True {
                n928 = property on="A1-position-X" class="DigNum (严格)"() -> (error out=w1548:errorcluster, "Value"=w1555:dbl)  [unwired: 2 in, 1 out]
                n929 = property on="A1-position-Y" class="DigNum (严格)"(error in=w1548) -> (error out=w1547:errorcluster, "Value"=w1544:dbl)  [unwired: 1 in, 1 out]
                n930 = Subtract(x=w1544, y=9) -> (x-y=w1543:dbl)
                n931 = Subtract(x=w1555, y=49.5) -> (x-y=w1546:dbl)
                n932 = vi-ref "goto.vi"() -> (w1553:refnum<vi>)
                n933 = property class="VI"(reference=w1553, error in=w1547) -> ("Name"=w1552:string)  [unwired: 2 out]
                n934 = Open VI Reference(type specifier VI Refnum (for type only)=refnum<vi> refnum, vi path=w1552, options=128) -> (vi reference=w1550:refnum<vi>)  [unwired: 3 in, 1 out]
                n935 = call-by-ref "Start Asynchronous Call"(reference=w1550, "Y(mm)"=w1543, "X(mm)"=w1546) -> ()  [unwired: 10 in, 3 out]
              }
            }
            n936 = property on="currentNO" class="Str"("Val(Sgnl)"="C12") -> ()  [unwired: 2 in, 2 out]
          }
          event "D1": Value Change {
            n937 = event-data() -> ("NewVal"=w1558:bool)  [unwired: 1 in, 5 out]
            n938 = property on="移动" class="Bool (严格)"() -> ("Value"=w1561:bool)  [unwired: 2 in, 2 out]
            n939 = Not(x=w1561) -> (.not. x?=w1560:bool)
            n940 = And(x=w1560, y=w1558) -> (x .and. y?=w1559:bool)
            n941 = case shown="真" w1559 {
              frame False {
              }
              frame True {
                n942 = property on="A1-position-X" class="DigNum (严格)"() -> (error out=w1567:errorcluster, "Value"=w1574:dbl)  [unwired: 2 in, 1 out]
                n943 = property on="A1-position-Y" class="DigNum (严格)"(error in=w1567) -> (error out=w1566:errorcluster, "Value"=w1563:dbl)  [unwired: 1 in, 1 out]
                n944 = Subtract(x=w1563, y=13.5) -> (x-y=w1562:dbl)
                n945 = Subtract(x=w1574, y=0) -> (x-y=w1565:dbl)
                n946 = vi-ref "goto.vi"() -> (w1572:refnum<vi>)
                n947 = property class="VI"(reference=w1572, error in=w1566) -> ("Name"=w1571:string)  [unwired: 2 out]
                n948 = Open VI Reference(type specifier VI Refnum (for type only)=refnum<vi> refnum, vi path=w1571, options=128) -> (vi reference=w1569:refnum<vi>)  [unwired: 3 in, 1 out]
                n949 = call-by-ref "Start Asynchronous Call"(reference=w1569, "Y(mm)"=w1562, "X(mm)"=w1565) -> ()  [unwired: 10 in, 3 out]
              }
            }
            n950 = property on="currentNO" class="Str"("Val(Sgnl)"="D1") -> ()  [unwired: 2 in, 2 out]
          }
          event "D2": Value Change {
            n951 = event-data() -> ("NewVal"=w1577:bool)  [unwired: 1 in, 5 out]
            n952 = property on="移动" class="Bool (严格)"() -> ("Value"=w1580:bool)  [unwired: 2 in, 2 out]
            n953 = Not(x=w1580) -> (.not. x?=w1579:bool)
            n954 = And(x=w1579, y=w1577) -> (x .and. y?=w1578:bool)
            n955 = case shown="真" w1578 {
              frame False {
              }
              frame True {
                n956 = property on="A1-position-X" class="DigNum (严格)"() -> (error out=w1586:errorcluster, "Value"=w1593:dbl)  [unwired: 2 in, 1 out]
                n957 = property on="A1-position-Y" class="DigNum (严格)"(error in=w1586) -> (error out=w1585:errorcluster, "Value"=w1582:dbl)  [unwired: 1 in, 1 out]
                n958 = Subtract(x=w1582, y=13.5) -> (x-y=w1581:dbl)
                n959 = Subtract(x=w1593, y=4.5) -> (x-y=w1584:dbl)
                n960 = vi-ref "goto.vi"() -> (w1591:refnum<vi>)
                n961 = property class="VI"(reference=w1591, error in=w1585) -> ("Name"=w1590:string)  [unwired: 2 out]
                n962 = Open VI Reference(type specifier VI Refnum (for type only)=refnum<vi> refnum, vi path=w1590, options=128) -> (vi reference=w1588:refnum<vi>)  [unwired: 3 in, 1 out]
                n963 = call-by-ref "Start Asynchronous Call"(reference=w1588, "Y(mm)"=w1581, "X(mm)"=w1584) -> ()  [unwired: 10 in, 3 out]
              }
            }
            n964 = property on="currentNO" class="Str"("Val(Sgnl)"="D2") -> ()  [unwired: 2 in, 2 out]
          }
          event "D3": Value Change {
            n965 = event-data() -> ("NewVal"=w1596:bool)  [unwired: 1 in, 5 out]
            n966 = property on="移动" class="Bool (严格)"() -> ("Value"=w1599:bool)  [unwired: 2 in, 2 out]
            n967 = Not(x=w1599) -> (.not. x?=w1598:bool)
            n968 = And(x=w1598, y=w1596) -> (x .and. y?=w1597:bool)
            n969 = case shown="真" w1597 {
              frame False {
              }
              frame True {
                n970 = property on="A1-position-X" class="DigNum (严格)"() -> (error out=w1605:errorcluster, "Value"=w1612:dbl)  [unwired: 2 in, 1 out]
                n971 = property on="A1-position-Y" class="DigNum (严格)"(error in=w1605) -> (error out=w1604:errorcluster, "Value"=w1601:dbl)  [unwired: 1 in, 1 out]
                n972 = Subtract(x=w1601, y=13.5) -> (x-y=w1600:dbl)
                n973 = Subtract(x=w1612, y=9) -> (x-y=w1603:dbl)
                n974 = vi-ref "goto.vi"() -> (w1610:refnum<vi>)
                n975 = property class="VI"(reference=w1610, error in=w1604) -> ("Name"=w1609:string)  [unwired: 2 out]
                n976 = Open VI Reference(type specifier VI Refnum (for type only)=refnum<vi> refnum, vi path=w1609, options=128) -> (vi reference=w1607:refnum<vi>)  [unwired: 3 in, 1 out]
                n977 = call-by-ref "Start Asynchronous Call"(reference=w1607, "Y(mm)"=w1600, "X(mm)"=w1603) -> ()  [unwired: 10 in, 3 out]
              }
            }
            n978 = property on="currentNO" class="Str"("Val(Sgnl)"="D3") -> ()  [unwired: 2 in, 2 out]
          }
          event "D4": Value Change {
            n979 = event-data() -> ("NewVal"=w1615:bool)  [unwired: 1 in, 5 out]
            n980 = property on="移动" class="Bool (严格)"() -> ("Value"=w1618:bool)  [unwired: 2 in, 2 out]
            n981 = Not(x=w1618) -> (.not. x?=w1617:bool)
            n982 = And(x=w1617, y=w1615) -> (x .and. y?=w1616:bool)
            n983 = case shown="真" w1616 {
              frame False {
              }
              frame True {
                n984 = property on="A1-position-X" class="DigNum (严格)"() -> (error out=w1624:errorcluster, "Value"=w1631:dbl)  [unwired: 2 in, 1 out]
                n985 = property on="A1-position-Y" class="DigNum (严格)"(error in=w1624) -> (error out=w1623:errorcluster, "Value"=w1620:dbl)  [unwired: 1 in, 1 out]
                n986 = Subtract(x=w1620, y=13.5) -> (x-y=w1619:dbl)
                n987 = Subtract(x=w1631, y=13.5) -> (x-y=w1622:dbl)
                n988 = vi-ref "goto.vi"() -> (w1629:refnum<vi>)
                n989 = property class="VI"(reference=w1629, error in=w1623) -> ("Name"=w1628:string)  [unwired: 2 out]
                n990 = Open VI Reference(type specifier VI Refnum (for type only)=refnum<vi> refnum, vi path=w1628, options=128) -> (vi reference=w1626:refnum<vi>)  [unwired: 3 in, 1 out]
                n991 = call-by-ref "Start Asynchronous Call"(reference=w1626, "Y(mm)"=w1619, "X(mm)"=w1622) -> ()  [unwired: 10 in, 3 out]
              }
            }
            n992 = property on="currentNO" class="Str"("Val(Sgnl)"="D4") -> ()  [unwired: 2 in, 2 out]
          }
          event "D5": Value Change {
            n993 = event-data() -> ("NewVal"=w1634:bool)  [unwired: 1 in, 5 out]
            n994 = property on="移动" class="Bool (严格)"() -> ("Value"=w1637:bool)  [unwired: 2 in, 2 out]
            n995 = Not(x=w1637) -> (.not. x?=w1636:bool)
            n996 = And(x=w1636, y=w1634) -> (x .and. y?=w1635:bool)
            n997 = case shown="真" w1635 {
              frame False {
              }
              frame True {
                n998 = property on="A1-position-X" class="DigNum (严格)"() -> (error out=w1643:errorcluster, "Value"=w1650:dbl)  [unwired: 2 in, 1 out]
                n999 = property on="A1-position-Y" class="DigNum (严格)"(error in=w1643) -> (error out=w1642:errorcluster, "Value"=w1639:dbl)  [unwired: 1 in, 1 out]
                n1000 = Subtract(x=w1639, y=13.5) -> (x-y=w1638:dbl)
                n1001 = Subtract(x=w1650, y=18) -> (x-y=w1641:dbl)
                n1002 = vi-ref "goto.vi"() -> (w1648:refnum<vi>)
                n1003 = property class="VI"(reference=w1648, error in=w1642) -> ("Name"=w1647:string)  [unwired: 2 out]
                n1004 = Open VI Reference(type specifier VI Refnum (for type only)=refnum<vi> refnum, vi path=w1647, options=128) -> (vi reference=w1645:refnum<vi>)  [unwired: 3 in, 1 out]
                n1005 = call-by-ref "Start Asynchronous Call"(reference=w1645, "Y(mm)"=w1638, "X(mm)"=w1641) -> ()  [unwired: 10 in, 3 out]
              }
            }
            n1006 = property on="currentNO" class="Str"("Val(Sgnl)"="D5") -> ()  [unwired: 2 in, 2 out]
          }
          event "D6": Value Change {
            n1007 = event-data() -> ("NewVal"=w1653:bool)  [unwired: 1 in, 5 out]
            n1008 = property on="移动" class="Bool (严格)"() -> ("Value"=w1656:bool)  [unwired: 2 in, 2 out]
            n1009 = Not(x=w1656) -> (.not. x?=w1655:bool)
            n1010 = And(x=w1655, y=w1653) -> (x .and. y?=w1654:bool)
            n1011 = case shown="真" w1654 {
              frame False {
              }
              frame True {
                n1012 = property on="A1-position-X" class="DigNum (严格)"() -> (error out=w1662:errorcluster, "Value"=w1669:dbl)  [unwired: 2 in, 1 out]
                n1013 = property on="A1-position-Y" class="DigNum (严格)"(error in=w1662) -> (error out=w1661:errorcluster, "Value"=w1658:dbl)  [unwired: 1 in, 1 out]
                n1014 = Subtract(x=w1658, y=13.5) -> (x-y=w1657:dbl)
                n1015 = Subtract(x=w1669, y=22.5) -> (x-y=w1660:dbl)
                n1016 = vi-ref "goto.vi"() -> (w1667:refnum<vi>)
                n1017 = property class="VI"(reference=w1667, error in=w1661) -> ("Name"=w1666:string)  [unwired: 2 out]
                n1018 = Open VI Reference(type specifier VI Refnum (for type only)=refnum<vi> refnum, vi path=w1666, options=128) -> (vi reference=w1664:refnum<vi>)  [unwired: 3 in, 1 out]
                n1019 = call-by-ref "Start Asynchronous Call"(reference=w1664, "Y(mm)"=w1657, "X(mm)"=w1660) -> ()  [unwired: 10 in, 3 out]
              }
            }
            n1020 = property on="currentNO" class="Str"("Val(Sgnl)"="D6") -> ()  [unwired: 2 in, 2 out]
          }
          event "D7": Value Change {
            n1021 = event-data() -> ("NewVal"=w1672:bool)  [unwired: 1 in, 5 out]
            n1022 = property on="移动" class="Bool (严格)"() -> ("Value"=w1675:bool)  [unwired: 2 in, 2 out]
            n1023 = Not(x=w1675) -> (.not. x?=w1674:bool)
            n1024 = And(x=w1674, y=w1672) -> (x .and. y?=w1673:bool)
            n1025 = case shown="真" w1673 {
              frame False {
              }
              frame True {
                n1026 = property on="A1-position-X" class="DigNum (严格)"() -> (error out=w1681:errorcluster, "Value"=w1688:dbl)  [unwired: 2 in, 1 out]
                n1027 = property on="A1-position-Y" class="DigNum (严格)"(error in=w1681) -> (error out=w1680:errorcluster, "Value"=w1677:dbl)  [unwired: 1 in, 1 out]
                n1028 = Subtract(x=w1677, y=13.5) -> (x-y=w1676:dbl)
                n1029 = Subtract(x=w1688, y=27) -> (x-y=w1679:dbl)
                n1030 = vi-ref "goto.vi"() -> (w1686:refnum<vi>)
                n1031 = property class="VI"(reference=w1686, error in=w1680) -> ("Name"=w1685:string)  [unwired: 2 out]
                n1032 = Open VI Reference(type specifier VI Refnum (for type only)=refnum<vi> refnum, vi path=w1685, options=128) -> (vi reference=w1683:refnum<vi>)  [unwired: 3 in, 1 out]
                n1033 = call-by-ref "Start Asynchronous Call"(reference=w1683, "Y(mm)"=w1676, "X(mm)"=w1679) -> ()  [unwired: 10 in, 3 out]
              }
            }
            n1034 = property on="currentNO" class="Str"("Val(Sgnl)"="D7") -> ()  [unwired: 2 in, 2 out]
          }
          event "D8": Value Change {
            n1035 = event-data() -> ("NewVal"=w1690:bool)  [unwired: 1 in, 5 out]
            n1036 = property on="移动" class="Bool (严格)"() -> ("Value"=w1693:bool)  [unwired: 2 in, 2 out]
            n1037 = Not(x=w1693) -> (.not. x?=w1692:bool)
            n1038 = And(x=w1692, y=w1690) -> (x .and. y?=w1691:bool)
            n1039 = case shown="真" w1691 {
              frame False {
              }
              frame True {
                n1040 = property on="A1-position-X" class="DigNum (严格)"() -> (error out=w1700:errorcluster, "Value"=w1707:dbl)  [unwired: 2 in, 1 out]
                n1041 = property on="A1-position-Y" class="DigNum (严格)"(error in=w1700) -> (error out=w1699:errorcluster, "Value"=w1696:dbl)  [unwired: 1 in, 1 out]
                n1042 = Subtract(x=w1696, y=13.5) -> (x-y=w1695:dbl)
                n1043 = Subtract(x=w1707, y=31.5) -> (x-y=w1698:dbl)
                n1044 = vi-ref "goto.vi"() -> (w1705:refnum<vi>)
                n1045 = property class="VI"(reference=w1705, error in=w1699) -> ("Name"=w1704:string)  [unwired: 2 out]
                n1046 = Open VI Reference(type specifier VI Refnum (for type only)=refnum<vi> refnum, vi path=w1704, options=128) -> (vi reference=w1702:refnum<vi>)  [unwired: 3 in, 1 out]
                n1047 = call-by-ref "Start Asynchronous Call"(reference=w1702, "Y(mm)"=w1695, "X(mm)"=w1698) -> ()  [unwired: 10 in, 3 out]
              }
            }
            n1048 = property on="currentNO" class="Str"("Val(Sgnl)"="D8") -> ()  [unwired: 2 in, 2 out]
          }
          event "D9": Value Change {
            n1049 = event-data() -> ("NewVal"=w1709:bool)  [unwired: 1 in, 5 out]
            n1050 = property on="移动" class="Bool (严格)"() -> ("Value"=w1712:bool)  [unwired: 2 in, 2 out]
            n1051 = Not(x=w1712) -> (.not. x?=w1711:bool)
            n1052 = And(x=w1711, y=w1709) -> (x .and. y?=w1710:bool)
            n1053 = case shown="真" w1710 {
              frame False {
              }
              frame True {
                n1054 = property on="A1-position-X" class="DigNum (严格)"() -> (error out=w1719:errorcluster, "Value"=w1726:dbl)  [unwired: 2 in, 1 out]
                n1055 = property on="A1-position-Y" class="DigNum (严格)"(error in=w1719) -> (error out=w1718:errorcluster, "Value"=w1715:dbl)  [unwired: 1 in, 1 out]
                n1056 = Subtract(x=w1715, y=13.5) -> (x-y=w1714:dbl)
                n1057 = Subtract(x=w1726, y=36) -> (x-y=w1717:dbl)
                n1058 = vi-ref "goto.vi"() -> (w1724:refnum<vi>)
                n1059 = property class="VI"(reference=w1724, error in=w1718) -> ("Name"=w1723:string)  [unwired: 2 out]
                n1060 = Open VI Reference(type specifier VI Refnum (for type only)=refnum<vi> refnum, vi path=w1723, options=128) -> (vi reference=w1721:refnum<vi>)  [unwired: 3 in, 1 out]
                n1061 = call-by-ref "Start Asynchronous Call"(reference=w1721, "Y(mm)"=w1714, "X(mm)"=w1717) -> ()  [unwired: 10 in, 3 out]
              }
            }
            n1062 = property on="currentNO" class="Str"("Val(Sgnl)"="D9") -> ()  [unwired: 2 in, 2 out]
          }
          event "D10": Value Change {
            n1063 = event-data() -> ("NewVal"=w1728:bool)  [unwired: 1 in, 5 out]
            n1064 = property on="移动" class="Bool (严格)"() -> ("Value"=w1731:bool)  [unwired: 2 in, 2 out]
            n1065 = Not(x=w1731) -> (.not. x?=w1730:bool)
            n1066 = And(x=w1730, y=w1728) -> (x .and. y?=w1729:bool)
            n1067 = case shown="真" w1729 {
              frame False {
              }
              frame True {
                n1068 = property on="A1-position-X" class="DigNum (严格)"() -> (error out=w1738:errorcluster, "Value"=w1745:dbl)  [unwired: 2 in, 1 out]
                n1069 = property on="A1-position-Y" class="DigNum (严格)"(error in=w1738) -> (error out=w1737:errorcluster, "Value"=w1734:dbl)  [unwired: 1 in, 1 out]
                n1070 = Subtract(x=w1734, y=13.5) -> (x-y=w1733:dbl)
                n1071 = Subtract(x=w1745, y=40.5) -> (x-y=w1736:dbl)
                n1072 = vi-ref "goto.vi"() -> (w1743:refnum<vi>)
                n1073 = property class="VI"(reference=w1743, error in=w1737) -> ("Name"=w1742:string)  [unwired: 2 out]
                n1074 = Open VI Reference(type specifier VI Refnum (for type only)=refnum<vi> refnum, vi path=w1742, options=128) -> (vi reference=w1740:refnum<vi>)  [unwired: 3 in, 1 out]
                n1075 = call-by-ref "Start Asynchronous Call"(reference=w1740, "Y(mm)"=w1733, "X(mm)"=w1736) -> ()  [unwired: 10 in, 3 out]
              }
            }
            n1076 = property on="currentNO" class="Str"("Val(Sgnl)"="D10") -> ()  [unwired: 2 in, 2 out]
          }
          event "D11": Value Change {
            n1077 = event-data() -> ("NewVal"=w1747:bool)  [unwired: 1 in, 5 out]
            n1078 = property on="移动" class="Bool (严格)"() -> ("Value"=w1750:bool)  [unwired: 2 in, 2 out]
            n1079 = Not(x=w1750) -> (.not. x?=w1749:bool)
            n1080 = And(x=w1749, y=w1747) -> (x .and. y?=w1748:bool)
            n1081 = case shown="真" w1748 {
              frame False {
              }
              frame True {
                n1082 = property on="A1-position-X" class="DigNum (严格)"() -> (error out=w1757:errorcluster, "Value"=w1764:dbl)  [unwired: 2 in, 1 out]
                n1083 = property on="A1-position-Y" class="DigNum (严格)"(error in=w1757) -> (error out=w1756:errorcluster, "Value"=w1753:dbl)  [unwired: 1 in, 1 out]
                n1084 = Subtract(x=w1753, y=13.5) -> (x-y=w1752:dbl)
                n1085 = Subtract(x=w1764, y=45) -> (x-y=w1755:dbl)
                n1086 = vi-ref "goto.vi"() -> (w1762:refnum<vi>)
                n1087 = property class="VI"(reference=w1762, error in=w1756) -> ("Name"=w1761:string)  [unwired: 2 out]
                n1088 = Open VI Reference(type specifier VI Refnum (for type only)=refnum<vi> refnum, vi path=w1761, options=128) -> (vi reference=w1759:refnum<vi>)  [unwired: 3 in, 1 out]
                n1089 = call-by-ref "Start Asynchronous Call"(reference=w1759, "Y(mm)"=w1752, "X(mm)"=w1755) -> ()  [unwired: 10 in, 3 out]
              }
            }
            n1090 = property on="currentNO" class="Str"("Val(Sgnl)"="D11") -> ()  [unwired: 2 in, 2 out]
          }
          event "D12": Value Change {
            n1091 = event-data() -> ("NewVal"=w1766:bool)  [unwired: 1 in, 5 out]
            n1092 = property on="移动" class="Bool (严格)"() -> ("Value"=w1769:bool)  [unwired: 2 in, 2 out]
            n1093 = Not(x=w1769) -> (.not. x?=w1768:bool)
            n1094 = And(x=w1768, y=w1766) -> (x .and. y?=w1767:bool)
            n1095 = case shown="真" w1767 {
              frame False {
              }
              frame True {
                n1096 = property on="A1-position-X" class="DigNum (严格)"() -> (error out=w1776:errorcluster, "Value"=w1783:dbl)  [unwired: 2 in, 1 out]
                n1097 = property on="A1-position-Y" class="DigNum (严格)"(error in=w1776) -> (error out=w1775:errorcluster, "Value"=w1772:dbl)  [unwired: 1 in, 1 out]
                n1098 = Subtract(x=w1772, y=13.5) -> (x-y=w1771:dbl)
                n1099 = Subtract(x=w1783, y=49.5) -> (x-y=w1774:dbl)
                n1100 = vi-ref "goto.vi"() -> (w1781:refnum<vi>)
                n1101 = property class="VI"(reference=w1781, error in=w1775) -> ("Name"=w1780:string)  [unwired: 2 out]
                n1102 = Open VI Reference(type specifier VI Refnum (for type only)=refnum<vi> refnum, vi path=w1780, options=128) -> (vi reference=w1778:refnum<vi>)  [unwired: 3 in, 1 out]
                n1103 = call-by-ref "Start Asynchronous Call"(reference=w1778, "Y(mm)"=w1771, "X(mm)"=w1774) -> ()  [unwired: 10 in, 3 out]
              }
            }
            n1104 = property on="currentNO" class="Str"("Val(Sgnl)"="D12") -> ()  [unwired: 2 in, 2 out]
          }
          event "E1": Value Change {
            n1105 = event-data() -> ("NewVal"=w1785:bool)  [unwired: 1 in, 5 out]
            n1106 = property on="移动" class="Bool (严格)"() -> ("Value"=w1788:bool)  [unwired: 2 in, 2 out]
            n1107 = Not(x=w1788) -> (.not. x?=w1787:bool)
            n1108 = And(x=w1787, y=w1785) -> (x .and. y?=w1786:bool)
            n1109 = case shown="真" w1786 {
              frame False {
              }
              frame True {
                n1110 = property on="A1-position-X" class="DigNum (严格)"() -> (error out=w1795:errorcluster, "Value"=w1802:dbl)  [unwired: 2 in, 1 out]
                n1111 = property on="A1-position-Y" class="DigNum (严格)"(error in=w1795) -> (error out=w1794:errorcluster, "Value"=w1791:dbl)  [unwired: 1 in, 1 out]
                n1112 = Subtract(x=w1791, y=18.0) -> (x-y=w1790:dbl)
                n1113 = Subtract(x=w1802, y=0) -> (x-y=w1793:dbl)
                n1114 = vi-ref "goto.vi"() -> (w1800:refnum<vi>)
                n1115 = property class="VI"(reference=w1800, error in=w1794) -> ("Name"=w1799:string)  [unwired: 2 out]
                n1116 = Open VI Reference(type specifier VI Refnum (for type only)=refnum<vi> refnum, vi path=w1799, options=128) -> (vi reference=w1797:refnum<vi>)  [unwired: 3 in, 1 out]
                n1117 = call-by-ref "Start Asynchronous Call"(reference=w1797, "Y(mm)"=w1790, "X(mm)"=w1793) -> ()  [unwired: 10 in, 3 out]
              }
            }
            n1118 = property on="currentNO" class="Str"("Val(Sgnl)"="E1") -> ()  [unwired: 2 in, 2 out]
          }
          event "E2": Value Change {
            n1119 = event-data() -> ("NewVal"=w1804:bool)  [unwired: 1 in, 5 out]
            n1120 = property on="移动" class="Bool (严格)"() -> ("Value"=w1807:bool)  [unwired: 2 in, 2 out]
            n1121 = Not(x=w1807) -> (.not. x?=w1806:bool)
            n1122 = And(x=w1806, y=w1804) -> (x .and. y?=w1805:bool)
            n1123 = case shown="真" w1805 {
              frame False {
              }
              frame True {
                n1124 = property on="A1-position-X" class="DigNum (严格)"() -> (error out=w1814:errorcluster, "Value"=w1821:dbl)  [unwired: 2 in, 1 out]
                n1125 = property on="A1-position-Y" class="DigNum (严格)"(error in=w1814) -> (error out=w1813:errorcluster, "Value"=w1810:dbl)  [unwired: 1 in, 1 out]
                n1126 = Subtract(x=w1810, y=18.0) -> (x-y=w1809:dbl)
                n1127 = Subtract(x=w1821, y=4.5) -> (x-y=w1812:dbl)
                n1128 = vi-ref "goto.vi"() -> (w1819:refnum<vi>)
                n1129 = property class="VI"(reference=w1819, error in=w1813) -> ("Name"=w1818:string)  [unwired: 2 out]
                n1130 = Open VI Reference(type specifier VI Refnum (for type only)=refnum<vi> refnum, vi path=w1818, options=128) -> (vi reference=w1816:refnum<vi>)  [unwired: 3 in, 1 out]
                n1131 = call-by-ref "Start Asynchronous Call"(reference=w1816, "Y(mm)"=w1809, "X(mm)"=w1812) -> ()  [unwired: 10 in, 3 out]
              }
            }
            n1132 = property on="currentNO" class="Str"("Val(Sgnl)"="E2") -> ()  [unwired: 2 in, 2 out]
          }
          event "E3": Value Change {
            n1133 = event-data() -> ("NewVal"=w1823:bool)  [unwired: 1 in, 5 out]
            n1134 = property on="移动" class="Bool (严格)"() -> ("Value"=w1826:bool)  [unwired: 2 in, 2 out]
            n1135 = Not(x=w1826) -> (.not. x?=w1825:bool)
            n1136 = And(x=w1825, y=w1823) -> (x .and. y?=w1824:bool)
            n1137 = case shown="真" w1824 {
              frame False {
              }
              frame True {
                n1138 = property on="A1-position-X" class="DigNum (严格)"() -> (error out=w1833:errorcluster, "Value"=w1840:dbl)  [unwired: 2 in, 1 out]
                n1139 = property on="A1-position-Y" class="DigNum (严格)"(error in=w1833) -> (error out=w1832:errorcluster, "Value"=w1829:dbl)  [unwired: 1 in, 1 out]
                n1140 = Subtract(x=w1829, y=18.0) -> (x-y=w1828:dbl)
                n1141 = Subtract(x=w1840, y=9) -> (x-y=w1831:dbl)
                n1142 = vi-ref "goto.vi"() -> (w1838:refnum<vi>)
                n1143 = property class="VI"(reference=w1838, error in=w1832) -> ("Name"=w1837:string)  [unwired: 2 out]
                n1144 = Open VI Reference(type specifier VI Refnum (for type only)=refnum<vi> refnum, vi path=w1837, options=128) -> (vi reference=w1835:refnum<vi>)  [unwired: 3 in, 1 out]
                n1145 = call-by-ref "Start Asynchronous Call"(reference=w1835, "Y(mm)"=w1828, "X(mm)"=w1831) -> ()  [unwired: 10 in, 3 out]
              }
            }
            n1146 = property on="currentNO" class="Str"("Val(Sgnl)"="E3") -> ()  [unwired: 2 in, 2 out]
          }
          event "E4": Value Change {
            n1147 = event-data() -> ("NewVal"=w1842:bool)  [unwired: 1 in, 5 out]
            n1148 = property on="移动" class="Bool (严格)"() -> ("Value"=w1845:bool)  [unwired: 2 in, 2 out]
            n1149 = Not(x=w1845) -> (.not. x?=w1844:bool)
            n1150 = And(x=w1844, y=w1842) -> (x .and. y?=w1843:bool)
            n1151 = case shown="真" w1843 {
              frame False {
              }
              frame True {
                n1152 = property on="A1-position-X" class="DigNum (严格)"() -> (error out=w1852:errorcluster, "Value"=w1859:dbl)  [unwired: 2 in, 1 out]
                n1153 = property on="A1-position-Y" class="DigNum (严格)"(error in=w1852) -> (error out=w1851:errorcluster, "Value"=w1848:dbl)  [unwired: 1 in, 1 out]
                n1154 = Subtract(x=w1848, y=18.0) -> (x-y=w1847:dbl)
                n1155 = Subtract(x=w1859, y=13.5) -> (x-y=w1850:dbl)
                n1156 = vi-ref "goto.vi"() -> (w1857:refnum<vi>)
                n1157 = property class="VI"(reference=w1857, error in=w1851) -> ("Name"=w1856:string)  [unwired: 2 out]
                n1158 = Open VI Reference(type specifier VI Refnum (for type only)=refnum<vi> refnum, vi path=w1856, options=128) -> (vi reference=w1854:refnum<vi>)  [unwired: 3 in, 1 out]
                n1159 = call-by-ref "Start Asynchronous Call"(reference=w1854, "Y(mm)"=w1847, "X(mm)"=w1850) -> ()  [unwired: 10 in, 3 out]
              }
            }
            n1160 = property on="currentNO" class="Str"("Val(Sgnl)"="E4") -> ()  [unwired: 2 in, 2 out]
          }
          event "E5": Value Change {
            n1161 = event-data() -> ("NewVal"=w1861:bool)  [unwired: 1 in, 5 out]
            n1162 = property on="移动" class="Bool (严格)"() -> ("Value"=w1864:bool)  [unwired: 2 in, 2 out]
            n1163 = Not(x=w1864) -> (.not. x?=w1863:bool)
            n1164 = And(x=w1863, y=w1861) -> (x .and. y?=w1862:bool)
            n1165 = case shown="真" w1862 {
              frame False {
              }
              frame True {
                n1166 = property on="A1-position-X" class="DigNum (严格)"() -> (error out=w1871:errorcluster, "Value"=w1878:dbl)  [unwired: 2 in, 1 out]
                n1167 = property on="A1-position-Y" class="DigNum (严格)"(error in=w1871) -> (error out=w1870:errorcluster, "Value"=w1867:dbl)  [unwired: 1 in, 1 out]
                n1168 = Subtract(x=w1867, y=18.0) -> (x-y=w1866:dbl)
                n1169 = Subtract(x=w1878, y=18) -> (x-y=w1869:dbl)
                n1170 = vi-ref "goto.vi"() -> (w1876:refnum<vi>)
                n1171 = property class="VI"(reference=w1876, error in=w1870) -> ("Name"=w1875:string)  [unwired: 2 out]
                n1172 = Open VI Reference(type specifier VI Refnum (for type only)=refnum<vi> refnum, vi path=w1875, options=128) -> (vi reference=w1873:refnum<vi>)  [unwired: 3 in, 1 out]
                n1173 = call-by-ref "Start Asynchronous Call"(reference=w1873, "Y(mm)"=w1866, "X(mm)"=w1869) -> ()  [unwired: 10 in, 3 out]
              }
            }
            n1174 = property on="currentNO" class="Str"("Val(Sgnl)"="E5") -> ()  [unwired: 2 in, 2 out]
          }
          event "E6": Value Change {
            n1175 = event-data() -> ("NewVal"=w1880:bool)  [unwired: 1 in, 5 out]
            n1176 = property on="移动" class="Bool (严格)"() -> ("Value"=w1883:bool)  [unwired: 2 in, 2 out]
            n1177 = Not(x=w1883) -> (.not. x?=w1882:bool)
            n1178 = And(x=w1882, y=w1880) -> (x .and. y?=w1881:bool)
            n1179 = case shown="真" w1881 {
              frame False {
              }
              frame True {
                n1180 = property on="A1-position-X" class="DigNum (严格)"() -> (error out=w1890:errorcluster, "Value"=w1897:dbl)  [unwired: 2 in, 1 out]
                n1181 = property on="A1-position-Y" class="DigNum (严格)"(error in=w1890) -> (error out=w1889:errorcluster, "Value"=w1886:dbl)  [unwired: 1 in, 1 out]
                n1182 = Subtract(x=w1886, y=18.0) -> (x-y=w1885:dbl)
                n1183 = Subtract(x=w1897, y=22.5) -> (x-y=w1888:dbl)
                n1184 = vi-ref "goto.vi"() -> (w1895:refnum<vi>)
                n1185 = property class="VI"(reference=w1895, error in=w1889) -> ("Name"=w1894:string)  [unwired: 2 out]
                n1186 = Open VI Reference(type specifier VI Refnum (for type only)=refnum<vi> refnum, vi path=w1894, options=128) -> (vi reference=w1892:refnum<vi>)  [unwired: 3 in, 1 out]
                n1187 = call-by-ref "Start Asynchronous Call"(reference=w1892, "Y(mm)"=w1885, "X(mm)"=w1888) -> ()  [unwired: 10 in, 3 out]
              }
            }
            n1188 = property on="currentNO" class="Str"("Val(Sgnl)"="E6") -> ()  [unwired: 2 in, 2 out]
          }
          event "E7": Value Change {
            n1189 = event-data() -> ("NewVal"=w1899:bool)  [unwired: 1 in, 5 out]
            n1190 = property on="移动" class="Bool (严格)"() -> ("Value"=w1902:bool)  [unwired: 2 in, 2 out]
            n1191 = Not(x=w1902) -> (.not. x?=w1901:bool)
            n1192 = And(x=w1901, y=w1899) -> (x .and. y?=w1900:bool)
            n1193 = case shown="真" w1900 {
              frame False {
              }
              frame True {
                n1194 = property on="A1-position-X" class="DigNum (严格)"() -> (error out=w1909:errorcluster, "Value"=w1916:dbl)  [unwired: 2 in, 1 out]
                n1195 = property on="A1-position-Y" class="DigNum (严格)"(error in=w1909) -> (error out=w1908:errorcluster, "Value"=w1905:dbl)  [unwired: 1 in, 1 out]
                n1196 = Subtract(x=w1905, y=18.0) -> (x-y=w1904:dbl)
                n1197 = Subtract(x=w1916, y=27) -> (x-y=w1907:dbl)
                n1198 = vi-ref "goto.vi"() -> (w1914:refnum<vi>)
                n1199 = property class="VI"(reference=w1914, error in=w1908) -> ("Name"=w1913:string)  [unwired: 2 out]
                n1200 = Open VI Reference(type specifier VI Refnum (for type only)=refnum<vi> refnum, vi path=w1913, options=128) -> (vi reference=w1911:refnum<vi>)  [unwired: 3 in, 1 out]
                n1201 = call-by-ref "Start Asynchronous Call"(reference=w1911, "Y(mm)"=w1904, "X(mm)"=w1907) -> ()  [unwired: 10 in, 3 out]
              }
            }
            n1202 = property on="currentNO" class="Str"("Val(Sgnl)"="E7") -> ()  [unwired: 2 in, 2 out]
          }
          event "E8": Value Change {
            n1203 = event-data() -> ("NewVal"=w1918:bool)  [unwired: 1 in, 5 out]
            n1204 = property on="移动" class="Bool (严格)"() -> ("Value"=w1921:bool)  [unwired: 2 in, 2 out]
            n1205 = Not(x=w1921) -> (.not. x?=w1920:bool)
            n1206 = And(x=w1920, y=w1918) -> (x .and. y?=w1919:bool)
            n1207 = case shown="真" w1919 {
              frame False {
              }
              frame True {
                n1208 = property on="A1-position-X" class="DigNum (严格)"() -> (error out=w1928:errorcluster, "Value"=w1935:dbl)  [unwired: 2 in, 1 out]
                n1209 = property on="A1-position-Y" class="DigNum (严格)"(error in=w1928) -> (error out=w1927:errorcluster, "Value"=w1924:dbl)  [unwired: 1 in, 1 out]
                n1210 = Subtract(x=w1924, y=18.0) -> (x-y=w1923:dbl)
                n1211 = Subtract(x=w1935, y=31.5) -> (x-y=w1926:dbl)
                n1212 = vi-ref "goto.vi"() -> (w1933:refnum<vi>)
                n1213 = property class="VI"(reference=w1933, error in=w1927) -> ("Name"=w1932:string)  [unwired: 2 out]
                n1214 = Open VI Reference(type specifier VI Refnum (for type only)=refnum<vi> refnum, vi path=w1932, options=128) -> (vi reference=w1930:refnum<vi>)  [unwired: 3 in, 1 out]
                n1215 = call-by-ref "Start Asynchronous Call"(reference=w1930, "Y(mm)"=w1923, "X(mm)"=w1926) -> ()  [unwired: 10 in, 3 out]
              }
            }
            n1216 = property on="currentNO" class="Str"("Val(Sgnl)"="E8") -> ()  [unwired: 2 in, 2 out]
          }
          event "E9": Value Change {
            n1217 = event-data() -> ("NewVal"=w1937:bool)  [unwired: 1 in, 5 out]
            n1218 = property on="移动" class="Bool (严格)"() -> ("Value"=w1940:bool)  [unwired: 2 in, 2 out]
            n1219 = Not(x=w1940) -> (.not. x?=w1939:bool)
            n1220 = And(x=w1939, y=w1937) -> (x .and. y?=w1938:bool)
            n1221 = case shown="真" w1938 {
              frame False {
              }
              frame True {
                n1222 = property on="A1-position-X" class="DigNum (严格)"() -> (error out=w1947:errorcluster, "Value"=w1954:dbl)  [unwired: 2 in, 1 out]
                n1223 = property on="A1-position-Y" class="DigNum (严格)"(error in=w1947) -> (error out=w1946:errorcluster, "Value"=w1943:dbl)  [unwired: 1 in, 1 out]
                n1224 = Subtract(x=w1943, y=18.0) -> (x-y=w1942:dbl)
                n1225 = Subtract(x=w1954, y=36.0) -> (x-y=w1945:dbl)
                n1226 = vi-ref "goto.vi"() -> (w1952:refnum<vi>)
                n1227 = property class="VI"(reference=w1952, error in=w1946) -> ("Name"=w1951:string)  [unwired: 2 out]
                n1228 = Open VI Reference(type specifier VI Refnum (for type only)=refnum<vi> refnum, vi path=w1951, options=128) -> (vi reference=w1949:refnum<vi>)  [unwired: 3 in, 1 out]
                n1229 = call-by-ref "Start Asynchronous Call"(reference=w1949, "Y(mm)"=w1942, "X(mm)"=w1945) -> ()  [unwired: 10 in, 3 out]
              }
            }
            n1230 = property on="currentNO" class="Str"("Val(Sgnl)"="E9") -> ()  [unwired: 2 in, 2 out]
          }
          event "E10": Value Change {
            n1231 = event-data() -> ("NewVal"=w1956:bool)  [unwired: 1 in, 5 out]
            n1232 = property on="移动" class="Bool (严格)"() -> ("Value"=w1957:bool)  [unwired: 2 in, 2 out]
            n1233 = Not(x=w1957) -> (.not. x?=w1958:bool)
            n1234 = And(x=w1958, y=w1956) -> (x .and. y?=w1959:bool)
            n1235 = case shown="真" w1959 {
              frame False {
              }
              frame True {
                n1236 = property on="A1-position-X" class="DigNum (严格)"() -> (error out=w1966:errorcluster, "Value"=w1973:dbl)  [unwired: 2 in, 1 out]
                n1237 = property on="A1-position-Y" class="DigNum (严格)"(error in=w1966) -> (error out=w1965:errorcluster, "Value"=w1962:dbl)  [unwired: 1 in, 1 out]
                n1238 = Subtract(x=w1962, y=18.0) -> (x-y=w1961:dbl)
                n1239 = Subtract(x=w1973, y=40.5) -> (x-y=w1964:dbl)
                n1240 = vi-ref "goto.vi"() -> (w1971:refnum<vi>)
                n1241 = property class="VI"(reference=w1971, error in=w1965) -> ("Name"=w1970:string)  [unwired: 2 out]
                n1242 = Open VI Reference(type specifier VI Refnum (for type only)=refnum<vi> refnum, vi path=w1970, options=128) -> (vi reference=w1968:refnum<vi>)  [unwired: 3 in, 1 out]
                n1243 = call-by-ref "Start Asynchronous Call"(reference=w1968, "Y(mm)"=w1961, "X(mm)"=w1964) -> ()  [unwired: 10 in, 3 out]
              }
            }
            n1244 = property on="currentNO" class="Str"("Val(Sgnl)"="E10") -> ()  [unwired: 2 in, 2 out]
          }
          event "E11": Value Change {
            n1245 = event-data() -> ("NewVal"=w1975:bool)  [unwired: 1 in, 5 out]
            n1246 = property on="移动" class="Bool (严格)"() -> ("Value"=w1978:bool)  [unwired: 2 in, 2 out]
            n1247 = Not(x=w1978) -> (.not. x?=w1977:bool)
            n1248 = And(x=w1977, y=w1975) -> (x .and. y?=w1976:bool)
            n1249 = case shown="真" w1976 {
              frame False {
              }
              frame True {
                n1250 = property on="A1-position-X" class="DigNum (严格)"() -> (error out=w1985:errorcluster, "Value"=w1992:dbl)  [unwired: 2 in, 1 out]
                n1251 = property on="A1-position-Y" class="DigNum (严格)"(error in=w1985) -> (error out=w1984:errorcluster, "Value"=w1981:dbl)  [unwired: 1 in, 1 out]
                n1252 = Subtract(x=w1981, y=18.0) -> (x-y=w1980:dbl)
                n1253 = Subtract(x=w1992, y=45.0) -> (x-y=w1983:dbl)
                n1254 = vi-ref "goto.vi"() -> (w1990:refnum<vi>)
                n1255 = property class="VI"(reference=w1990, error in=w1984) -> ("Name"=w1989:string)  [unwired: 2 out]
                n1256 = Open VI Reference(type specifier VI Refnum (for type only)=refnum<vi> refnum, vi path=w1989, options=128) -> (vi reference=w1987:refnum<vi>)  [unwired: 3 in, 1 out]
                n1257 = call-by-ref "Start Asynchronous Call"(reference=w1987, "Y(mm)"=w1980, "X(mm)"=w1983) -> ()  [unwired: 10 in, 3 out]
              }
            }
            n1258 = property on="currentNO" class="Str"("Val(Sgnl)"="E11") -> ()  [unwired: 2 in, 2 out]
          }
          event "E12": Value Change {
            n1259 = event-data() -> ("NewVal"=w1994:bool)  [unwired: 1 in, 5 out]
            n1260 = property on="移动" class="Bool (严格)"() -> ("Value"=w1997:bool)  [unwired: 2 in, 2 out]
            n1261 = Not(x=w1997) -> (.not. x?=w1996:bool)
            n1262 = And(x=w1996, y=w1994) -> (x .and. y?=w1995:bool)
            n1263 = case shown="真" w1995 {
              frame False {
              }
              frame True {
                n1264 = property on="A1-position-X" class="DigNum (严格)"() -> (error out=w2004:errorcluster, "Value"=w2011:dbl)  [unwired: 2 in, 1 out]
                n1265 = property on="A1-position-Y" class="DigNum (严格)"(error in=w2004) -> (error out=w2003:errorcluster, "Value"=w2000:dbl)  [unwired: 1 in, 1 out]
                n1266 = Subtract(x=w2000, y=18.0) -> (x-y=w1999:dbl)
                n1267 = Subtract(x=w2011, y=49.5) -> (x-y=w2002:dbl)
                n1268 = vi-ref "goto.vi"() -> (w2009:refnum<vi>)
                n1269 = property class="VI"(reference=w2009, error in=w2003) -> ("Name"=w2008:string)  [unwired: 2 out]
                n1270 = Open VI Reference(type specifier VI Refnum (for type only)=refnum<vi> refnum, vi path=w2008, options=128) -> (vi reference=w2006:refnum<vi>)  [unwired: 3 in, 1 out]
                n1271 = call-by-ref "Start Asynchronous Call"(reference=w2006, "Y(mm)"=w1999, "X(mm)"=w2002) -> ()  [unwired: 10 in, 3 out]
              }
            }
            n1272 = property on="currentNO" class="Str"("Val(Sgnl)"="E12") -> ()  [unwired: 2 in, 2 out]
          }
          event "F1": Value Change {
            n1273 = event-data() -> ("NewVal"=w2013:bool)  [unwired: 1 in, 5 out]
            n1274 = property on="移动" class="Bool (严格)"() -> ("Value"=w2016:bool)  [unwired: 2 in, 2 out]
            n1275 = Not(x=w2016) -> (.not. x?=w2015:bool)
            n1276 = And(x=w2015, y=w2013) -> (x .and. y?=w2014:bool)
            n1277 = case shown="真" w2014 {
              frame False {
              }
              frame True {
                n1278 = property on="A1-position-X" class="DigNum (严格)"() -> (error out=w2023:errorcluster, "Value"=w2030:dbl)  [unwired: 2 in, 1 out]
                n1279 = property on="A1-position-Y" class="DigNum (严格)"(error in=w2023) -> (error out=w2022:errorcluster, "Value"=w2019:dbl)  [unwired: 1 in, 1 out]
                n1280 = Subtract(x=w2019, y=22.5) -> (x-y=w2018:dbl)
                n1281 = Subtract(x=w2030, y=0) -> (x-y=w2021:dbl)
                n1282 = vi-ref "goto.vi"() -> (w2028:refnum<vi>)
                n1283 = property class="VI"(reference=w2028, error in=w2022) -> ("Name"=w2027:string)  [unwired: 2 out]
                n1284 = Open VI Reference(type specifier VI Refnum (for type only)=refnum<vi> refnum, vi path=w2027, options=128) -> (vi reference=w2025:refnum<vi>)  [unwired: 3 in, 1 out]
                n1285 = call-by-ref "Start Asynchronous Call"(reference=w2025, "Y(mm)"=w2018, "X(mm)"=w2021) -> ()  [unwired: 10 in, 3 out]
              }
            }
            n1286 = property on="currentNO" class="Str"("Val(Sgnl)"="F1") -> ()  [unwired: 2 in, 2 out]
          }
          event "F2": Value Change {
            n1287 = event-data() -> ("NewVal"=w2032:bool)  [unwired: 1 in, 5 out]
            n1288 = property on="移动" class="Bool (严格)"() -> ("Value"=w2033:bool)  [unwired: 2 in, 2 out]
            n1289 = Not(x=w2033) -> (.not. x?=w2034:bool)
            n1290 = And(x=w2034, y=w2032) -> (x .and. y?=w2035:bool)
            n1291 = case shown="真" w2035 {
              frame False {
              }
              frame True {
                n1292 = property on="A1-position-X" class="DigNum (严格)"() -> (error out=w2042:errorcluster, "Value"=w2049:dbl)  [unwired: 2 in, 1 out]
                n1293 = property on="A1-position-Y" class="DigNum (严格)"(error in=w2042) -> (error out=w2041:errorcluster, "Value"=w2038:dbl)  [unwired: 1 in, 1 out]
                n1294 = Subtract(x=w2038, y=22.5) -> (x-y=w2037:dbl)
                n1295 = Subtract(x=w2049, y=4.5) -> (x-y=w2040:dbl)
                n1296 = vi-ref "goto.vi"() -> (w2047:refnum<vi>)
                n1297 = property class="VI"(reference=w2047, error in=w2041) -> ("Name"=w2046:string)  [unwired: 2 out]
                n1298 = Open VI Reference(type specifier VI Refnum (for type only)=refnum<vi> refnum, vi path=w2046, options=128) -> (vi reference=w2044:refnum<vi>)  [unwired: 3 in, 1 out]
                n1299 = call-by-ref "Start Asynchronous Call"(reference=w2044, "Y(mm)"=w2037, "X(mm)"=w2040) -> ()  [unwired: 10 in, 3 out]
              }
            }
            n1300 = property on="currentNO" class="Str"("Val(Sgnl)"="F2") -> ()  [unwired: 2 in, 2 out]
          }
          event "F3": Value Change {
            n1301 = event-data() -> ("NewVal"=w2051:bool)  [unwired: 1 in, 5 out]
            n1302 = property on="移动" class="Bool (严格)"() -> ("Value"=w2052:bool)  [unwired: 2 in, 2 out]
            n1303 = Not(x=w2052) -> (.not. x?=w2053:bool)
            n1304 = And(x=w2053, y=w2051) -> (x .and. y?=w2054:bool)
            n1305 = case shown="真" w2054 {
              frame False {
              }
              frame True {
                n1306 = property on="A1-position-X" class="DigNum (严格)"() -> (error out=w2061:errorcluster, "Value"=w2068:dbl)  [unwired: 2 in, 1 out]
                n1307 = property on="A1-position-Y" class="DigNum (严格)"(error in=w2061) -> (error out=w2060:errorcluster, "Value"=w2057:dbl)  [unwired: 1 in, 1 out]
                n1308 = Subtract(x=w2057, y=22.5) -> (x-y=w2056:dbl)
                n1309 = Subtract(x=w2068, y=9) -> (x-y=w2059:dbl)
                n1310 = vi-ref "goto.vi"() -> (w2066:refnum<vi>)
                n1311 = property class="VI"(reference=w2066, error in=w2060) -> ("Name"=w2065:string)  [unwired: 2 out]
                n1312 = Open VI Reference(type specifier VI Refnum (for type only)=refnum<vi> refnum, vi path=w2065, options=128) -> (vi reference=w2063:refnum<vi>)  [unwired: 3 in, 1 out]
                n1313 = call-by-ref "Start Asynchronous Call"(reference=w2063, "Y(mm)"=w2056, "X(mm)"=w2059) -> ()  [unwired: 10 in, 3 out]
              }
            }
            n1314 = property on="currentNO" class="Str"("Val(Sgnl)"="F3") -> ()  [unwired: 2 in, 2 out]
          }
          event "F4": Value Change {
            n1315 = event-data() -> ("NewVal"=w2070:bool)  [unwired: 1 in, 5 out]
            n1316 = property on="移动" class="Bool (严格)"() -> ("Value"=w2073:bool)  [unwired: 2 in, 2 out]
            n1317 = Not(x=w2073) -> (.not. x?=w2072:bool)
            n1318 = And(x=w2072, y=w2070) -> (x .and. y?=w2071:bool)
            n1319 = case shown="真" w2071 {
              frame False {
              }
              frame True {
                n1320 = property on="A1-position-X" class="DigNum (严格)"() -> (error out=w2080:errorcluster, "Value"=w2087:dbl)  [unwired: 2 in, 1 out]
                n1321 = property on="A1-position-Y" class="DigNum (严格)"(error in=w2080) -> (error out=w2079:errorcluster, "Value"=w2076:dbl)  [unwired: 1 in, 1 out]
                n1322 = Subtract(x=w2076, y=22.5) -> (x-y=w2075:dbl)
                n1323 = Subtract(x=w2087, y=13.5) -> (x-y=w2078:dbl)
                n1324 = vi-ref "goto.vi"() -> (w2085:refnum<vi>)
                n1325 = property class="VI"(reference=w2085, error in=w2079) -> ("Name"=w2084:string)  [unwired: 2 out]
                n1326 = Open VI Reference(type specifier VI Refnum (for type only)=refnum<vi> refnum, vi path=w2084, options=128) -> (vi reference=w2082:refnum<vi>)  [unwired: 3 in, 1 out]
                n1327 = call-by-ref "Start Asynchronous Call"(reference=w2082, "Y(mm)"=w2075, "X(mm)"=w2078) -> ()  [unwired: 10 in, 3 out]
              }
            }
            n1328 = property on="currentNO" class="Str"("Val(Sgnl)"="F4") -> ()  [unwired: 2 in, 2 out]
          }
          event "F5": Value Change {
            n1329 = event-data() -> ("NewVal"=w2089:bool)  [unwired: 1 in, 5 out]
            n1330 = property on="移动" class="Bool (严格)"() -> ("Value"=w2092:bool)  [unwired: 2 in, 2 out]
            n1331 = Not(x=w2092) -> (.not. x?=w2091:bool)
            n1332 = And(x=w2091, y=w2089) -> (x .and. y?=w2090:bool)
            n1333 = case shown="真" w2090 {
              frame False {
              }
              frame True {
                n1334 = property on="A1-position-X" class="DigNum (严格)"() -> (error out=w2099:errorcluster, "Value"=w2106:dbl)  [unwired: 2 in, 1 out]
                n1335 = property on="A1-position-Y" class="DigNum (严格)"(error in=w2099) -> (error out=w2098:errorcluster, "Value"=w2095:dbl)  [unwired: 1 in, 1 out]
                n1336 = Subtract(x=w2095, y=22.5) -> (x-y=w2094:dbl)
                n1337 = Subtract(x=w2106, y=18.0) -> (x-y=w2097:dbl)
                n1338 = vi-ref "goto.vi"() -> (w2104:refnum<vi>)
                n1339 = property class="VI"(reference=w2104, error in=w2098) -> ("Name"=w2103:string)  [unwired: 2 out]
                n1340 = Open VI Reference(type specifier VI Refnum (for type only)=refnum<vi> refnum, vi path=w2103, options=128) -> (vi reference=w2101:refnum<vi>)  [unwired: 3 in, 1 out]
                n1341 = call-by-ref "Start Asynchronous Call"(reference=w2101, "Y(mm)"=w2094, "X(mm)"=w2097) -> ()  [unwired: 10 in, 3 out]
              }
            }
            n1342 = property on="currentNO" class="Str"("Val(Sgnl)"="F5") -> ()  [unwired: 2 in, 2 out]
          }
          event "F6": Value Change {
            n1343 = event-data() -> ("NewVal"=w2108:bool)  [unwired: 1 in, 5 out]
            n1344 = property on="移动" class="Bool (严格)"() -> ("Value"=w2111:bool)  [unwired: 2 in, 2 out]
            n1345 = Not(x=w2111) -> (.not. x?=w2110:bool)
            n1346 = And(x=w2110, y=w2108) -> (x .and. y?=w2109:bool)
            n1347 = case shown="真" w2109 {
              frame False {
              }
              frame True {
                n1348 = property on="A1-position-X" class="DigNum (严格)"() -> (error out=w2118:errorcluster, "Value"=w2125:dbl)  [unwired: 2 in, 1 out]
                n1349 = property on="A1-position-Y" class="DigNum (严格)"(error in=w2118) -> (error out=w2117:errorcluster, "Value"=w2114:dbl)  [unwired: 1 in, 1 out]
                n1350 = Subtract(x=w2114, y=22.5) -> (x-y=w2113:dbl)
                n1351 = Subtract(x=w2125, y=22.5) -> (x-y=w2116:dbl)
                n1352 = vi-ref "goto.vi"() -> (w2123:refnum<vi>)
                n1353 = property class="VI"(reference=w2123, error in=w2117) -> ("Name"=w2122:string)  [unwired: 2 out]
                n1354 = Open VI Reference(type specifier VI Refnum (for type only)=refnum<vi> refnum, vi path=w2122, options=128) -> (vi reference=w2120:refnum<vi>)  [unwired: 3 in, 1 out]
                n1355 = call-by-ref "Start Asynchronous Call"(reference=w2120, "Y(mm)"=w2113, "X(mm)"=w2116) -> ()  [unwired: 10 in, 3 out]
              }
            }
            n1356 = property on="currentNO" class="Str"("Val(Sgnl)"="F6") -> ()  [unwired: 2 in, 2 out]
          }
          event "F7": Value Change {
            n1357 = event-data() -> ("NewVal"=w2127:bool)  [unwired: 1 in, 5 out]
            n1358 = property on="移动" class="Bool (严格)"() -> ("Value"=w2130:bool)  [unwired: 2 in, 2 out]
            n1359 = Not(x=w2130) -> (.not. x?=w2129:bool)
            n1360 = And(x=w2129, y=w2127) -> (x .and. y?=w2128:bool)
            n1361 = case shown="真" w2128 {
              frame False {
              }
              frame True {
                n1362 = property on="A1-position-X" class="DigNum (严格)"() -> (error out=w2137:errorcluster, "Value"=w2144:dbl)  [unwired: 2 in, 1 out]
                n1363 = property on="A1-position-Y" class="DigNum (严格)"(error in=w2137) -> (error out=w2136:errorcluster, "Value"=w2133:dbl)  [unwired: 1 in, 1 out]
                n1364 = Subtract(x=w2133, y=22.5) -> (x-y=w2132:dbl)
                n1365 = Subtract(x=w2144, y=27) -> (x-y=w2135:dbl)
                n1366 = vi-ref "goto.vi"() -> (w2142:refnum<vi>)
                n1367 = property class="VI"(reference=w2142, error in=w2136) -> ("Name"=w2141:string)  [unwired: 2 out]
                n1368 = Open VI Reference(type specifier VI Refnum (for type only)=refnum<vi> refnum, vi path=w2141, options=128) -> (vi reference=w2139:refnum<vi>)  [unwired: 3 in, 1 out]
                n1369 = call-by-ref "Start Asynchronous Call"(reference=w2139, "Y(mm)"=w2132, "X(mm)"=w2135) -> ()  [unwired: 10 in, 3 out]
              }
            }
            n1370 = property on="currentNO" class="Str"("Val(Sgnl)"="F7") -> ()  [unwired: 2 in, 2 out]
          }
          event "F8": Value Change {
            n1371 = event-data() -> ("NewVal"=w2146:bool)  [unwired: 1 in, 5 out]
            n1372 = property on="移动" class="Bool (严格)"() -> ("Value"=w2149:bool)  [unwired: 2 in, 2 out]
            n1373 = Not(x=w2149) -> (.not. x?=w2148:bool)
            n1374 = And(x=w2148, y=w2146) -> (x .and. y?=w2147:bool)
            n1375 = case shown="真" w2147 {
              frame False {
              }
              frame True {
                n1376 = property on="A1-position-X" class="DigNum (严格)"() -> (error out=w2156:errorcluster, "Value"=w2163:dbl)  [unwired: 2 in, 1 out]
                n1377 = property on="A1-position-Y" class="DigNum (严格)"(error in=w2156) -> (error out=w2155:errorcluster, "Value"=w2152:dbl)  [unwired: 1 in, 1 out]
                n1378 = Subtract(x=w2152, y=22.5) -> (x-y=w2151:dbl)
                n1379 = Subtract(x=w2163, y=31.5) -> (x-y=w2154:dbl)
                n1380 = vi-ref "goto.vi"() -> (w2161:refnum<vi>)
                n1381 = property class="VI"(reference=w2161, error in=w2155) -> ("Name"=w2160:string)  [unwired: 2 out]
                n1382 = Open VI Reference(type specifier VI Refnum (for type only)=refnum<vi> refnum, vi path=w2160, options=128) -> (vi reference=w2158:refnum<vi>)  [unwired: 3 in, 1 out]
                n1383 = call-by-ref "Start Asynchronous Call"(reference=w2158, "Y(mm)"=w2151, "X(mm)"=w2154) -> ()  [unwired: 10 in, 3 out]
              }
            }
            n1384 = property on="currentNO" class="Str"("Val(Sgnl)"="F8") -> ()  [unwired: 2 in, 2 out]
          }
          event "F9": Value Change {
            n1385 = event-data() -> ("NewVal"=w2165:bool)  [unwired: 1 in, 5 out]
            n1386 = property on="移动" class="Bool (严格)"() -> ("Value"=w2168:bool)  [unwired: 2 in, 2 out]
            n1387 = Not(x=w2168) -> (.not. x?=w2167:bool)
            n1388 = And(x=w2167, y=w2165) -> (x .and. y?=w2166:bool)
            n1389 = case shown="真" w2166 {
              frame False {
              }
              frame True {
                n1390 = property on="A1-position-X" class="DigNum (严格)"() -> (error out=w2175:errorcluster, "Value"=w2182:dbl)  [unwired: 2 in, 1 out]
                n1391 = property on="A1-position-Y" class="DigNum (严格)"(error in=w2175) -> (error out=w2174:errorcluster, "Value"=w2171:dbl)  [unwired: 1 in, 1 out]
                n1392 = Subtract(x=w2171, y=22.5) -> (x-y=w2170:dbl)
                n1393 = Subtract(x=w2182, y=36) -> (x-y=w2173:dbl)
                n1394 = vi-ref "goto.vi"() -> (w2180:refnum<vi>)
                n1395 = property class="VI"(reference=w2180, error in=w2174) -> ("Name"=w2179:string)  [unwired: 2 out]
                n1396 = Open VI Reference(type specifier VI Refnum (for type only)=refnum<vi> refnum, vi path=w2179, options=128) -> (vi reference=w2177:refnum<vi>)  [unwired: 3 in, 1 out]
                n1397 = call-by-ref "Start Asynchronous Call"(reference=w2177, "Y(mm)"=w2170, "X(mm)"=w2173) -> ()  [unwired: 10 in, 3 out]
              }
            }
            n1398 = property on="currentNO" class="Str"("Val(Sgnl)"="F9") -> ()  [unwired: 2 in, 2 out]
          }
          event "F10": Value Change {
            n1399 = event-data() -> ("NewVal"=w2184:bool)  [unwired: 1 in, 5 out]
            n1400 = property on="移动" class="Bool (严格)"() -> ("Value"=w2187:bool)  [unwired: 2 in, 2 out]
            n1401 = Not(x=w2187) -> (.not. x?=w2186:bool)
            n1402 = And(x=w2186, y=w2184) -> (x .and. y?=w2185:bool)
            n1403 = case shown="真" w2185 {
              frame False {
              }
              frame True {
                n1404 = property on="A1-position-X" class="DigNum (严格)"() -> (error out=w2194:errorcluster, "Value"=w2201:dbl)  [unwired: 2 in, 1 out]
                n1405 = property on="A1-position-Y" class="DigNum (严格)"(error in=w2194) -> (error out=w2193:errorcluster, "Value"=w2190:dbl)  [unwired: 1 in, 1 out]
                n1406 = Subtract(x=w2190, y=22.5) -> (x-y=w2189:dbl)
                n1407 = Subtract(x=w2201, y=40.5) -> (x-y=w2192:dbl)
                n1408 = vi-ref "goto.vi"() -> (w2199:refnum<vi>)
                n1409 = property class="VI"(reference=w2199, error in=w2193) -> ("Name"=w2198:string)  [unwired: 2 out]
                n1410 = Open VI Reference(type specifier VI Refnum (for type only)=refnum<vi> refnum, vi path=w2198, options=128) -> (vi reference=w2196:refnum<vi>)  [unwired: 3 in, 1 out]
                n1411 = call-by-ref "Start Asynchronous Call"(reference=w2196, "Y(mm)"=w2189, "X(mm)"=w2192) -> ()  [unwired: 10 in, 3 out]
              }
            }
            n1412 = property on="currentNO" class="Str"("Val(Sgnl)"="F10") -> ()  [unwired: 2 in, 2 out]
          }
          event "F11": Value Change {
            n1413 = event-data() -> ("NewVal"=w2203:bool)  [unwired: 1 in, 5 out]
            n1414 = property on="移动" class="Bool (严格)"() -> ("Value"=w2206:bool)  [unwired: 2 in, 2 out]
            n1415 = Not(x=w2206) -> (.not. x?=w2205:bool)
            n1416 = And(x=w2205, y=w2203) -> (x .and. y?=w2204:bool)
            n1417 = case shown="真" w2204 {
              frame False {
              }
              frame True {
                n1418 = property on="A1-position-X" class="DigNum (严格)"() -> (error out=w2213:errorcluster, "Value"=w2220:dbl)  [unwired: 2 in, 1 out]
                n1419 = property on="A1-position-Y" class="DigNum (严格)"(error in=w2213) -> (error out=w2212:errorcluster, "Value"=w2209:dbl)  [unwired: 1 in, 1 out]
                n1420 = Subtract(x=w2209, y=22.5) -> (x-y=w2208:dbl)
                n1421 = Subtract(x=w2220, y=45) -> (x-y=w2211:dbl)
                n1422 = vi-ref "goto.vi"() -> (w2218:refnum<vi>)
                n1423 = property class="VI"(reference=w2218, error in=w2212) -> ("Name"=w2217:string)  [unwired: 2 out]
                n1424 = Open VI Reference(type specifier VI Refnum (for type only)=refnum<vi> refnum, vi path=w2217, options=128) -> (vi reference=w2215:refnum<vi>)  [unwired: 3 in, 1 out]
                n1425 = call-by-ref "Start Asynchronous Call"(reference=w2215, "Y(mm)"=w2208, "X(mm)"=w2211) -> ()  [unwired: 10 in, 3 out]
              }
            }
            n1426 = property on="currentNO" class="Str"("Val(Sgnl)"="F11") -> ()  [unwired: 2 in, 2 out]
          }
          event "F12": Value Change {
            n1427 = event-data() -> ("NewVal"=w2222:bool)  [unwired: 1 in, 5 out]
            n1428 = property on="移动" class="Bool (严格)"() -> ("Value"=w2225:bool)  [unwired: 2 in, 2 out]
            n1429 = Not(x=w2225) -> (.not. x?=w2224:bool)
            n1430 = And(x=w2224, y=w2222) -> (x .and. y?=w2223:bool)
            n1431 = case shown="真" w2223 {
              frame False {
              }
              frame True {
                n1432 = property on="A1-position-X" class="DigNum (严格)"() -> (error out=w2232:errorcluster, "Value"=w2239:dbl)  [unwired: 2 in, 1 out]
                n1433 = property on="A1-position-Y" class="DigNum (严格)"(error in=w2232) -> (error out=w2231:errorcluster, "Value"=w2228:dbl)  [unwired: 1 in, 1 out]
                n1434 = Subtract(x=w2228, y=22.5) -> (x-y=w2227:dbl)
                n1435 = Subtract(x=w2239, y=49.5) -> (x-y=w2230:dbl)
                n1436 = vi-ref "goto.vi"() -> (w2237:refnum<vi>)
                n1437 = property class="VI"(reference=w2237, error in=w2231) -> ("Name"=w2236:string)  [unwired: 2 out]
                n1438 = Open VI Reference(type specifier VI Refnum (for type only)=refnum<vi> refnum, vi path=w2236, options=128) -> (vi reference=w2234:refnum<vi>)  [unwired: 3 in, 1 out]
                n1439 = call-by-ref "Start Asynchronous Call"(reference=w2234, "Y(mm)"=w2227, "X(mm)"=w2230) -> ()  [unwired: 10 in, 3 out]
              }
            }
            n1440 = property on="currentNO" class="Str"("Val(Sgnl)"="F12") -> ()  [unwired: 2 in, 2 out]
          }
          event "G1": Value Change {
            n1441 = event-data() -> ("NewVal"=w2241:bool)  [unwired: 1 in, 5 out]
            n1442 = property on="移动" class="Bool (严格)"() -> ("Value"=w2244:bool)  [unwired: 2 in, 2 out]
            n1443 = Not(x=w2244) -> (.not. x?=w2243:bool)
            n1444 = And(x=w2243, y=w2241) -> (x .and. y?=w2242:bool)
            n1445 = case shown="真" w2242 {
              frame False {
              }
              frame True {
                n1446 = property on="A1-position-X" class="DigNum (严格)"() -> (error out=w2251:errorcluster, "Value"=w2258:dbl)  [unwired: 2 in, 1 out]
                n1447 = property on="A1-position-Y" class="DigNum (严格)"(error in=w2251) -> (error out=w2250:errorcluster, "Value"=w2247:dbl)  [unwired: 1 in, 1 out]
                n1448 = Subtract(x=w2247, y=27.0) -> (x-y=w2246:dbl)
                n1449 = Subtract(x=w2258, y=0) -> (x-y=w2249:dbl)
                n1450 = vi-ref "goto.vi"() -> (w2256:refnum<vi>)
                n1451 = property class="VI"(reference=w2256, error in=w2250) -> ("Name"=w2255:string)  [unwired: 2 out]
                n1452 = Open VI Reference(type specifier VI Refnum (for type only)=refnum<vi> refnum, vi path=w2255, options=128) -> (vi reference=w2253:refnum<vi>)  [unwired: 3 in, 1 out]
                n1453 = call-by-ref "Start Asynchronous Call"(reference=w2253, "Y(mm)"=w2246, "X(mm)"=w2249) -> ()  [unwired: 10 in, 3 out]
              }
            }
            n1454 = property on="currentNO" class="Str"("Val(Sgnl)"="G1") -> ()  [unwired: 2 in, 2 out]
          }
          event "G2": Value Change {
            n1455 = event-data() -> ("NewVal"=w2260:bool)  [unwired: 1 in, 5 out]
            n1456 = property on="移动" class="Bool (严格)"() -> ("Value"=w2263:bool)  [unwired: 2 in, 2 out]
            n1457 = Not(x=w2263) -> (.not. x?=w2262:bool)
            n1458 = And(x=w2262, y=w2260) -> (x .and. y?=w2261:bool)
            n1459 = case shown="真" w2261 {
              frame False {
              }
              frame True {
                n1460 = property on="A1-position-X" class="DigNum (严格)"() -> (error out=w2270:errorcluster, "Value"=w2277:dbl)  [unwired: 2 in, 1 out]
                n1461 = property on="A1-position-Y" class="DigNum (严格)"(error in=w2270) -> (error out=w2269:errorcluster, "Value"=w2266:dbl)  [unwired: 1 in, 1 out]
                n1462 = Subtract(x=w2266, y=27.0) -> (x-y=w2265:dbl)
                n1463 = Subtract(x=w2277, y=4.5) -> (x-y=w2268:dbl)
                n1464 = vi-ref "goto.vi"() -> (w2275:refnum<vi>)
                n1465 = property class="VI"(reference=w2275, error in=w2269) -> ("Name"=w2274:string)  [unwired: 2 out]
                n1466 = Open VI Reference(type specifier VI Refnum (for type only)=refnum<vi> refnum, vi path=w2274, options=128) -> (vi reference=w2272:refnum<vi>)  [unwired: 3 in, 1 out]
                n1467 = call-by-ref "Start Asynchronous Call"(reference=w2272, "Y(mm)"=w2265, "X(mm)"=w2268) -> ()  [unwired: 10 in, 3 out]
              }
            }
            n1468 = property on="currentNO" class="Str"("Val(Sgnl)"="G2") -> ()  [unwired: 2 in, 2 out]
          }
          event "G3": Value Change {
            n1469 = event-data() -> ("NewVal"=w2279:bool)  [unwired: 1 in, 5 out]
            n1470 = property on="移动" class="Bool (严格)"() -> ("Value"=w2282:bool)  [unwired: 2 in, 2 out]
            n1471 = Not(x=w2282) -> (.not. x?=w2281:bool)
            n1472 = And(x=w2281, y=w2279) -> (x .and. y?=w2280:bool)
            n1473 = case shown="真" w2280 {
              frame False {
              }
              frame True {
                n1474 = property on="A1-position-X" class="DigNum (严格)"() -> (error out=w2289:errorcluster, "Value"=w2296:dbl)  [unwired: 2 in, 1 out]
                n1475 = property on="A1-position-Y" class="DigNum (严格)"(error in=w2289) -> (error out=w2288:errorcluster, "Value"=w2285:dbl)  [unwired: 1 in, 1 out]
                n1476 = Subtract(x=w2285, y=27.0) -> (x-y=w2284:dbl)
                n1477 = Subtract(x=w2296, y=9.0) -> (x-y=w2287:dbl)
                n1478 = vi-ref "goto.vi"() -> (w2294:refnum<vi>)
                n1479 = property class="VI"(reference=w2294, error in=w2288) -> ("Name"=w2293:string)  [unwired: 2 out]
                n1480 = Open VI Reference(type specifier VI Refnum (for type only)=refnum<vi> refnum, vi path=w2293, options=128) -> (vi reference=w2291:refnum<vi>)  [unwired: 3 in, 1 out]
                n1481 = call-by-ref "Start Asynchronous Call"(reference=w2291, "Y(mm)"=w2284, "X(mm)"=w2287) -> ()  [unwired: 10 in, 3 out]
              }
            }
            n1482 = property on="currentNO" class="Str"("Val(Sgnl)"="G3") -> ()  [unwired: 2 in, 2 out]
          }
          event "G4": Value Change {
            n1483 = event-data() -> ("NewVal"=w2298:bool)  [unwired: 1 in, 5 out]
            n1484 = property on="移动" class="Bool (严格)"() -> ("Value"=w2301:bool)  [unwired: 2 in, 2 out]
            n1485 = Not(x=w2301) -> (.not. x?=w2300:bool)
            n1486 = And(x=w2300, y=w2298) -> (x .and. y?=w2299:bool)
            n1487 = case shown="真" w2299 {
              frame False {
              }
              frame True {
                n1488 = property on="A1-position-X" class="DigNum (严格)"() -> (error out=w2308:errorcluster, "Value"=w2315:dbl)  [unwired: 2 in, 1 out]
                n1489 = property on="A1-position-Y" class="DigNum (严格)"(error in=w2308) -> (error out=w2307:errorcluster, "Value"=w2304:dbl)  [unwired: 1 in, 1 out]
                n1490 = Subtract(x=w2304, y=27.0) -> (x-y=w2303:dbl)
                n1491 = Subtract(x=w2315, y=13.5) -> (x-y=w2306:dbl)
                n1492 = vi-ref "goto.vi"() -> (w2313:refnum<vi>)
                n1493 = property class="VI"(reference=w2313, error in=w2307) -> ("Name"=w2312:string)  [unwired: 2 out]
                n1494 = Open VI Reference(type specifier VI Refnum (for type only)=refnum<vi> refnum, vi path=w2312, options=128) -> (vi reference=w2310:refnum<vi>)  [unwired: 3 in, 1 out]
                n1495 = call-by-ref "Start Asynchronous Call"(reference=w2310, "Y(mm)"=w2303, "X(mm)"=w2306) -> ()  [unwired: 10 in, 3 out]
              }
            }
            n1496 = property on="currentNO" class="Str"("Val(Sgnl)"="G4") -> ()  [unwired: 2 in, 2 out]
          }
          event "G5": Value Change {
            n1497 = event-data() -> ("NewVal"=w2317:bool)  [unwired: 1 in, 5 out]
            n1498 = property on="移动" class="Bool (严格)"() -> ("Value"=w2320:bool)  [unwired: 2 in, 2 out]
            n1499 = Not(x=w2320) -> (.not. x?=w2319:bool)
            n1500 = And(x=w2319, y=w2317) -> (x .and. y?=w2318:bool)
            n1501 = case shown="真" w2318 {
              frame False {
              }
              frame True {
                n1502 = property on="A1-position-X" class="DigNum (严格)"() -> (error out=w2327:errorcluster, "Value"=w2334:dbl)  [unwired: 2 in, 1 out]
                n1503 = property on="A1-position-Y" class="DigNum (严格)"(error in=w2327) -> (error out=w2326:errorcluster, "Value"=w2323:dbl)  [unwired: 1 in, 1 out]
                n1504 = Subtract(x=w2323, y=27.0) -> (x-y=w2322:dbl)
                n1505 = Subtract(x=w2334, y=18) -> (x-y=w2325:dbl)
                n1506 = vi-ref "goto.vi"() -> (w2332:refnum<vi>)
                n1507 = property class="VI"(reference=w2332, error in=w2326) -> ("Name"=w2331:string)  [unwired: 2 out]
                n1508 = Open VI Reference(type specifier VI Refnum (for type only)=refnum<vi> refnum, vi path=w2331, options=128) -> (vi reference=w2329:refnum<vi>)  [unwired: 3 in, 1 out]
                n1509 = call-by-ref "Start Asynchronous Call"(reference=w2329, "Y(mm)"=w2322, "X(mm)"=w2325) -> ()  [unwired: 10 in, 3 out]
              }
            }
            n1510 = property on="currentNO" class="Str"("Val(Sgnl)"="G5") -> ()  [unwired: 2 in, 2 out]
          }
          event "G6": Value Change {
            n1511 = event-data() -> ("NewVal"=w2336:bool)  [unwired: 1 in, 5 out]
            n1512 = property on="移动" class="Bool (严格)"() -> ("Value"=w2339:bool)  [unwired: 2 in, 2 out]
            n1513 = Not(x=w2339) -> (.not. x?=w2338:bool)
            n1514 = And(x=w2338, y=w2336) -> (x .and. y?=w2337:bool)
            n1515 = case shown="真" w2337 {
              frame False {
              }
              frame True {
                n1516 = property on="A1-position-X" class="DigNum (严格)"() -> (error out=w2346:errorcluster, "Value"=w2353:dbl)  [unwired: 2 in, 1 out]
                n1517 = property on="A1-position-Y" class="DigNum (严格)"(error in=w2346) -> (error out=w2345:errorcluster, "Value"=w2342:dbl)  [unwired: 1 in, 1 out]
                n1518 = Subtract(x=w2342, y=27.0) -> (x-y=w2341:dbl)
                n1519 = Subtract(x=w2353, y=22.5) -> (x-y=w2344:dbl)
                n1520 = vi-ref "goto.vi"() -> (w2351:refnum<vi>)
                n1521 = property class="VI"(reference=w2351, error in=w2345) -> ("Name"=w2350:string)  [unwired: 2 out]
                n1522 = Open VI Reference(type specifier VI Refnum (for type only)=refnum<vi> refnum, vi path=w2350, options=128) -> (vi reference=w2348:refnum<vi>)  [unwired: 3 in, 1 out]
                n1523 = call-by-ref "Start Asynchronous Call"(reference=w2348, "Y(mm)"=w2341, "X(mm)"=w2344) -> ()  [unwired: 10 in, 3 out]
              }
            }
            n1524 = property on="currentNO" class="Str"("Val(Sgnl)"="G6") -> ()  [unwired: 2 in, 2 out]
          }
          event "G7": Value Change {
            n1525 = event-data() -> ("NewVal"=w2355:bool)  [unwired: 1 in, 5 out]
            n1526 = property on="移动" class="Bool (严格)"() -> ("Value"=w2358:bool)  [unwired: 2 in, 2 out]
            n1527 = Not(x=w2358) -> (.not. x?=w2357:bool)
            n1528 = And(x=w2357, y=w2355) -> (x .and. y?=w2356:bool)
            n1529 = case shown="真" w2356 {
              frame False {
              }
              frame True {
                n1530 = property on="A1-position-X" class="DigNum (严格)"() -> (error out=w2365:errorcluster, "Value"=w2372:dbl)  [unwired: 2 in, 1 out]
                n1531 = property on="A1-position-Y" class="DigNum (严格)"(error in=w2365) -> (error out=w2364:errorcluster, "Value"=w2361:dbl)  [unwired: 1 in, 1 out]
                n1532 = Subtract(x=w2361, y=27.0) -> (x-y=w2360:dbl)
                n1533 = Subtract(x=w2372, y=27) -> (x-y=w2363:dbl)
                n1534 = vi-ref "goto.vi"() -> (w2370:refnum<vi>)
                n1535 = property class="VI"(reference=w2370, error in=w2364) -> ("Name"=w2369:string)  [unwired: 2 out]
                n1536 = Open VI Reference(type specifier VI Refnum (for type only)=refnum<vi> refnum, vi path=w2369, options=128) -> (vi reference=w2367:refnum<vi>)  [unwired: 3 in, 1 out]
                n1537 = call-by-ref "Start Asynchronous Call"(reference=w2367, "Y(mm)"=w2360, "X(mm)"=w2363) -> ()  [unwired: 10 in, 3 out]
              }
            }
            n1538 = property on="currentNO" class="Str"("Val(Sgnl)"="G7") -> ()  [unwired: 2 in, 2 out]
          }
          event "G8": Value Change {
            n1539 = event-data() -> ("NewVal"=w2374:bool)  [unwired: 1 in, 5 out]
            n1540 = property on="移动" class="Bool (严格)"() -> ("Value"=w2377:bool)  [unwired: 2 in, 2 out]
            n1541 = Not(x=w2377) -> (.not. x?=w2376:bool)
            n1542 = And(x=w2376, y=w2374) -> (x .and. y?=w2375:bool)
            n1543 = case shown="真" w2375 {
              frame False {
              }
              frame True {
                n1544 = property on="A1-position-X" class="DigNum (严格)"() -> (error out=w2384:errorcluster, "Value"=w2391:dbl)  [unwired: 2 in, 1 out]
                n1545 = property on="A1-position-Y" class="DigNum (严格)"(error in=w2384) -> (error out=w2383:errorcluster, "Value"=w2380:dbl)  [unwired: 1 in, 1 out]
                n1546 = Subtract(x=w2380, y=27.0) -> (x-y=w2379:dbl)
                n1547 = Subtract(x=w2391, y=31.5) -> (x-y=w2382:dbl)
                n1548 = vi-ref "goto.vi"() -> (w2389:refnum<vi>)
                n1549 = property class="VI"(reference=w2389, error in=w2383) -> ("Name"=w2388:string)  [unwired: 2 out]
                n1550 = Open VI Reference(type specifier VI Refnum (for type only)=refnum<vi> refnum, vi path=w2388, options=128) -> (vi reference=w2386:refnum<vi>)  [unwired: 3 in, 1 out]
                n1551 = call-by-ref "Start Asynchronous Call"(reference=w2386, "Y(mm)"=w2379, "X(mm)"=w2382) -> ()  [unwired: 10 in, 3 out]
              }
            }
            n1552 = property on="currentNO" class="Str"("Val(Sgnl)"="G8") -> ()  [unwired: 2 in, 2 out]
          }
          event "G9": Value Change {
            n1553 = event-data() -> ("NewVal"=w2393:bool)  [unwired: 1 in, 5 out]
            n1554 = property on="移动" class="Bool (严格)"() -> ("Value"=w2396:bool)  [unwired: 2 in, 2 out]
            n1555 = Not(x=w2396) -> (.not. x?=w2395:bool)
            n1556 = And(x=w2395, y=w2393) -> (x .and. y?=w2394:bool)
            n1557 = case shown="真" w2394 {
              frame False {
              }
              frame True {
                n1558 = property on="A1-position-X" class="DigNum (严格)"() -> (error out=w2403:errorcluster, "Value"=w2410:dbl)  [unwired: 2 in, 1 out]
                n1559 = property on="A1-position-Y" class="DigNum (严格)"(error in=w2403) -> (error out=w2402:errorcluster, "Value"=w2399:dbl)  [unwired: 1 in, 1 out]
                n1560 = Subtract(x=w2399, y=27.0) -> (x-y=w2398:dbl)
                n1561 = Subtract(x=w2410, y=36.0) -> (x-y=w2401:dbl)
                n1562 = vi-ref "goto.vi"() -> (w2408:refnum<vi>)
                n1563 = property class="VI"(reference=w2408, error in=w2402) -> ("Name"=w2407:string)  [unwired: 2 out]
                n1564 = Open VI Reference(type specifier VI Refnum (for type only)=refnum<vi> refnum, vi path=w2407, options=128) -> (vi reference=w2405:refnum<vi>)  [unwired: 3 in, 1 out]
                n1565 = call-by-ref "Start Asynchronous Call"(reference=w2405, "Y(mm)"=w2398, "X(mm)"=w2401) -> ()  [unwired: 10 in, 3 out]
              }
            }
            n1566 = property on="currentNO" class="Str"("Val(Sgnl)"="G9") -> ()  [unwired: 2 in, 2 out]
          }
          event "G10": Value Change {
            n1567 = event-data() -> ("NewVal"=w2412:bool)  [unwired: 1 in, 5 out]
            n1568 = property on="移动" class="Bool (严格)"() -> ("Value"=w2415:bool)  [unwired: 2 in, 2 out]
            n1569 = Not(x=w2415) -> (.not. x?=w2414:bool)
            n1570 = And(x=w2414, y=w2412) -> (x .and. y?=w2413:bool)
            n1571 = case shown="真" w2413 {
              frame False {
              }
              frame True {
                n1572 = property on="A1-position-X" class="DigNum (严格)"() -> (error out=w2422:errorcluster, "Value"=w2429:dbl)  [unwired: 2 in, 1 out]
                n1573 = property on="A1-position-Y" class="DigNum (严格)"(error in=w2422) -> (error out=w2421:errorcluster, "Value"=w2418:dbl)  [unwired: 1 in, 1 out]
                n1574 = Subtract(x=w2418, y=27.0) -> (x-y=w2417:dbl)
                n1575 = Subtract(x=w2429, y=40.5) -> (x-y=w2420:dbl)
                n1576 = vi-ref "goto.vi"() -> (w2427:refnum<vi>)
                n1577 = property class="VI"(reference=w2427, error in=w2421) -> ("Name"=w2426:string)  [unwired: 2 out]
                n1578 = Open VI Reference(type specifier VI Refnum (for type only)=refnum<vi> refnum, vi path=w2426, options=128) -> (vi reference=w2424:refnum<vi>)  [unwired: 3 in, 1 out]
                n1579 = call-by-ref "Start Asynchronous Call"(reference=w2424, "Y(mm)"=w2417, "X(mm)"=w2420) -> ()  [unwired: 10 in, 3 out]
              }
            }
            n1580 = property on="currentNO" class="Str"("Val(Sgnl)"="G10") -> ()  [unwired: 2 in, 2 out]
          }
          event "G11": Value Change {
            n1581 = event-data() -> ("NewVal"=w2431:bool)  [unwired: 1 in, 5 out]
            n1582 = property on="移动" class="Bool (严格)"() -> ("Value"=w2434:bool)  [unwired: 2 in, 2 out]
            n1583 = Not(x=w2434) -> (.not. x?=w2433:bool)
            n1584 = And(x=w2433, y=w2431) -> (x .and. y?=w2432:bool)
            n1585 = case shown="真" w2432 {
              frame False {
              }
              frame True {
                n1586 = property on="A1-position-X" class="DigNum (严格)"() -> (error out=w2441:errorcluster, "Value"=w2448:dbl)  [unwired: 2 in, 1 out]
                n1587 = property on="A1-position-Y" class="DigNum (严格)"(error in=w2441) -> (error out=w2440:errorcluster, "Value"=w2437:dbl)  [unwired: 1 in, 1 out]
                n1588 = Subtract(x=w2437, y=27.0) -> (x-y=w2436:dbl)
                n1589 = Subtract(x=w2448, y=45) -> (x-y=w2439:dbl)
                n1590 = vi-ref "goto.vi"() -> (w2446:refnum<vi>)
                n1591 = property class="VI"(reference=w2446, error in=w2440) -> ("Name"=w2445:string)  [unwired: 2 out]
                n1592 = Open VI Reference(type specifier VI Refnum (for type only)=refnum<vi> refnum, vi path=w2445, options=128) -> (vi reference=w2443:refnum<vi>)  [unwired: 3 in, 1 out]
                n1593 = call-by-ref "Start Asynchronous Call"(reference=w2443, "Y(mm)"=w2436, "X(mm)"=w2439) -> ()  [unwired: 10 in, 3 out]
              }
            }
            n1594 = property on="currentNO" class="Str"("Val(Sgnl)"="G11") -> ()  [unwired: 2 in, 2 out]
          }
          event "G12": Value Change {
            n1595 = event-data() -> ("NewVal"=w2450:bool)  [unwired: 1 in, 5 out]
            n1596 = property on="移动" class="Bool (严格)"() -> ("Value"=w2453:bool)  [unwired: 2 in, 2 out]
            n1597 = Not(x=w2453) -> (.not. x?=w2452:bool)
            n1598 = And(x=w2452, y=w2450) -> (x .and. y?=w2451:bool)
            n1599 = case shown="真" w2451 {
              frame False {
              }
              frame True {
                n1600 = property on="A1-position-X" class="DigNum (严格)"() -> (error out=w2460:errorcluster, "Value"=w2467:dbl)  [unwired: 2 in, 1 out]
                n1601 = property on="A1-position-Y" class="DigNum (严格)"(error in=w2460) -> (error out=w2459:errorcluster, "Value"=w2456:dbl)  [unwired: 1 in, 1 out]
                n1602 = Subtract(x=w2456, y=27.0) -> (x-y=w2455:dbl)
                n1603 = Subtract(x=w2467, y=49.5) -> (x-y=w2458:dbl)
                n1604 = vi-ref "goto.vi"() -> (w2465:refnum<vi>)
                n1605 = property class="VI"(reference=w2465, error in=w2459) -> ("Name"=w2464:string)  [unwired: 2 out]
                n1606 = Open VI Reference(type specifier VI Refnum (for type only)=refnum<vi> refnum, vi path=w2464, options=128) -> (vi reference=w2462:refnum<vi>)  [unwired: 3 in, 1 out]
                n1607 = call-by-ref "Start Asynchronous Call"(reference=w2462, "Y(mm)"=w2455, "X(mm)"=w2458) -> ()  [unwired: 10 in, 3 out]
              }
            }
            n1608 = property on="currentNO" class="Str"("Val(Sgnl)"="G12") -> ()  [unwired: 2 in, 2 out]
          }
          event "H1": Value Change {
            n1609 = event-data() -> ("NewVal"=w2469:bool)  [unwired: 1 in, 5 out]
            n1610 = property on="移动" class="Bool (严格)"() -> ("Value"=w2472:bool)  [unwired: 2 in, 2 out]
            n1611 = Not(x=w2472) -> (.not. x?=w2471:bool)
            n1612 = And(x=w2471, y=w2469) -> (x .and. y?=w2470:bool)
            n1613 = case shown="真" w2470 {
              frame False {
              }
              frame True {
                n1614 = property on="A1-position-X" class="DigNum (严格)"() -> (error out=w2479:errorcluster, "Value"=w2486:dbl)  [unwired: 2 in, 1 out]
                n1615 = property on="A1-position-Y" class="DigNum (严格)"(error in=w2479) -> (error out=w2478:errorcluster, "Value"=w2475:dbl)  [unwired: 1 in, 1 out]
                n1616 = Subtract(x=w2475, y=31.5) -> (x-y=w2474:dbl)
                n1617 = Subtract(x=w2486, y=0) -> (x-y=w2477:dbl)
                n1618 = vi-ref "goto.vi"() -> (w2484:refnum<vi>)
                n1619 = property class="VI"(reference=w2484, error in=w2478) -> ("Name"=w2483:string)  [unwired: 2 out]
                n1620 = Open VI Reference(type specifier VI Refnum (for type only)=refnum<vi> refnum, vi path=w2483, options=128) -> (vi reference=w2481:refnum<vi>)  [unwired: 3 in, 1 out]
                n1621 = call-by-ref "Start Asynchronous Call"(reference=w2481, "Y(mm)"=w2474, "X(mm)"=w2477) -> ()  [unwired: 10 in, 3 out]
              }
            }
            n1622 = property on="currentNO" class="Str"("Val(Sgnl)"="H1") -> ()  [unwired: 2 in, 2 out]
          }
          event "H2": Value Change {
            n1623 = event-data() -> ("NewVal"=w2488:bool)  [unwired: 1 in, 5 out]
            n1624 = property on="移动" class="Bool (严格)"() -> ("Value"=w2491:bool)  [unwired: 2 in, 2 out]
            n1625 = Not(x=w2491) -> (.not. x?=w2490:bool)
            n1626 = And(x=w2490, y=w2488) -> (x .and. y?=w2489:bool)
            n1627 = case shown="真" w2489 {
              frame False {
              }
              frame True {
                n1628 = property on="A1-position-X" class="DigNum (严格)"() -> (error out=w2498:errorcluster, "Value"=w2505:dbl)  [unwired: 2 in, 1 out]
                n1629 = property on="A1-position-Y" class="DigNum (严格)"(error in=w2498) -> (error out=w2497:errorcluster, "Value"=w2494:dbl)  [unwired: 1 in, 1 out]
                n1630 = Subtract(x=w2494, y=31.5) -> (x-y=w2493:dbl)
                n1631 = Subtract(x=w2505, y=4.5) -> (x-y=w2496:dbl)
                n1632 = vi-ref "goto.vi"() -> (w2503:refnum<vi>)
                n1633 = property class="VI"(reference=w2503, error in=w2497) -> ("Name"=w2502:string)  [unwired: 2 out]
                n1634 = Open VI Reference(type specifier VI Refnum (for type only)=refnum<vi> refnum, vi path=w2502, options=128) -> (vi reference=w2500:refnum<vi>)  [unwired: 3 in, 1 out]
                n1635 = call-by-ref "Start Asynchronous Call"(reference=w2500, "Y(mm)"=w2493, "X(mm)"=w2496) -> ()  [unwired: 10 in, 3 out]
              }
            }
            n1636 = property on="currentNO" class="Str"("Val(Sgnl)"="H2") -> ()  [unwired: 2 in, 2 out]
          }
          event "H3": Value Change {
            n1637 = event-data() -> ("NewVal"=w2507:bool)  [unwired: 1 in, 5 out]
            n1638 = property on="移动" class="Bool (严格)"() -> ("Value"=w2510:bool)  [unwired: 2 in, 2 out]
            n1639 = Not(x=w2510) -> (.not. x?=w2509:bool)
            n1640 = And(x=w2509, y=w2507) -> (x .and. y?=w2508:bool)
            n1641 = case shown="真" w2508 {
              frame False {
              }
              frame True {
                n1642 = property on="A1-position-X" class="DigNum (严格)"() -> (error out=w2517:errorcluster, "Value"=w2524:dbl)  [unwired: 2 in, 1 out]
                n1643 = property on="A1-position-Y" class="DigNum (严格)"(error in=w2517) -> (error out=w2516:errorcluster, "Value"=w2513:dbl)  [unwired: 1 in, 1 out]
                n1644 = Subtract(x=w2513, y=31.5) -> (x-y=w2512:dbl)
                n1645 = Subtract(x=w2524, y=9.0) -> (x-y=w2515:dbl)
                n1646 = vi-ref "goto.vi"() -> (w2522:refnum<vi>)
                n1647 = property class="VI"(reference=w2522, error in=w2516) -> ("Name"=w2521:string)  [unwired: 2 out]
                n1648 = Open VI Reference(type specifier VI Refnum (for type only)=refnum<vi> refnum, vi path=w2521, options=128) -> (vi reference=w2519:refnum<vi>)  [unwired: 3 in, 1 out]
                n1649 = call-by-ref "Start Asynchronous Call"(reference=w2519, "Y(mm)"=w2512, "X(mm)"=w2515) -> ()  [unwired: 10 in, 3 out]
              }
            }
            n1650 = property on="currentNO" class="Str"("Val(Sgnl)"="H3") -> ()  [unwired: 2 in, 2 out]
          }
          event "H4": Value Change {
            n1651 = event-data() -> ("NewVal"=w2526:bool)  [unwired: 1 in, 5 out]
            n1652 = property on="移动" class="Bool (严格)"() -> ("Value"=w2529:bool)  [unwired: 2 in, 2 out]
            n1653 = Not(x=w2529) -> (.not. x?=w2528:bool)
            n1654 = And(x=w2528, y=w2526) -> (x .and. y?=w2527:bool)
            n1655 = case shown="真" w2527 {
              frame False {
              }
              frame True {
                n1656 = property on="A1-position-X" class="DigNum (严格)"() -> (error out=w2536:errorcluster, "Value"=w2543:dbl)  [unwired: 2 in, 1 out]
                n1657 = property on="A1-position-Y" class="DigNum (严格)"(error in=w2536) -> (error out=w2535:errorcluster, "Value"=w2532:dbl)  [unwired: 1 in, 1 out]
                n1658 = Subtract(x=w2532, y=31.5) -> (x-y=w2531:dbl)
                n1659 = Subtract(x=w2543, y=13.5) -> (x-y=w2534:dbl)
                n1660 = vi-ref "goto.vi"() -> (w2541:refnum<vi>)
                n1661 = property class="VI"(reference=w2541, error in=w2535) -> ("Name"=w2540:string)  [unwired: 2 out]
                n1662 = Open VI Reference(type specifier VI Refnum (for type only)=refnum<vi> refnum, vi path=w2540, options=128) -> (vi reference=w2538:refnum<vi>)  [unwired: 3 in, 1 out]
                n1663 = call-by-ref "Start Asynchronous Call"(reference=w2538, "Y(mm)"=w2531, "X(mm)"=w2534) -> ()  [unwired: 10 in, 3 out]
              }
            }
            n1664 = property on="currentNO" class="Str"("Val(Sgnl)"="H4") -> ()  [unwired: 2 in, 2 out]
          }
          event "H5": Value Change {
            n1665 = event-data() -> ("NewVal"=w2545:bool)  [unwired: 1 in, 5 out]
            n1666 = property on="移动" class="Bool (严格)"() -> ("Value"=w2548:bool)  [unwired: 2 in, 2 out]
            n1667 = Not(x=w2548) -> (.not. x?=w2547:bool)
            n1668 = And(x=w2547, y=w2545) -> (x .and. y?=w2546:bool)
            n1669 = case shown="真" w2546 {
              frame False {
              }
              frame True {
                n1670 = property on="A1-position-X" class="DigNum (严格)"() -> (error out=w2555:errorcluster, "Value"=w2562:dbl)  [unwired: 2 in, 1 out]
                n1671 = property on="A1-position-Y" class="DigNum (严格)"(error in=w2555) -> (error out=w2554:errorcluster, "Value"=w2551:dbl)  [unwired: 1 in, 1 out]
                n1672 = Subtract(x=w2551, y=31.5) -> (x-y=w2550:dbl)
                n1673 = Subtract(x=w2562, y=18) -> (x-y=w2553:dbl)
                n1674 = vi-ref "goto.vi"() -> (w2560:refnum<vi>)
                n1675 = property class="VI"(reference=w2560, error in=w2554) -> ("Name"=w2559:string)  [unwired: 2 out]
                n1676 = Open VI Reference(type specifier VI Refnum (for type only)=refnum<vi> refnum, vi path=w2559, options=128) -> (vi reference=w2557:refnum<vi>)  [unwired: 3 in, 1 out]
                n1677 = call-by-ref "Start Asynchronous Call"(reference=w2557, "Y(mm)"=w2550, "X(mm)"=w2553) -> ()  [unwired: 10 in, 3 out]
              }
            }
            n1678 = property on="currentNO" class="Str"("Val(Sgnl)"="H5") -> ()  [unwired: 2 in, 2 out]
          }
          event "H6": Value Change {
            n1679 = event-data() -> ("NewVal"=w2564:bool)  [unwired: 1 in, 5 out]
            n1680 = property on="移动" class="Bool (严格)"() -> ("Value"=w2567:bool)  [unwired: 2 in, 2 out]
            n1681 = Not(x=w2567) -> (.not. x?=w2566:bool)
            n1682 = And(x=w2566, y=w2564) -> (x .and. y?=w2565:bool)
            n1683 = case shown="真" w2565 {
              frame False {
              }
              frame True {
                n1684 = property on="A1-position-X" class="DigNum (严格)"() -> (error out=w2574:errorcluster, "Value"=w2581:dbl)  [unwired: 2 in, 1 out]
                n1685 = property on="A1-position-Y" class="DigNum (严格)"(error in=w2574) -> (error out=w2573:errorcluster, "Value"=w2570:dbl)  [unwired: 1 in, 1 out]
                n1686 = Subtract(x=w2570, y=31.5) -> (x-y=w2569:dbl)
                n1687 = Subtract(x=w2581, y=22.5) -> (x-y=w2572:dbl)
                n1688 = vi-ref "goto.vi"() -> (w2579:refnum<vi>)
                n1689 = property class="VI"(reference=w2579, error in=w2573) -> ("Name"=w2578:string)  [unwired: 2 out]
                n1690 = Open VI Reference(type specifier VI Refnum (for type only)=refnum<vi> refnum, vi path=w2578, options=128) -> (vi reference=w2576:refnum<vi>)  [unwired: 3 in, 1 out]
                n1691 = call-by-ref "Start Asynchronous Call"(reference=w2576, "Y(mm)"=w2569, "X(mm)"=w2572) -> ()  [unwired: 10 in, 3 out]
              }
            }
            n1692 = property on="currentNO" class="Str"("Val(Sgnl)"="H6") -> ()  [unwired: 2 in, 2 out]
          }
          event "H7": Value Change {
            n1693 = event-data() -> ("NewVal"=w2583:bool)  [unwired: 1 in, 5 out]
            n1694 = property on="移动" class="Bool (严格)"() -> ("Value"=w2586:bool)  [unwired: 2 in, 2 out]
            n1695 = Not(x=w2586) -> (.not. x?=w2585:bool)
            n1696 = And(x=w2585, y=w2583) -> (x .and. y?=w2584:bool)
            n1697 = case shown="真" w2584 {
              frame False {
              }
              frame True {
                n1698 = property on="A1-position-X" class="DigNum (严格)"() -> (error out=w2593:errorcluster, "Value"=w2600:dbl)  [unwired: 2 in, 1 out]
                n1699 = property on="A1-position-Y" class="DigNum (严格)"(error in=w2593) -> (error out=w2592:errorcluster, "Value"=w2589:dbl)  [unwired: 1 in, 1 out]
                n1700 = Subtract(x=w2589, y=31.5) -> (x-y=w2588:dbl)
                n1701 = Subtract(x=w2600, y=27) -> (x-y=w2591:dbl)
                n1702 = vi-ref "goto.vi"() -> (w2598:refnum<vi>)
                n1703 = property class="VI"(reference=w2598, error in=w2592) -> ("Name"=w2597:string)  [unwired: 2 out]
                n1704 = Open VI Reference(type specifier VI Refnum (for type only)=refnum<vi> refnum, vi path=w2597, options=128) -> (vi reference=w2595:refnum<vi>)  [unwired: 3 in, 1 out]
                n1705 = call-by-ref "Start Asynchronous Call"(reference=w2595, "Y(mm)"=w2588, "X(mm)"=w2591) -> ()  [unwired: 10 in, 3 out]
              }
            }
            n1706 = property on="currentNO" class="Str"("Val(Sgnl)"="H7") -> ()  [unwired: 2 in, 2 out]
          }
          event "H8": Value Change {
            n1707 = event-data() -> ("NewVal"=w2602:bool)  [unwired: 1 in, 5 out]
            n1708 = property on="移动" class="Bool (严格)"() -> ("Value"=w2605:bool)  [unwired: 2 in, 2 out]
            n1709 = Not(x=w2605) -> (.not. x?=w2604:bool)
            n1710 = And(x=w2604, y=w2602) -> (x .and. y?=w2603:bool)
            n1711 = case shown="真" w2603 {
              frame False {
              }
              frame True {
                n1712 = property on="A1-position-X" class="DigNum (严格)"() -> (error out=w2612:errorcluster, "Value"=w2619:dbl)  [unwired: 2 in, 1 out]
                n1713 = property on="A1-position-Y" class="DigNum (严格)"(error in=w2612) -> (error out=w2611:errorcluster, "Value"=w2608:dbl)  [unwired: 1 in, 1 out]
                n1714 = Subtract(x=w2608, y=31.5) -> (x-y=w2607:dbl)
                n1715 = Subtract(x=w2619, y=31.5) -> (x-y=w2610:dbl)
                n1716 = vi-ref "goto.vi"() -> (w2617:refnum<vi>)
                n1717 = property class="VI"(reference=w2617, error in=w2611) -> ("Name"=w2616:string)  [unwired: 2 out]
                n1718 = Open VI Reference(type specifier VI Refnum (for type only)=refnum<vi> refnum, vi path=w2616, options=128) -> (vi reference=w2614:refnum<vi>)  [unwired: 3 in, 1 out]
                n1719 = call-by-ref "Start Asynchronous Call"(reference=w2614, "Y(mm)"=w2607, "X(mm)"=w2610) -> ()  [unwired: 10 in, 3 out]
              }
            }
            n1720 = property on="currentNO" class="Str"("Val(Sgnl)"="H8") -> ()  [unwired: 2 in, 2 out]
          }
          event "H9": Value Change {
            n1721 = event-data() -> ("NewVal"=w2621:bool)  [unwired: 1 in, 5 out]
            n1722 = property on="移动" class="Bool (严格)"() -> ("Value"=w2624:bool)  [unwired: 2 in, 2 out]
            n1723 = Not(x=w2624) -> (.not. x?=w2623:bool)
            n1724 = And(x=w2623, y=w2621) -> (x .and. y?=w2622:bool)
            n1725 = case shown="真" w2622 {
              frame False {
              }
              frame True {
                n1726 = property on="A1-position-X" class="DigNum (严格)"() -> (error out=w2631:errorcluster, "Value"=w2638:dbl)  [unwired: 2 in, 1 out]
                n1727 = property on="A1-position-Y" class="DigNum (严格)"(error in=w2631) -> (error out=w2630:errorcluster, "Value"=w2627:dbl)  [unwired: 1 in, 1 out]
                n1728 = Subtract(x=w2627, y=31.5) -> (x-y=w2626:dbl)
                n1729 = Subtract(x=w2638, y=36) -> (x-y=w2629:dbl)
                n1730 = vi-ref "goto.vi"() -> (w2636:refnum<vi>)
                n1731 = property class="VI"(reference=w2636, error in=w2630) -> ("Name"=w2635:string)  [unwired: 2 out]
                n1732 = Open VI Reference(type specifier VI Refnum (for type only)=refnum<vi> refnum, vi path=w2635, options=128) -> (vi reference=w2633:refnum<vi>)  [unwired: 3 in, 1 out]
                n1733 = call-by-ref "Start Asynchronous Call"(reference=w2633, "Y(mm)"=w2626, "X(mm)"=w2629) -> ()  [unwired: 10 in, 3 out]
              }
            }
            n1734 = property on="currentNO" class="Str"("Val(Sgnl)"="H9") -> ()  [unwired: 2 in, 2 out]
          }
          event "H10": Value Change {
            n1735 = event-data() -> ("NewVal"=w2640:bool)  [unwired: 1 in, 5 out]
            n1736 = property on="移动" class="Bool (严格)"() -> ("Value"=w2643:bool)  [unwired: 2 in, 2 out]
            n1737 = Not(x=w2643) -> (.not. x?=w2642:bool)
            n1738 = And(x=w2642, y=w2640) -> (x .and. y?=w2641:bool)
            n1739 = case shown="真" w2641 {
              frame False {
              }
              frame True {
                n1740 = property on="A1-position-X" class="DigNum (严格)"() -> (error out=w2650:errorcluster, "Value"=w2657:dbl)  [unwired: 2 in, 1 out]
                n1741 = property on="A1-position-Y" class="DigNum (严格)"(error in=w2650) -> (error out=w2649:errorcluster, "Value"=w2646:dbl)  [unwired: 1 in, 1 out]
                n1742 = Subtract(x=w2646, y=31.5) -> (x-y=w2645:dbl)
                n1743 = Subtract(x=w2657, y=40.5) -> (x-y=w2648:dbl)
                n1744 = vi-ref "goto.vi"() -> (w2655:refnum<vi>)
                n1745 = property class="VI"(reference=w2655, error in=w2649) -> ("Name"=w2654:string)  [unwired: 2 out]
                n1746 = Open VI Reference(type specifier VI Refnum (for type only)=refnum<vi> refnum, vi path=w2654, options=128) -> (vi reference=w2652:refnum<vi>)  [unwired: 3 in, 1 out]
                n1747 = call-by-ref "Start Asynchronous Call"(reference=w2652, "Y(mm)"=w2645, "X(mm)"=w2648) -> ()  [unwired: 10 in, 3 out]
              }
            }
            n1748 = property on="currentNO" class="Str"("Val(Sgnl)"="H10") -> ()  [unwired: 2 in, 2 out]
          }
          event "H11": Value Change {
            n1749 = event-data() -> ("NewVal"=w2659:bool)  [unwired: 1 in, 5 out]
            n1750 = property on="移动" class="Bool (严格)"() -> ("Value"=w2662:bool)  [unwired: 2 in, 2 out]
            n1751 = Not(x=w2662) -> (.not. x?=w2661:bool)
            n1752 = And(x=w2661, y=w2659) -> (x .and. y?=w2660:bool)
            n1753 = case shown="真" w2660 {
              frame False {
              }
              frame True {
                n1754 = property on="A1-position-X" class="DigNum (严格)"() -> (error out=w2669:errorcluster, "Value"=w2676:dbl)  [unwired: 2 in, 1 out]
                n1755 = property on="A1-position-Y" class="DigNum (严格)"(error in=w2669) -> (error out=w2668:errorcluster, "Value"=w2665:dbl)  [unwired: 1 in, 1 out]
                n1756 = Subtract(x=w2665, y=31.5) -> (x-y=w2664:dbl)
                n1757 = Subtract(x=w2676, y=45) -> (x-y=w2667:dbl)
                n1758 = vi-ref "goto.vi"() -> (w2674:refnum<vi>)
                n1759 = property class="VI"(reference=w2674, error in=w2668) -> ("Name"=w2673:string)  [unwired: 2 out]
                n1760 = Open VI Reference(type specifier VI Refnum (for type only)=refnum<vi> refnum, vi path=w2673, options=128) -> (vi reference=w2671:refnum<vi>)  [unwired: 3 in, 1 out]
                n1761 = call-by-ref "Start Asynchronous Call"(reference=w2671, "Y(mm)"=w2664, "X(mm)"=w2667) -> ()  [unwired: 10 in, 3 out]
              }
            }
            n1762 = property on="currentNO" class="Str"("Val(Sgnl)"="H11") -> ()  [unwired: 2 in, 2 out]
          }
          event "H12": Value Change {
            n1763 = event-data() -> ("NewVal"=w2678:bool)  [unwired: 1 in, 5 out]
            n1764 = property on="移动" class="Bool (严格)"() -> ("Value"=w2681:bool)  [unwired: 2 in, 2 out]
            n1765 = Not(x=w2681) -> (.not. x?=w2680:bool)
            n1766 = And(x=w2680, y=w2678) -> (x .and. y?=w2679:bool)
            n1767 = case shown="真" w2679 {
              frame False {
              }
              frame True {
                n1768 = property on="A1-position-X" class="DigNum (严格)"() -> (error out=w2688:errorcluster, "Value"=w2695:dbl)  [unwired: 2 in, 1 out]
                n1769 = property on="A1-position-Y" class="DigNum (严格)"(error in=w2688) -> (error out=w2687:errorcluster, "Value"=w2684:dbl)  [unwired: 1 in, 1 out]
                n1770 = Subtract(x=w2684, y=31.5) -> (x-y=w2683:dbl)
                n1771 = Subtract(x=w2695, y=49.5) -> (x-y=w2686:dbl)
                n1772 = vi-ref "goto.vi"() -> (w2693:refnum<vi>)
                n1773 = property class="VI"(reference=w2693, error in=w2687) -> ("Name"=w2692:string)  [unwired: 2 out]
                n1774 = Open VI Reference(type specifier VI Refnum (for type only)=refnum<vi> refnum, vi path=w2692, options=128) -> (vi reference=w2690:refnum<vi>)  [unwired: 3 in, 1 out]
                n1775 = call-by-ref "Start Asynchronous Call"(reference=w2690, "Y(mm)"=w2683, "X(mm)"=w2686) -> ()  [unwired: 10 in, 3 out]
              }
            }
            n1776 = property on="currentNO" class="Str"("Val(Sgnl)"="H12") -> ()  [unwired: 2 in, 2 out]
          }
          event "ShutDownSystem": Value Change {
            n1777 = event-data() -> ("NewVal"=w2698:bool)  [unwired: 1 in, 5 out]
            n1778 = case shown="真" w2698 {
              tunnel: w2697 -> [_ _]
              frame False {
              }
              frame True {
                n1779 = flat-sequence {
                  frame #0 {
                    n1780 = call "stop_device.vi"() -> ()  [unwired: 11 in, 1 out]
                  }
                  frame #1 {
                    n1781 = property on="stop" class="Bool (严格)"("Value"=TRUE ("stop")) -> ()  [unwired: 2 in, 2 out]
                  }
                }
              }
            }
          }
        }
        n1782 = property on="stop" class="Bool (严格)"() -> ("Value"=w252:bool)  [unwired: 2 in, 2 out]
      }
      n1783 = while {
        tunnel: w146 -> [w152]
        stop <- w151 stop-if-true
        n1784 = event shown="[4] \"currentNO\": 值改变" {
          selector: w152 -> [_ _ _ _ _]
          dyn-events: _ -> [_ _ _ _ _]
          timeout: _ -> [_ _ _ _ _]
          event Timeout {
            n1785 = event-data() -> ()  [unwired: 1 in, 3 out]
          }
          event User Event {
            n1786 = event-data() -> ("AI"=w154:dbl[], "DI"=w153:bool[])  [unwired: 1 in, 4 out]
            n1787 = Index Array(array=w154, index=0) -> (element=w172:dbl)
            n1788 = Index Array(array=w153, index=0) -> (element=→"X0":bool)
            n1789 = Divide(x=w172, y=10.0) -> (x/y=w174:dbl)
            n1790 = Multiply(x=w174, y=2000.0) -> (x*y=w176:dbl)
            n1791 = property on="MCPHV-Real" class="DigNum (严格)"("Value"=w176) -> (error out=w155:errorcluster)  [unwired: 2 in, 1 out]
            n1792 = Index Array(array=w153, index=4) -> (element=→"Y0":bool)
            n1793 = Index Array(array=w154, index=1) -> (element=w177:dbl)
            n1794 = Divide(x=w177, y=10.0) -> (x/y=w179:dbl)
            n1795 = Multiply(x=w179, y=20000.0) -> (x*y=w181:dbl)
            n1796 = Index Array(array=w153, index=1) -> (element=→"X满":bool)
            n1797 = property on="Tar.HV-Real" class="DigNum (严格)"(error in=w155, "Value"=w181) -> (error out=w156:errorcluster)  [unwired: 1 in, 1 out]
            n1798 = Index Array(array=w154, index=2) -> (element=w182:dbl)
            n1799 = Index Array(array=w153, index=3) -> (element=→"Y标":bool)
            n1800 = Divide(x=w182, y=10.0) -> (x/y=w184:dbl)
            n1801 = Multiply(x=w184, y=2000.0) -> (x*y=w186:dbl)
            n1802 = property on="Pul.HV-Real" class="DigNum (严格)"(error in=w156, "Value"=w186) -> (error out=w157:errorcluster)  [unwired: 1 in, 1 out]
            n1803 = Index Array(array=w154, index=3) -> (element=w187:dbl)
            n1804 = Index Array(array=w153, index=2) -> (element=→"Y满":bool)
            n1805 = Divide(x=w187, y=10.0) -> (x/y=w189:dbl)
            n1806 = Multiply(x=w189, y=10000.0) -> (x*y=w191:dbl)
            n1807 = property on="LensHV-Real" class="DigNum (严格)"(error in=w157, "Value"=w191) -> (error out=w193:errorcluster)  [unwired: 1 in, 1 out]
            n1808 = Index Array(array=w154, index=19) -> (element=w195:dbl)
            n1809 = Subtract(x=w195, y=3.572) -> (x-y=w197:dbl)
            n1810 = Divide(x=w197, y=1.286) -> (x/y=w199:dbl)
            n1811 = Power Of 10(x=w199) -> (10^x=w200:dbl)
            n1812 = Index Array(array=w154, index=18) -> (element=w201:dbl)
            n1813 = Subtract(x=w201, y=8.5) -> (x-y=w203:dbl)
            n1814 = property on="Lvaccum" class="DigNum (严格)"(error in=w193, "Value"=w200) -> (error out=w205:errorcluster)  [unwired: 1 in, 1 out]
            n1815 = Power Of 10(x=w203) -> (10^x=w204:dbl)
            n1816 = property on="Hvaccum" class="DigNum (严格)"(error in=w205, "Value"=w204) -> ()  [unwired: 1 in, 2 out]
          }
          event User Event {
            n1817 = event-data() -> ("status"=w206:string)  [unwired: 1 in, 5 out]
            n1818 = case shown="\"stop\", 默认" w206 {
              frame "stop", Default {
                n1819 = property on="GO" class="Bool (严格)"("DisabledEnum"=T11."Enabled" ("Disabled")) -> (error out=w208:errorcluster)  [unwired: 2 in, 1 out]
                n1820 = property on="移动" class="Bool (严格)"(error in=w208, "Value"=FALSE ("移动")) -> ()  [unwired: 1 in, 2 out]
              }
              frame "moving" {
                n1821 = property on="GO" class="Bool (严格)"("DisabledEnum"=T11."Disabled and Grayed Out" ("Disabled")) -> (error out=w211:errorcluster)  [unwired: 2 in, 1 out]
                n1822 = property on="移动" class="Bool (严格)"(error in=w211, "Value"=TRUE ("移动")) -> ()  [unwired: 1 in, 2 out]
              }
            }
          }
          event User Event {
            n1823 = event-data() -> ("source"=w213:string, "value"=w214:dbl)  [unwired: 1 in, 4 out]
            n1824 = case shown="\"X\"" w213 {
              tunnel: w214 -> [w221 w229]
              tunnel: [w223 w230] -> w220
              frame "Y", Default {
                n1825 = property on="X当前" class="DigNum (严格)"() -> ("Value"=w225:dbl)  [unwired: 2 in, 2 out]
                n1826 = Multiply(x=w221, y=1000.0) -> (x*y=w226:dbl)
                n1827 = Divide(x=w225, y=1000.0) -> (x/y=w222:dbl)
                n1828 = Build Array "Build Array"(w222, w221) -> (w223:dbl[])
                n1829 = property on="Y当前" class="DigNum (严格)"("Value"=w226) -> ()  [unwired: 2 in, 2 out]
              }
              frame "X" {
                n1830 = property on="Y当前" class="DigNum (严格)"() -> ("Value"=w232:dbl)  [unwired: 2 in, 2 out]
                n1831 = Multiply(x=w229, y=1000.0) -> (x*y=w233:dbl)
                n1832 = Divide(x=w232, y=1000.0) -> (x/y=w228:dbl)
                n1833 = property on="X当前" class="DigNum (严格)"("Value"=w233) -> ()  [unwired: 2 in, 2 out]
                n1834 = Build Array(w229, w228) -> (w230:dbl[])
              }
            }
            n1835 = Current VI's Path() -> (path=w217:path)
            n1836 = Strip Path(path=w217) -> (stripped path=w218:path)  [unwired: 1 out]
            n1837 = Build Path(base path=w218, name or relative path="last_position") -> (appended path=w216:path)
            n1838 = call-poly <vilib>:"Write To Spreadsheet File.vi"("format (%.3f)"="%.9f", "1D data"=w220, "file path (dialog if empty)"=w216) -> ()  [unwired: 5 in, 1 out]
          }
          event "currentNO": Value Change {
            n1839 = event-data() -> ("NewVal"=w238:string)  [unwired: 1 in, 5 out]
            n1840 = control-ref of="本VI"() -> (w248:refnum<vi>)
            n1841 = property on="targetMark" class="Str"() -> (error out=w235:errorcluster, "Value"=w251:string)  [unwired: 2 in, 1 out]
            n1842 = call "index_ctl.vi"("错误输入（无错误）"=w235, "lable"=w251, "VI refence"=w248) -> ("error out"=w245:errorcluster, "Ctl refence"=w250:refnum<vi>)  [unwired: 7 in]
            n1843 = property class="Ctl"(reference=w250, error in=w245, "Value"=FALSE) -> (error out=w244:errorcluster)  [unwired: 1 out]
            n1844 = call "index_ctl.vi"("错误输入（无错误）"=w244, "lable"=w238, "VI refence"=w248) -> ("error out"=w243:errorcluster, "Ctl refence"=w247:refnum<vi>)  [unwired: 7 in]
            n1845 = property class="Ctl"(reference=w247, error in=w243, "Value"=TRUE) -> (error out=w242:errorcluster)  [unwired: 1 out]
            n1846 = property on="targetMark" class="Str"(error in=w242, "Value"=w238) -> (error out=w237:errorcluster)  [unwired: 1 in, 1 out]
            n1847 = property on="config" class="TypRef (严格)"(error in=w237) -> (error out=w236:errorcluster, "Value"=w241:T1)  [unwired: 1 in, 1 out]
            n1848 = call-poly <vilib>:"Write Key.vi"("section"="plat", "error in (no error)"=w236, "value"=w238, "key"="num", "refnum"=w241) -> ()  [unwired: 4 in, 3 out]
          }
        }
        n1849 = property on="stop" class="Bool (严格)"() -> ("Value"=w151:bool)  [unwired: 2 in, 2 out]
      }
    }
    frame #2 {
      n1850 = property on="config" class="TypRef (严格)"() -> ("Value"=w2700:T1)  [unwired: 2 in, 2 out]
      n1851 = call <vilib>:"Close Config Data.vi"("refnum"=w2700) -> ()  [unwired: 9 in, 2 out]
    }
  }
  n1852 = Unbundle(w28) -> ("tasks"=w9:T14, "interface"=w8:T13, "error out"=w7:errorcluster)
  n1853 = call "USB6343_Control_v1.6.2.vi"("error in"=w7, "interface"=w8, "tasks"=w9) -> ()  [unwired: 9 in]
  n1854 = call <vilib>:"IMAQdx Enumerate Cameras.vi"() -> ("error out"=w18:errorcluster, "Camera Information Array"=w15:T19)  [unwired: 10 in]
  n1855 = while {
    tunnel: w30 -> [w2728]
    tunnel: w29 -> [w2701]
    tunnel: [w2702] -> w5
    tunnel: [w2701] -> w4
    stop <- w2703 stop-if-true
    n1856 = Unbundle By Name(w2728) -> ("pump semaphore"=w2727:T4, "laser semaphore"=w2724:T4)
    n1857 = Unbundle By Name(w2701) -> ("ConfiguredPumpCom"=w2726:refnum<visa-resource-name>, "ConfiguredLaserCom"=w2715:refnum<visa-resource-name>)
    n1858 = call <vilib>:"Acquire Semaphore.vi"("semaphore"=w2727) -> ("error out"=w2714:errorcluster, "semaphore out"=w2725:T4)  [unwired: 4 in, 1 out]
    n1859 = call "pumpStatus.vi"("VISA resource name"=w2726, "error in (no error)"=w2714) -> ("PumpKW"=→"PumpKW":dbl, "PumpTemp"=→"PumpTemp":u16, "PumpAmps"=→"PumpAmps":dbl, "PumpVolts"=→"PumpVolts":dbl, "TurboSpeed"=→"TurboSpeed":dbl, "error out"=w2713:errorcluster)  [unwired: 8 in]
    n1860 = call <vilib>:"Release Semaphore.vi"("error in (no error)"=w2713, "semaphore"=w2725) -> ("error out"=w2711:errorcluster)  [unwired: 4 in, 1 out]
    n1861 = call <vilib>:"Acquire Semaphore.vi"("error in (no error)"=w2711, "semaphore"=w2724) -> ("error out"=w2712:errorcluster, "semaphore out"=w2710:T4)  [unwired: 3 in, 1 out]
    n1862 = call "Laser-Get-Shotstatus.vi"("VISA resource name"=w2715, "error in (no error)"=w2712) -> ("VISA resource name out"=w2708:refnum<visa-resource-name>, "cluster"=→"cluster":T8, "error out"=w2706:errorcluster)
    n1863 = property on="SetLaserTransmission" class="Slide (严格)"(error in=w2706) -> (error out=w2705:errorcluster, "Value"=w2704:dbl)  [unwired: 1 in, 1 out]
    n1864 = call "Laser-Read-Energy.vi"("Transimission"=w2704, "error in (no error)"=w2705, "VISA resource name"=w2708) -> ("LaserEnergy uJ"=→"LaserEnergy uJ 2":dbl, "error out"=w2709:errorcluster)  [unwired: 1 out]
    n1865 = call <vilib>:"Release Semaphore.vi"("error in (no error)"=w2709, "semaphore"=w2710) -> ("error out"=w2723:errorcluster)  [unwired: 4 in, 1 out]
    n1866 = property on="stop" class="Bool (严格)"() -> ("Value"=w2703:bool)  [unwired: 2 in, 2 out]
    n1867 = call "Time Delay2"("error in (no error)"=w2723, "Delay Time (s)"=0.3) -> ("error out"=w2702:errorcluster)  [unwired: 9 in]
  }
  n1868 = Index Array(array=w15, index=0) -> (element=w17:T20)
  n1869 = Unbundle By Name(w17) -> ("InterfaceName"=w25:string)
  n1870 = call <vilib>:"IMAQdx Open Camera.vi"("error in"=w18, "Session In"=w25) -> ("error out"=w12:errorcluster, "Session Out"=w13:T21)  [unwired: 8 in]
  n1871 = property class="IMAQdx" props=["VideoMode", "Width", "Height"](reference=w13, error in=w12, "VideoMode"=u32 13) -> (reference out=w11:T21, error out=w10:errorcluster)  [unwired: 2 out]
  n1872 = call "IMAQ Create"("Image Name"=w25) -> ("New Image"=w20:T3)  [unwired: 4 in, 1 out]
  n1873 = call <vilib>:"IMAQdx Configure Grab.vi"("error in"=w10, "Session In"=w11) -> ("error out"=w24:errorcluster, "Session Out"=w19:T21)  [unwired: 8 in]
  n1874 = while {
    tunnel: w24 -> [w2735]
    tunnel: w19 -> [w2734]
    tunnel: w20 -> [w2733]
    tunnel: [w2732] -> w21
    tunnel: [w2731] -> w22
    tunnel: [w2730] -> w23
    stop <- w2729 stop-if-true
    n1875 = call <vilib>:"IMAQdx Grab.vi"("error in"=w2735, "Image In"=w2733, "Session In"=w2734) -> ("error out"=w2732:errorcluster, "Image Out"=w2730:T3, "Session Out"=w2731:T21)  [unwired: 5 in, 1 out]
    "Image" <- w2730
    n1876 = property on="stop" class="Bool (严格)"() -> ("Value"=w2729:bool)  [unwired: 2 in, 2 out]
  }
  n1877 = call "IMAQ Dispose"("Image"=w23) -> ()  [unwired: 5 in, 1 out]
  n1878 = call <vilib>:"IMAQdx Close Camera.vi"("error in"=w21, "Session In"=w22) -> ()  [unwired: 9 in, 1 out]
  n1879 = Unbundle By Name(w4) -> ("ConfiguredPumpCom"=w3:refnum<visa-resource-name>, "ConfiguredLaserCom"=w1:refnum<visa-resource-name>)
  n1880 = VISA Close(VISA resource name=w3, error in (no error)=w5) -> (error out=w2:errorcluster)
  n1881 = VISA Close(VISA resource name=w1, error in (no error)=w2) -> ()  [unwired: 1 out]
